vi "Loop_Auto.vi"() -> ()   [LabVIEW 2017, in "Autonomous.lvlib"]
uses:
  Autonomous.lvlib
  ENUM_Auto_State.ctl
  TypeDef/CLUSTER_CMD_WC_Drive.ctl
  TypeDef/ENUM_WC_Drive_DriveMode.ctl
  TypeDef/CLUSTER_Drive_ACT Loop_VBus Data.ctl
  TypeDef/CLUSTER_X and Y.ctl
  TypeDef/CLUSTER_Drive_ACT Loop_Profile Data.ctl
  ENUM_Auto_AutoMode.ctl
  TypeDef/CLUSTER_AUTO_switchBools.ctl
  Rotation_Overloard/CLUSTER_Rotation_CMD.ctl
  Rotation_Overloard/ENUM_Rotation_Positon.ctl
  <vilib>/Rock Robotics/WPI/ThirdParty/Sensors/navX/_TypeDefs/FRIC_navX_DeviceNumbersTypeDef.ctl
  ENUM_Auto_Action.ctl
  _SHARE ALL/Global Share All/Global_STOP.vi
  Globals/Global_Drive_Encoders.vi
  Rotation_Overloard/Global_CMD.vi
  Rotation_Overloard/Global_SM_Output.vi
  <vilib>/addons/control/pid/pid.llb/PID (DBL).vi
  Globals/Global_CMD_Drive.vi
  Rotation_Overloard/Rotation_Overlord.lvlib
  <vilib>/addons/control/pid/NI_PID_pid.lvlib
panel:
  in  "Enum":enum16{"LRL", "RLR", "RRR", "LLL"}(ring)
  out "Yaw":dbl
  out "Cycle Time (S)":dbl format="%.3g"
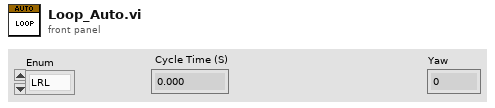
[diagram p1: front panel]
types:
  T1 = typedef "Rotation_Overlord.lvlib/ENUM_Rotation_Positon.ctl" = enum16{"Neutral", "Pickup", "Switch", "Scale", "Climb", "Manual"}
  T2 = typedef "Rotation_Overlord.lvlib/CLUSTER_Rotation_CMD.ctl" = cluster{"Rotation Positon":T1, "Enable Rotation":bool, "Manual Override":bool, "Arm Value":dbl, "Claw Rotation Value":dbl, "Lift Value":dbl}
  T3 = typedef "CLUSTER_AUTO_switchBools.ctl" = cluster{"First Drive":bool, "Rotated ":bool, "Second Move":bool, "Arm In position":bool, "Cube released":bool}
  T4 = typedef "ENUM_Auto_AutoMode.ctl" = enum16{"No Movement", "Scale And Switch", "Switch", "Scale", "Cross Line"}
  T5 = typedef "CLUSTER_CMD_WC_Drive.ctl" = cluster{"Drive_Mode":T6, "VBus":T7, "Profile":T9, "Zero Drive Encoders":bool, "Set Target Position(IN)":dbl, "Target Angle(Degree)":dbl, "Lock Angle":bool, "Zero YAW":bool, "Follow Cubes":bool, "Follow Road":bool, "Anti-Turbo":bool}
  T6 = typedef "ENUM_WC_Drive_DriveMode.ctl" = enum16{"Motion Profile", "CrossLineAuto", "VBus", "Stop"}
  T7 = typedef "CLUSTER_Drive_ACT Loop_VBus Data.ctl" = cluster{"Drive":T8, "Turbo":bool}
  T8 = typedef "CLUSTER_X and Y.ctl" = cluster{"Steer":dbl, "Throtle":dbl}
  T9 = typedef "CLUSTER_Drive_ACT Loop_Profile Data.ctl" = cluster{"Start":bool}
  T10 = typedef "Autonomous.lvlib/ENUM_Auto_State.ctl" = enum16{"Startup", "Idle", "position claw arm lift", "Intake", "Rotate To Angle", "Cross Line", "Shutdown"}
  T11 = typedef "Autonomous.lvlib/ENUM_Auto_Action.ctl" = enum16{"No Action", "Reset Time", "Reset All", "Lock Angle", "Drive", "Zero Drive Encoders", "Zero YAW"}
  T12 = cluster{"State":T10, "Previous State":T10, "Current Time":timestamp, "Previous Time":timestamp, "Start Time":timestamp, "Target Time (ms)":u32, "Cycle Time(S)":dbl, "CMD_Drive_Data":T5, "Test":dbl, "Steering":dbl, "Throtal":dbl, "Encoder Target Position(in)":dbl, "Zero Drive Encoders":bool, "Lock Angle":bool, "Target Angle(Degree)":dbl, "Zero YAW":bool, "Left Encoder":i32, "Right Encoder":i32, "YAW":dbl, "AutoMode":T4, "Switch Booleans":T3, "CMD_SM_Rotation":T2, "SM_Rotation_Output":T1}
  T13 = typedef "FRIC_navX_DeviceNumbersTypeDef.ctl" = enum16{"Dev0", "Dev1", "Dev2", "Dev3"}
  T14 = cluster{"proportional gain (Kc)":dbl, "integral time (Ti, min)":dbl, "derivative time (Td, min)":dbl}
  T15 = cluster{"Left_Drive_Encoder":i32, "Right_Drive_Encoder":i32}
  T16 = cluster{"Rollover":dbl, "Yaw":dbl, "Cont Yaw":dbl}
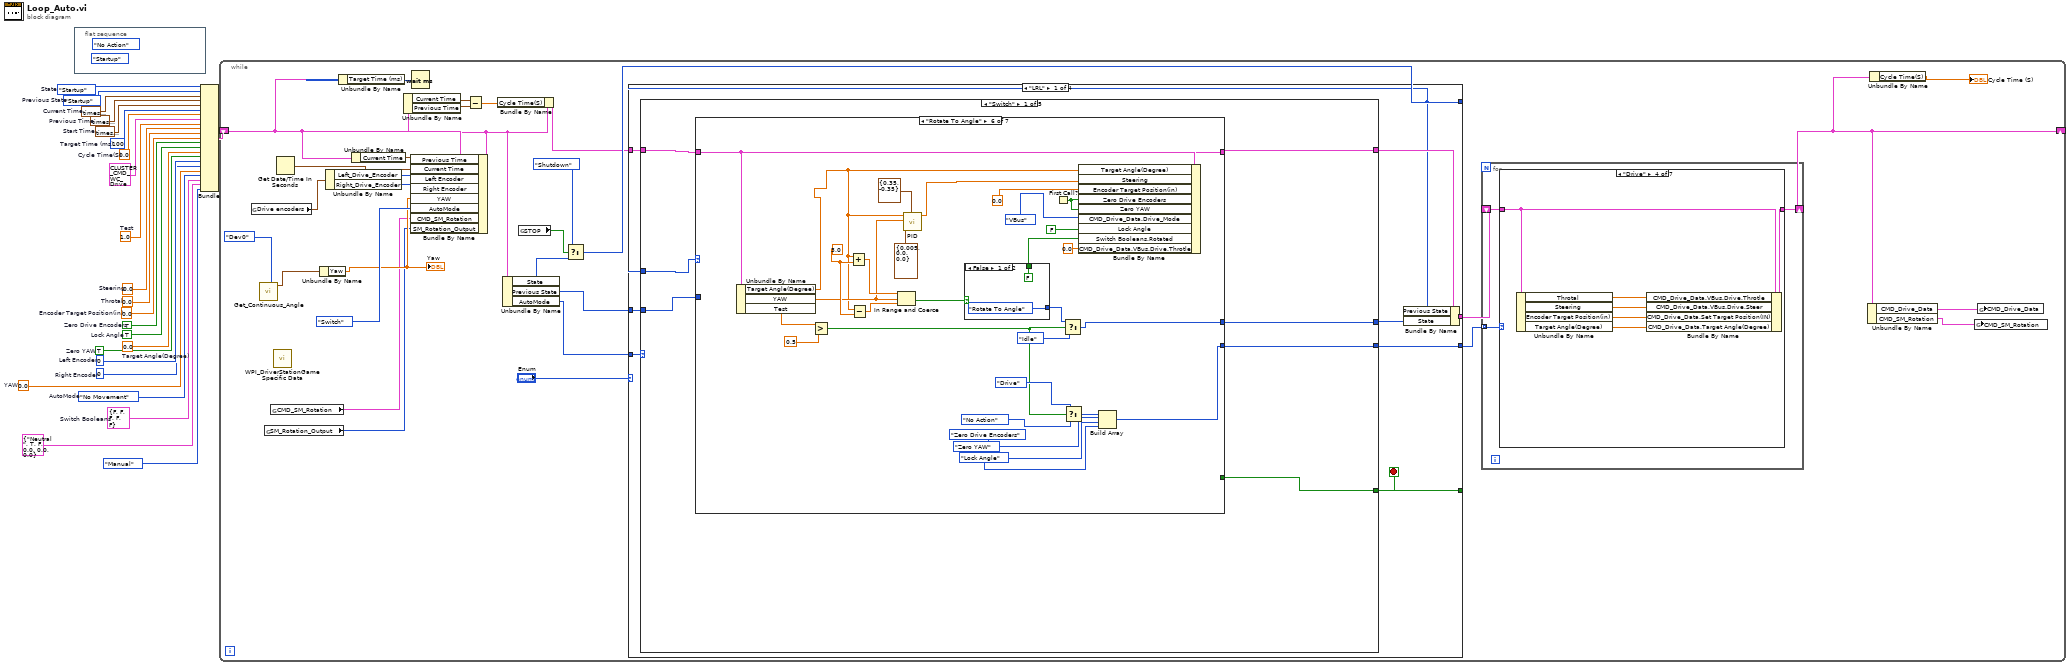
[diagram p0: block diagram]
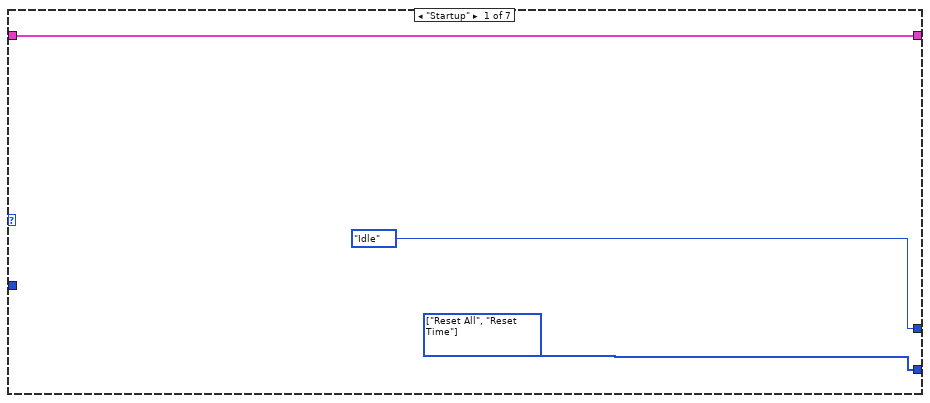
[diagram p2: hidden frame]
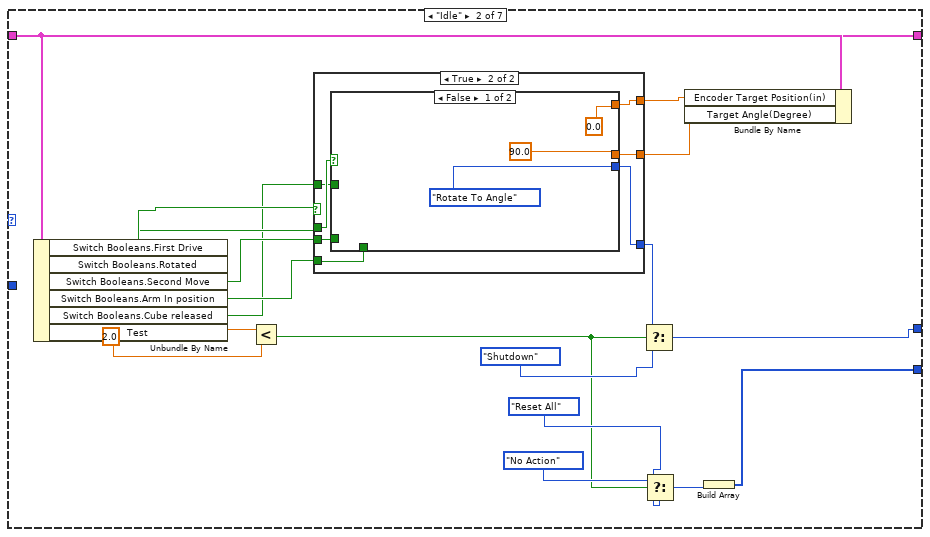
[diagram p3: hidden frame]
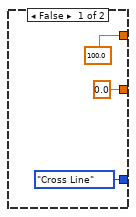
[diagram p4: hidden frame]
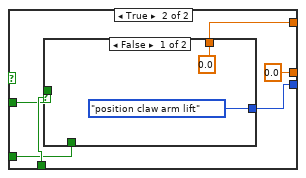
[diagram p5: hidden frame]
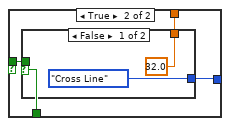
[diagram p6: hidden frame]
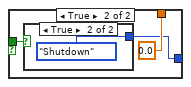
[diagram p7: hidden frame]
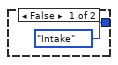
[diagram p8: hidden frame]
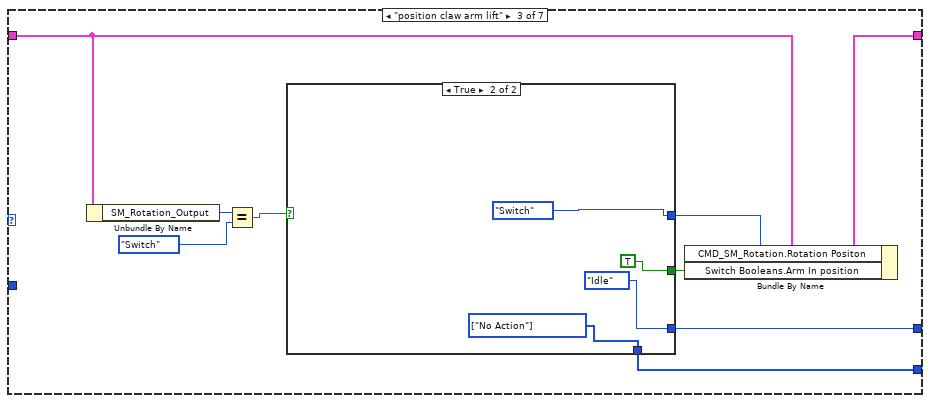
[diagram p9: hidden frame]
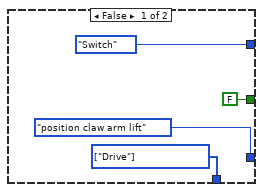
[diagram p10: hidden frame]
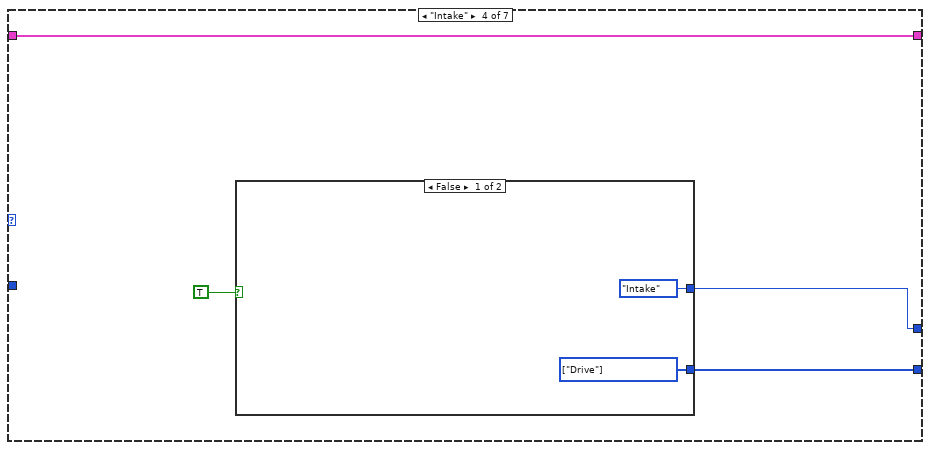
[diagram p11: hidden frame]
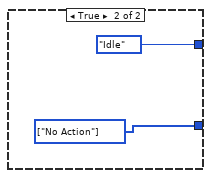
[diagram p12: hidden frame]
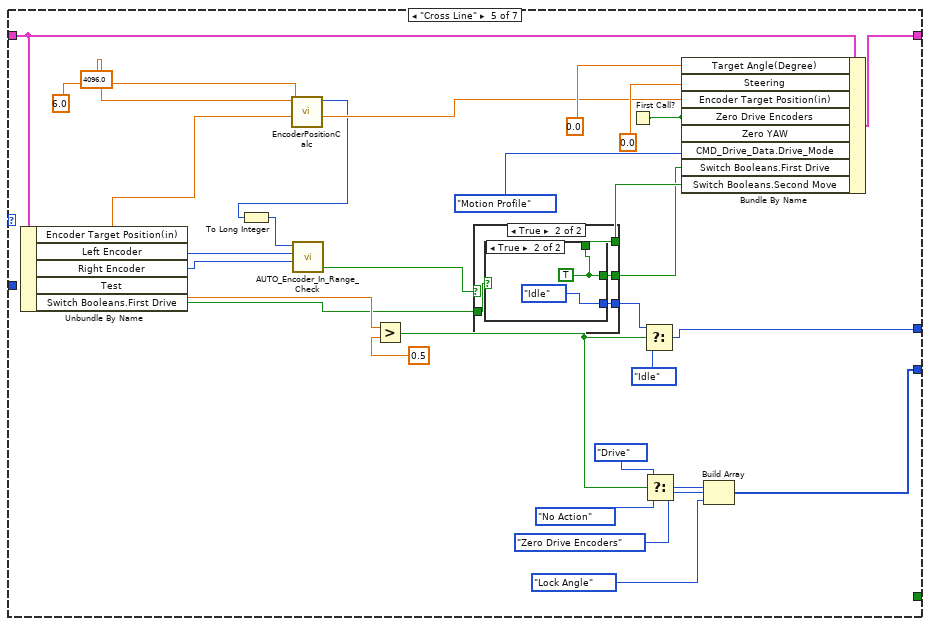
[diagram p13: hidden frame]
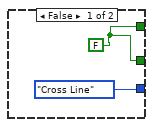
[diagram p14: hidden frame]
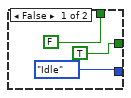
[diagram p15: hidden frame]
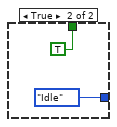
[diagram p16: hidden frame]
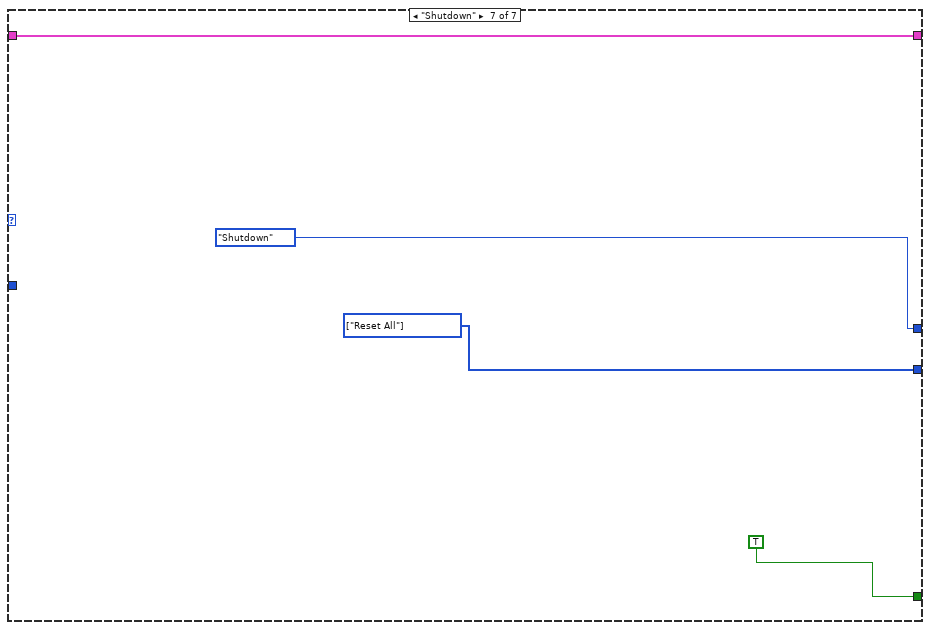
[diagram p17: hidden frame]
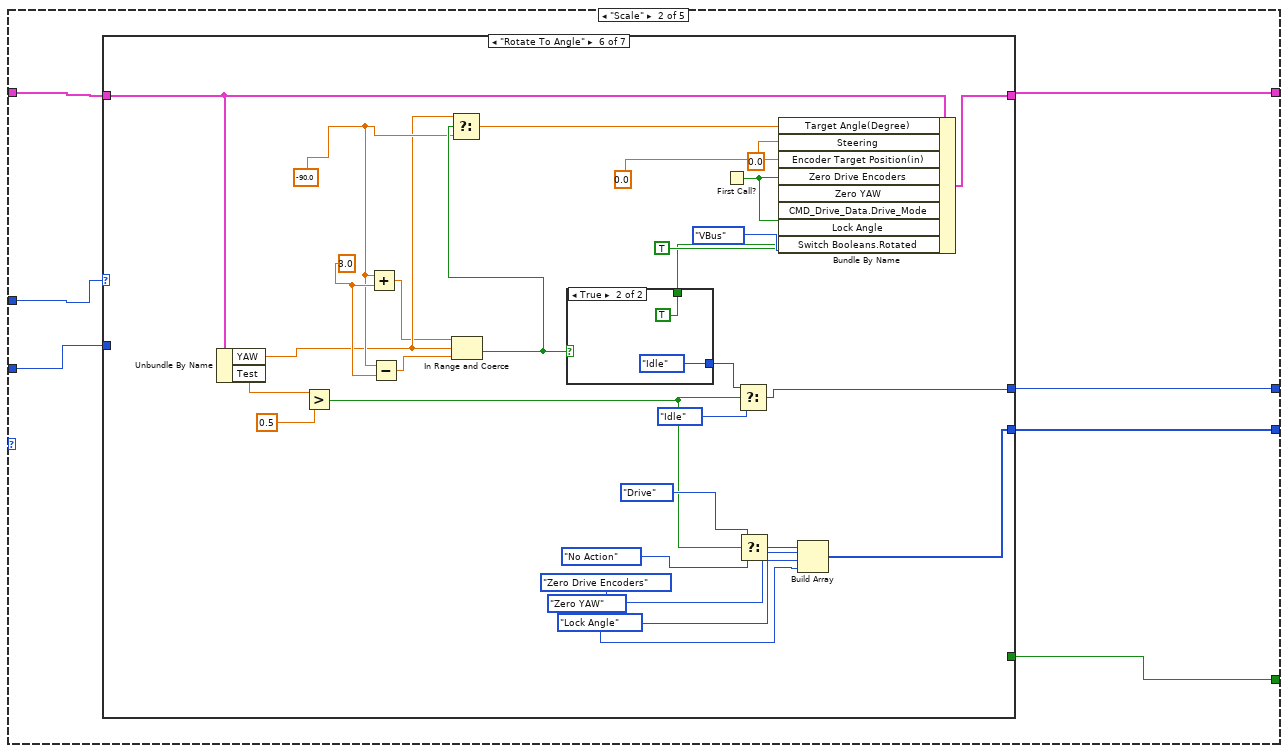
[diagram p18: hidden frame]
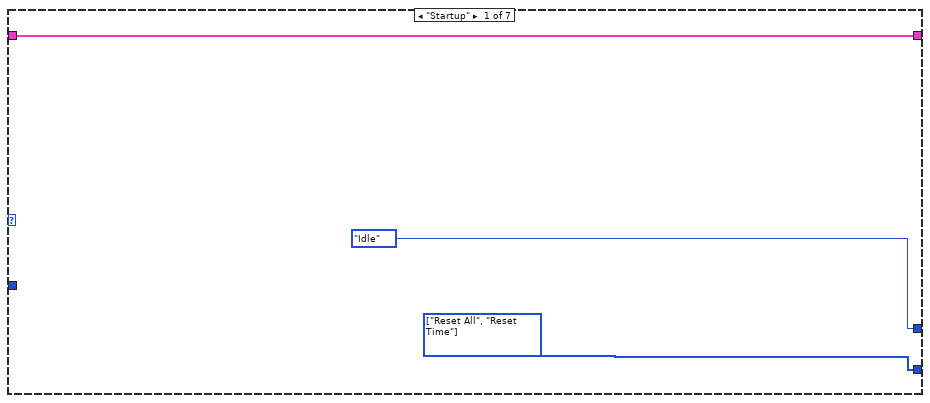
[diagram p19: hidden frame]
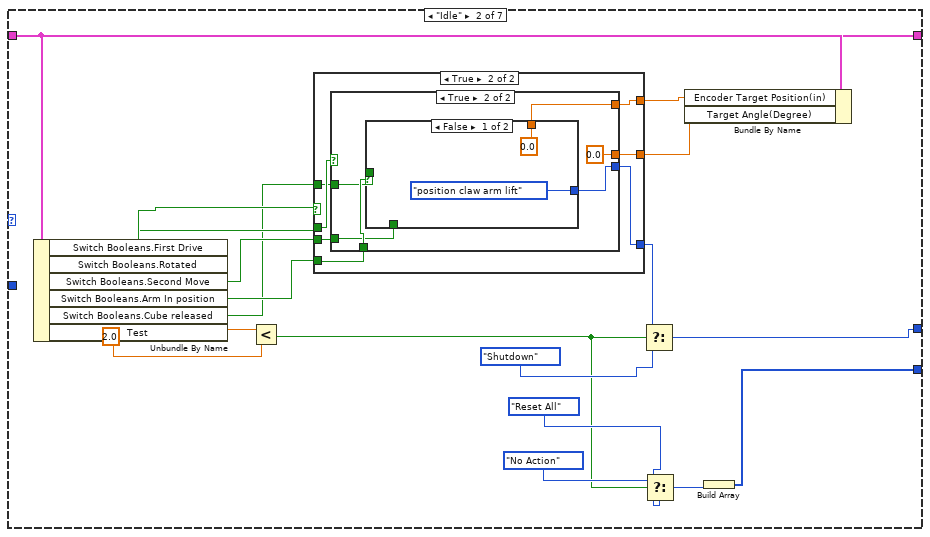
[diagram p20: hidden frame]
diagram:
  w3 = T3 {"First Drive"=FALSE, "Rotated "=FALSE, "Second Move"=FALSE, "Arm In position"=FALSE, "Cube released"=FALSE}  # Switch Booleans
  w4 = ENUM_Auto_AutoMode."No Movement"  # AutoMode
  w5 = 0.0  # YAW
  w6 = 0  # Right Encoder
  w7 = 0  # Left Encoder
  w8 = TRUE  # Zero YAW
  w9 = 0.0  # Target Angle(Degree)
  w10 = TRUE  # Lock Angle
  w11 = TRUE  # Zero Drive Encoders
  w12 = 0.0  # Encoder Target Position(in)
  w13 = 0.0  # Throtal
  w14 = 0.0  # Steering
  w15 = 1.0  # Test
  w17 = 0.0  # Cycle Time(S)
  w18 = ENUM_Auto_State."Startup"  # Previous State
  w19 = timestamp(0 s since 1904-01-01)  # Previous Time
  w20 = u32 100  # Target Time (ms)
  w21 = timestamp(0 s since 1904-01-01)  # Start Time
  w22 = timestamp(0 s since 1904-01-01)  # Current Time
  w23 = ENUM_Auto_State."Startup"  # State
  n1 = flat-sequence {
    frame #0 {
      (unwired) ENUM_Auto_State."Startup" ("State")
      (unwired) ENUM_Auto_Action."No Action" ("Action")
    }
  }
  n2 = Bundle("State"=w23, "Previous State"=w18, "Current Time"=w22, "Previous Time"=w19, "Start Time"=w21, "Target Time (ms)"=w20, "Cycle Time(S)"=w17, "CMD_Drive_Data"=T5 {"Drive_Mode"=enum."Motion Profile", "VBus"={"Drive"={"Steer"=0.0, "Throtle"=0.0}, "Turbo"=FALSE}, "Profile"={"Start"=FALSE}, "Zero Drive Encoders"=FALSE, "Set Target Position(IN)"=0.0, "Target Angle(Degree)"=0.0, "Lock Angle"=FALSE, "Zero YAW"=FALSE, "Follow Cubes"=FALSE, "Follow Road"=FALSE, "Anti-Turbo"=FALSE}, "Test"=w15, "Steering"=w14, "Throtal"=w13, "Encoder Target Position(in)"=w12, "Zero Drive Encoders"=w11, "Lock Angle"=w10, "Target Angle(Degree)"=w9, "Zero YAW"=w8, "Left Encoder"=w7, "Right Encoder"=w6, "YAW"=w5, "AutoMode"=w4, "Switch Booleans"=w3, "CMD_SM_Rotation"=T2 {"Rotation Positon"=enum."Neutral", "Enable Rotation"=TRUE, "Manual Override"=FALSE, "Arm Value"=0.0, "Claw Rotation Value"=0.0, "Lift Value"=0.0}, "SM_Rotation_Output"=ENUM_Rotation_Positon."Manual") -> (w24:T12)  [unwired: 1 in]
  n3 = while {
    shift-right: [w46] -> _
    shift-left: w24 -> [w49]
    stop <- w38 stop-if-true
    n4 = global read "Global_Drive_Encoders.vi" "Drive encoders"() -> (w31:T15)
    n5 = call <vilib>:"Get_Continuous_Angle.vi"("Device Number"=FRIC_navX_DeviceNumbersTypeDef."Dev0") -> ("Continuous Angle"=w33:T16)  [unwired: 10 in]
    n6 = global read "Global_SM_Output.vi" "SM_Rotation_Output"() -> (w27:T1)
    n7 = global read "Global_CMD.vi" "CMD_SM_Rotation"() -> (w28:T2)
    n8 = call <vilib>:"WPI_DriverStationGame Specific Data.vi"() -> ()  [unwired: 11 in, 1 out]
    n9 = Get Date/Time In Seconds() -> (seconds since 1Jan1904=w56:timestamp)
    n10 = Unbundle By Name(w33) -> ("Yaw"=w32:dbl)
    "Yaw" <- w32
    n11 = Unbundle By Name(w31) -> ("Left_Drive_Encoder"=w30:i32, "Right_Drive_Encoder"=w29:i32)
    n12 = Unbundle By Name(w49) -> ("Target Time (ms)"=w51:u32)
    n13 = Unbundle By Name(w49) -> ("Current Time"=w50:timestamp)
    n14 = Bundle By Name(cluster=w49, "Previous Time"=w50, "Current Time"=w56, "Left Encoder"=w30, "Right Encoder"=w29, "YAW"=w32, "AutoMode"=ENUM_Auto_AutoMode."Switch", "CMD_SM_Rotation"=w28, "SM_Rotation_Output"=w27) -> (w42:T12)
    n15 = Unbundle By Name(w42) -> ("Current Time"=w43:timestamp, "Previous Time"=w44:timestamp)
    n16 = Wait (ms)(milliseconds to wait=w51) -> ()  [unwired: 1 out]
    n17 = Subtract(x=w43, y=w44) -> (x-y=w40:dbl)
    n18 = Bundle By Name(cluster=w42, "Cycle Time(S)"=w40) -> (w41:T12)
    n19 = Unbundle By Name(w42) -> ("State"=w52:T10, "Previous State"=w48:T10, "AutoMode"=w36:T4)
    n20 = global read "Global_STOP.vi" "STOP"() -> (w54:bool)
    n21 = Select(t=ENUM_Auto_State."Shutdown" ("State"), s=w54, f=w52) -> (s? t:f=w47:T10)
    n22 = case shown="\"LRL\"" "Enum" {
      tunnel: [w65 w692 w1318 w1942] -> w55
      tunnel: w48 -> [w62 w689 w1315 w1939]
      tunnel: w47 -> [w61 w688 w1314 w1938]
      tunnel: w41 -> [w60 w687 w1313 w1937]
      tunnel: [w59 w686 w1312 w1936] -> w39
      tunnel: [w58 w685 w1311 w1935] -> w38
      tunnel: w36 -> [w57 w684 w1310 w1934]
      frame "LRL" {
        n23 = case shown="\"Switch\"" w57 {
          tunnel: [w72 w236 w397 w558 w651] -> w64
          tunnel: [w66 w230 w391 w557 w650] -> w63
          tunnel: w62 -> [w71 w235 w396 w556 w649]
          tunnel: w61 -> [w70 w234 w395 w555 w648]
          tunnel: w60 -> [w69 w233 w394 w554 w647]
          tunnel: [w67 w231 w392 w553 w646] -> w59
          tunnel: [w68 w232 w393 w552 w645] -> w58
          frame "Switch" {
            n24 = case shown="\"Rotate To Angle\"" w70 {
              tunnel: w69 -> [w75 w81 w132 w147 w173 w214 w229]
              tunnel: [w75 w80 w131 w147 w172 w213 w229] -> w72
              tunnel: w71 -> [_ _ _ _ _ _ _]
              tunnel: [_ _ _ _ _ _ TRUE] -> w68
              tunnel: [ENUM_Auto_State."Idle" ("State") w76 w129 w145 w159 w200 ENUM_Auto_State."Shutdown" ("State")] -> w66
              tunnel: [w73 w77 w127 w146 w158 w199 w226] -> w67
              frame "Startup" {
                w73 = T11[] [enum."Reset All", enum."Reset Time"] items=["No Action", "Reset Time", "Reset All", "Lock Angle", "Drive", "Zero Drive Encoders", "Zero YAW"] ("Actions")
              }
              frame "Idle" {
                n25 = Unbundle By Name(w81) -> ("Switch Booleans.First Drive"=w86:bool, "Switch Booleans.Rotated"=w85:bool, "Switch Booleans.Second Move"=w84:bool, "Switch Booleans.Arm In position"=w83:bool, "Switch Booleans.Cube released"=w82:bool, "Test"=w88:dbl)
                n26 = Less?(x=w88, y=2.0) -> (x < y?=w90:bool)
                n27 = case shown="True" w86 {
                  tunnel: [ENUM_Auto_State."Cross Line" ("State") w103] -> w94
                  tunnel: w85 -> [_ w104]
                  tunnel: w84 -> [_ w102]
                  tunnel: w83 -> [_ w101]
                  tunnel: w82 -> [_ w100]
                  tunnel: [100.0 w98] -> w79
                  tunnel: [0.0 w99] -> w78
                  frame False {
                  }
                  frame True {
                    n28 = case shown="False" w104 {
                      tunnel: [ENUM_Auto_State."Rotate To Angle" ("State") w111] -> w103
                      tunnel: w102 -> [_ w110]
                      tunnel: w101 -> [_ w112]
                      tunnel: w100 -> [_ w108]
                      tunnel: [90.0 0.0] -> w99
                      tunnel: [0.0 w109] -> w98
                      frame False {
                      }
                      frame True {
                        n29 = case shown="False" w112 {
                          tunnel: [ENUM_Auto_State."position claw arm lift" ("State") w118] -> w111
                          tunnel: w110 -> [_ w119]
                          tunnel: [0.0 w117] -> w109
                          tunnel: w108 -> [_ w116]
                          frame False {
                          }
                          frame True {
                            n30 = case shown="False" w119 {
                              tunnel: [ENUM_Auto_State."Cross Line" ("State") w123] -> w118
                              tunnel: [32.0 0.0] -> w117
                              tunnel: w116 -> [_ w122]
                              frame False {
                              }
                              frame True {
                                n31 = case shown="True" w122 {
                                tunnel: [ENUM_Auto_State."Intake" ("State") ENUM_Auto_State."Shutdown" ("State")] -> w123
                                frame False {
                                }
                                frame True {
                                }
                                }
                              }
                            }
                          }
                        }
                      }
                    }
                  }
                }
                n32 = Select(t=w94, s=w90, f=ENUM_Auto_State."Shutdown" ("State")) -> (s? t:f=w76:T10)
                n33 = Select(t=ENUM_Auto_Action."Reset All" ("Action"), s=w90, f=ENUM_Auto_Action."No Action" ("Action")) -> (s? t:f=w89:T11)
                n34 = Bundle By Name(cluster=w81, "Encoder Target Position(in)"=w79, "Target Angle(Degree)"=w78) -> (w80:T12)
                n35 = Build Array(w89) -> (w77:T11[])
              }
              frame "position claw arm lift" {
                n36 = Unbundle By Name(w132) -> ("SM_Rotation_Output"=w135:T1)
                n37 = Equal?(x=w135, y=ENUM_Rotation_Positon."Switch" ("CMD_SM_Rotation.Rotation Positon")) -> (x = y?=w133:bool)
                n38 = case shown="True" w133 {
                  tunnel: [ENUM_Rotation_Positon."Switch" ("CMD_SM_Rotation.Rotation Positon") ENUM_Rotation_Positon."Switch" ("CMD_SM_Rotation.Rotation Positon")] -> w130
                  tunnel: [ENUM_Auto_State."position claw arm lift" ("State") ENUM_Auto_State."Idle" ("State")] -> w129
                  tunnel: [FALSE ("Switch Booleans.Arm In position") TRUE ("Switch Booleans.Arm In position")] -> w128
                  tunnel: [w136 w140] -> w127
                  frame False {
                    w136 = T11[] [enum."Drive"] items=["No Action", "Reset Time", "Reset All", "Lock Angle", "Drive", "Zero Drive Encoders", "Zero YAW"] ("Actions")
                  }
                  frame True {
                    w140 = T11[] [enum."No Action"] items=["No Action", "Reset Time", "Reset All", "Lock Angle", "Drive", "Zero Drive Encoders", "Zero YAW"] ("Actions")
                  }
                }
                n39 = Bundle By Name(cluster=w132, "CMD_SM_Rotation.Rotation Positon"=w130, "Switch Booleans.Arm In position"=w128) -> (w131:T12)
              }
              frame "Intake" {
                n40 = case shown="False" TRUE {
                  tunnel: [ENUM_Auto_State."Intake" ("State") ENUM_Auto_State."Idle" ("State")] -> w145
                  tunnel: [w148 w150] -> w146
                  frame False {
                    w148 = T11[] [enum."Drive"] items=["No Action", "Reset Time", "Reset All", "Lock Angle", "Drive", "Zero Drive Encoders", "Zero YAW"] ("Actions")
                  }
                  frame True {
                    w150 = T11[] [enum."No Action"] items=["No Action", "Reset Time", "Reset All", "Lock Angle", "Drive", "Zero Drive Encoders", "Zero YAW"] ("Actions")
                  }
                }
              }
              frame "Cross Line" {
                n41 = Unbundle By Name(w173) -> ("Encoder Target Position(in)"=w155:dbl, "Left Encoder"=w157:i32, "Right Encoder"=w156:i32, "Test"=w175:dbl, "Switch Booleans.First Drive"=w164:bool)
                n42 = call "EncoderPositionCalc.vi"("PositionTarget(in)"=w155, "Wheel Size(in)"=6.0, "EncoderCount/Revolution"=4096.0) -> ("PostionTarget(Counts)"=w152:i32)  [unwired: 8 in]
                n43 = To Long Integer(number=w152) -> (32bit integer=w153:i32)
                n44 = call "AUTO_Encoder_In_Range_Check.vi"("Right Encoder"=w156, "Left Encoder"=w157, "PostionTarget(Counts)"=w153) -> ("Boolean"=w166:bool)  [unwired: 8 in]
                n45 = Greater?(x=w175, y=0.5) -> (0:w177:bool)
                n46 = case shown="True" w166 {
                  tunnel: [ENUM_Auto_State."Cross Line" ("State") w186] -> w167
                  tunnel: w164 -> [_ w185]
                  tunnel: [w181 w184] -> w163
                  tunnel: [w181 w183] -> w162
                  frame False {
                    w181 = FALSE
                  }
                  frame True {
                    n47 = case shown="True" w185 {
                      tunnel: [ENUM_Auto_State."Idle" ("State") ENUM_Auto_State."Idle" ("State")] -> w186
                      tunnel: [FALSE w190] -> w184
                      tunnel: [TRUE w190] -> w183
                      frame False {
                      }
                      frame True {
                        w190 = TRUE
                      }
                    }
                  }
                }
                n48 = First Call?() -> (First Call?: T/F=w154:bool)
                n49 = Select(t=w167, s=w177, f=ENUM_Auto_State."Idle" ("State")) -> (s? t:f=w159:T10)
                n50 = Select(t=ENUM_Auto_Action."Drive" ("Action"), s=w177, f=ENUM_Auto_Action."No Action" ("Action")) -> (s? t:f=w176:T11)
                n51 = Bundle By Name(cluster=w173, "Target Angle(Degree)"=0.0, "Steering"=0.0, "Encoder Target Position(in)"=w155, "Zero Drive Encoders"=w154, "Zero YAW"=w154, "CMD_Drive_Data.Drive_Mode"=ENUM_WC_Drive_DriveMode."Motion Profile", "Switch Booleans.First Drive"=w162, "Switch Booleans.Second Move"=w163) -> (w172:T12)
                n52 = Build Array(w176, ENUM_Auto_Action."Zero Drive Encoders" ("Action"), ENUM_Auto_Action."Lock Angle" ("Action")) -> (w158:T11[])
              }
              frame "Rotate To Angle" {
                w206 = 3.0 ("y")
                n53 = Unbundle By Name(w214) -> ("Target Angle(Degree)"=w194:dbl, "YAW"=w195:dbl, "Test"=w216:dbl)
                n54 = Greater?(x=w216, y=0.5) -> (0:w218:bool)
                n55 = Add(x=w194, y=w206) -> (x+y=w202:dbl)
                n56 = Subtract(x=w194, y=w206) -> (x-y=w201:dbl)
                n57 = In Range and Coerce(upper limit=w202, x=w195, lower limit=w201) -> (In Range?=w204:bool)  [unwired: 1 out]
                n58 = call-poly <vilib>:"PID.vi"("output range"=cluster{"output high":dbl, "output low":dbl} {"output high"=0.35, "output low"=-0.35}, "PID gains"=T14 {"proportional gain (Kc)"=0.005, "integral time (Ti, min)"=0.0, "derivative time (Td, min)"=0.0}, "process variable"=w195, "setpoint"=w194) -> ("output"=w193:dbl)  [unwired: 6 in, 1 out]
                n59 = case shown="False" w204 {
                  tunnel: [ENUM_Auto_State."Rotate To Angle" ("State") ENUM_Auto_State."Idle" ("State")] -> w208
                  tunnel: [FALSE ("Lock Angle") TRUE ("Lock Angle")] -> w203
                  frame False {
                  }
                  frame True {
                  }
                }
                n60 = First Call?() -> (First Call?: T/F=w198:bool)
                n61 = Select(t=w208, s=w218, f=ENUM_Auto_State."Idle" ("State")) -> (s? t:f=w200:T10)
                n62 = Select(t=ENUM_Auto_Action."Drive" ("Action"), s=w218, f=ENUM_Auto_Action."No Action" ("Action")) -> (s? t:f=w217:T11)
                n63 = Bundle By Name(cluster=w214, "Target Angle(Degree)"=w194, "Steering"=w193, "Encoder Target Position(in)"=0.0, "Zero Drive Encoders"=w198, "Zero YAW"=w198, "CMD_Drive_Data.Drive_Mode"=ENUM_WC_Drive_DriveMode."VBus", "Lock Angle"=FALSE, "Switch Booleans.Rotated"=w203, "CMD_Drive_Data.VBus.Drive.Throtle"=0.0) -> (w213:T12)
                n64 = Build Array(w217, ENUM_Auto_Action."Zero Drive Encoders" ("Action"), ENUM_Auto_Action."Zero YAW" ("Action"), ENUM_Auto_Action."Lock Angle" ("Action")) -> (w199:T11[])
              }
              frame "Shutdown" {
                w226 = T11[] [enum."Reset All"] items=["No Action", "Reset Time", "Reset All", "Lock Angle", "Drive", "Zero Drive Encoders", "Zero YAW"] ("Actions")
              }
            }
          }
          frame "Scale" {
            n65 = case shown="\"Rotate To Angle\"" w234 {
              tunnel: w233 -> [w239 w245 w296 w311 w336 w375 w390]
              tunnel: [w239 w244 w295 w311 w335 w374 w390] -> w236
              tunnel: w235 -> [_ _ _ _ _ _ _]
              tunnel: [_ _ _ _ _ _ TRUE] -> w232
              tunnel: [ENUM_Auto_State."Idle" ("State") w240 w293 w309 w317 w356 ENUM_Auto_State."Shutdown" ("State")] -> w230
              tunnel: [w237 w241 w291 w310 w316 w355 w387] -> w231
              frame "Startup" {
                w237 = T11[] [enum."Reset All", enum."Reset Time"] items=["No Action", "Reset Time", "Reset All", "Lock Angle", "Drive", "Zero Drive Encoders", "Zero YAW"] ("Actions")
              }
              frame "Idle" {
                n66 = Unbundle By Name(w245) -> ("Switch Booleans.First Drive"=w250:bool, "Switch Booleans.Rotated"=w249:bool, "Switch Booleans.Second Move"=w248:bool, "Switch Booleans.Arm In position"=w247:bool, "Switch Booleans.Cube released"=w246:bool, "Test"=w252:dbl)
                n67 = Less?(x=w252, y=2.0) -> (x < y?=w254:bool)
                n68 = case shown="True" w250 {
                  tunnel: [ENUM_Auto_State."Cross Line" ("State") w267] -> w258
                  tunnel: w249 -> [_ w268]
                  tunnel: w248 -> [_ w266]
                  tunnel: w247 -> [_ w265]
                  tunnel: w246 -> [_ w264]
                  tunnel: [94.0 w262] -> w243
                  tunnel: [0.0 w263] -> w242
                  frame False {
                  }
                  frame True {
                    n69 = case shown="True" w268 {
                      tunnel: [ENUM_Auto_State."Rotate To Angle" ("State") w275] -> w267
                      tunnel: w266 -> [_ w274]
                      tunnel: w265 -> [_ w276]
                      tunnel: w264 -> [_ w272]
                      tunnel: [90.0 0.0] -> w263
                      tunnel: [0.0 w273] -> w262
                      frame False {
                      }
                      frame True {
                        n70 = case shown="False" w276 {
                          tunnel: [ENUM_Auto_State."position claw arm lift" ("State") w282] -> w275
                          tunnel: w274 -> [_ w283]
                          tunnel: [0.0 w281] -> w273
                          tunnel: w272 -> [_ w280]
                          frame False {
                          }
                          frame True {
                            n71 = case shown="False" w283 {
                              tunnel: [ENUM_Auto_State."Cross Line" ("State") w287] -> w282
                              tunnel: [32.0 0.0] -> w281
                              tunnel: w280 -> [_ w286]
                              frame False {
                              }
                              frame True {
                                n72 = case shown="True" w286 {
                                tunnel: [ENUM_Auto_State."Intake" ("State") ENUM_Auto_State."Shutdown" ("State")] -> w287
                                frame False {
                                }
                                frame True {
                                }
                                }
                              }
                            }
                          }
                        }
                      }
                    }
                  }
                }
                n73 = Select(t=w258, s=w254, f=ENUM_Auto_State."Shutdown" ("State")) -> (s? t:f=w240:T10)
                n74 = Select(t=ENUM_Auto_Action."Reset All" ("Action"), s=w254, f=ENUM_Auto_Action."No Action" ("Action")) -> (s? t:f=w253:T11)
                n75 = Bundle By Name(cluster=w245, "Encoder Target Position(in)"=w243, "Target Angle(Degree)"=w242) -> (w244:T12)
                n76 = Build Array(w253) -> (w241:T11[])
              }
              frame "position claw arm lift" {
                n77 = Unbundle By Name(w296) -> ("SM_Rotation_Output"=w299:T1)
                n78 = Equal?(x=w299, y=ENUM_Rotation_Positon."Switch" ("CMD_SM_Rotation.Rotation Positon")) -> (x = y?=w297:bool)
                n79 = case shown="True" w297 {
                  tunnel: [ENUM_Rotation_Positon."Switch" ("CMD_SM_Rotation.Rotation Positon") ENUM_Rotation_Positon."Switch" ("CMD_SM_Rotation.Rotation Positon")] -> w294
                  tunnel: [ENUM_Auto_State."position claw arm lift" ("State") ENUM_Auto_State."Idle" ("State")] -> w293
                  tunnel: [FALSE ("Switch Booleans.Arm In position") TRUE ("Switch Booleans.Arm In position")] -> w292
                  tunnel: [w300 w304] -> w291
                  frame False {
                    w300 = T11[] [enum."Drive"] items=["No Action", "Reset Time", "Reset All", "Lock Angle", "Drive", "Zero Drive Encoders", "Zero YAW"] ("Actions")
                  }
                  frame True {
                    w304 = T11[] [enum."No Action"] items=["No Action", "Reset Time", "Reset All", "Lock Angle", "Drive", "Zero Drive Encoders", "Zero YAW"] ("Actions")
                  }
                }
                n80 = Bundle By Name(cluster=w296, "CMD_SM_Rotation.Rotation Positon"=w294, "Switch Booleans.Arm In position"=w292) -> (w295:T12)
              }
              frame "Intake" {
                n81 = case shown="False" TRUE {
                  tunnel: [ENUM_Auto_State."Intake" ("State") ENUM_Auto_State."Idle" ("State")] -> w309
                  tunnel: [w312 w314] -> w310
                  frame False {
                    w312 = T11[] [enum."Drive"] items=["No Action", "Reset Time", "Reset All", "Lock Angle", "Drive", "Zero Drive Encoders", "Zero YAW"] ("Actions")
                  }
                  frame True {
                    w314 = T11[] [enum."No Action"] items=["No Action", "Reset Time", "Reset All", "Lock Angle", "Drive", "Zero Drive Encoders", "Zero YAW"] ("Actions")
                  }
                }
              }
              frame "Cross Line" {
                n82 = Unbundle By Name(w336) -> ("Encoder Target Position(in)"=w318:dbl, "Left Encoder"=w327:i32, "Right Encoder"=w326:i32, "Test"=w338:dbl, "Switch Booleans.First Drive"=w323:bool)
                n83 = call "EncoderPositionCalc.vi"("PositionTarget(in)"=w318, "Wheel Size(in)"=6.0, "EncoderCount/Revolution"=4096.0) -> ("PostionTarget(Counts)"=w325:i32)  [unwired: 8 in]
                n84 = call "AUTO_Encoder_In_Range_Check.vi"("Right Encoder"=w326, "Left Encoder"=w327, "PostionTarget(Counts)"=w325) -> ("Boolean"=w328:bool)  [unwired: 8 in]
                n85 = Greater?(x=w338, y=0.5) -> (0:w340:bool)
                n86 = case shown="False" w328 {
                  tunnel: [ENUM_Auto_State."Cross Line" ("State") w349] -> w329
                  tunnel: w323 -> [_ w348]
                  tunnel: [w344 w347] -> w322
                  tunnel: [w344 w346] -> w321
                  frame False {
                    w344 = FALSE
                  }
                  frame True {
                    n87 = case shown="False" w348 {
                      tunnel: [ENUM_Auto_State."Idle" ("State") ENUM_Auto_State."Idle" ("State")] -> w349
                      tunnel: [FALSE w353] -> w347
                      tunnel: [TRUE w353] -> w346
                      frame False {
                      }
                      frame True {
                        w353 = TRUE
                      }
                    }
                  }
                }
                n88 = First Call?() -> (First Call?: T/F=w331:bool)
                n89 = Select(t=w329, s=w340, f=ENUM_Auto_State."Idle" ("State")) -> (s? t:f=w317:T10)
                n90 = Select(t=ENUM_Auto_Action."Drive" ("Action"), s=w340, f=ENUM_Auto_Action."No Action" ("Action")) -> (s? t:f=w339:T11)
                n91 = Bundle By Name(cluster=w336, "Target Angle(Degree)"=0.0, "Steering"=0.0, "Encoder Target Position(in)"=w318, "Zero Drive Encoders"=w331, "Zero YAW"=w331, "CMD_Drive_Data.Drive_Mode"=ENUM_WC_Drive_DriveMode."Motion Profile", "Switch Booleans.First Drive"=w321, "Switch Booleans.Second Move"=w322) -> (w335:T12)
                n92 = Build Array(w339, ENUM_Auto_Action."Zero Drive Encoders" ("Action"), ENUM_Auto_Action."Lock Angle" ("Action")) -> (w316:T11[])
              }
              frame "Rotate To Angle" {
                w366 = 3.0 ("y")
                w362 = -90.0 ("Target Angle(Degree)")
                n93 = Unbundle By Name(w375) -> ("YAW"=w361:dbl, "Test"=w377:dbl)
                n94 = Greater?(x=w377, y=0.5) -> (0:w379:bool)
                n95 = Add(x=w362, y=w366) -> (x+y=w358:dbl)
                n96 = Subtract(x=w362, y=w366) -> (x-y=w357:dbl)
                n97 = In Range and Coerce(upper limit=w358, x=w361, lower limit=w357) -> (In Range?=w363:bool)  [unwired: 1 out]
                n98 = Select(t=w361, s=w363, f=w362) -> (s? t:f=w364:dbl)
                n99 = case shown="True" w363 {
                  tunnel: [ENUM_Auto_State."Rotate To Angle" ("State") ENUM_Auto_State."Idle" ("State")] -> w368
                  tunnel: [FALSE ("Lock Angle") TRUE ("Lock Angle")] -> w359
                  frame False {
                  }
                  frame True {
                  }
                }
                n100 = First Call?() -> (First Call?: T/F=w372:bool)
                n101 = Select(t=w368, s=w379, f=ENUM_Auto_State."Idle" ("State")) -> (s? t:f=w356:T10)
                n102 = Select(t=ENUM_Auto_Action."Drive" ("Action"), s=w379, f=ENUM_Auto_Action."No Action" ("Action")) -> (s? t:f=w378:T11)
                n103 = Bundle By Name(cluster=w375, "Target Angle(Degree)"=w364, "Steering"=0.0, "Encoder Target Position(in)"=0.0, "Zero Drive Encoders"=w372, "Zero YAW"=w372, "CMD_Drive_Data.Drive_Mode"=ENUM_WC_Drive_DriveMode."VBus", "Lock Angle"=TRUE, "Switch Booleans.Rotated"=w359) -> (w374:T12)
                n104 = Build Array(w378, ENUM_Auto_Action."Zero Drive Encoders" ("Action"), ENUM_Auto_Action."Zero YAW" ("Action"), ENUM_Auto_Action."Lock Angle" ("Action")) -> (w355:T11[])
              }
              frame "Shutdown" {
                w387 = T11[] [enum."Reset All"] items=["No Action", "Reset Time", "Reset All", "Lock Angle", "Drive", "Zero Drive Encoders", "Zero YAW"] ("Actions")
              }
            }
          }
          frame "Scale And Switch" {
            n105 = case shown="\"Rotate To Angle\"" w395 {
              tunnel: w394 -> [w400 w406 w457 w472 w497 w536 w551]
              tunnel: [w400 w405 w456 w472 w496 w535 w551] -> w397
              tunnel: w396 -> [_ _ _ _ _ _ _]
              tunnel: [_ _ _ _ _ _ TRUE] -> w393
              tunnel: [ENUM_Auto_State."Idle" ("State") w401 w454 w470 w478 w517 ENUM_Auto_State."Shutdown" ("State")] -> w391
              tunnel: [w398 w402 w452 w471 w477 w516 w548] -> w392
              frame "Startup" {
                w398 = T11[] [enum."Reset All", enum."Reset Time"] items=["No Action", "Reset Time", "Reset All", "Lock Angle", "Drive", "Zero Drive Encoders", "Zero YAW"] ("Actions")
              }
              frame "Idle" {
                n106 = Unbundle By Name(w406) -> ("Switch Booleans.First Drive"=w411:bool, "Switch Booleans.Rotated"=w410:bool, "Switch Booleans.Second Move"=w409:bool, "Switch Booleans.Arm In position"=w408:bool, "Switch Booleans.Cube released"=w407:bool, "Test"=w413:dbl)
                n107 = Less?(x=w413, y=2.0) -> (x < y?=w415:bool)
                n108 = case shown="True" w411 {
                  tunnel: [ENUM_Auto_State."Cross Line" ("State") w428] -> w419
                  tunnel: w410 -> [_ w429]
                  tunnel: w409 -> [_ w427]
                  tunnel: w408 -> [_ w426]
                  tunnel: w407 -> [_ w425]
                  tunnel: [94.0 w423] -> w404
                  tunnel: [0.0 w424] -> w403
                  frame False {
                  }
                  frame True {
                    n109 = case shown="True" w429 {
                      tunnel: [ENUM_Auto_State."Rotate To Angle" ("State") w436] -> w428
                      tunnel: w427 -> [_ w435]
                      tunnel: w426 -> [_ w437]
                      tunnel: w425 -> [_ w433]
                      tunnel: [90.0 0.0] -> w424
                      tunnel: [0.0 w434] -> w423
                      frame False {
                      }
                      frame True {
                        n110 = case shown="False" w437 {
                          tunnel: [ENUM_Auto_State."position claw arm lift" ("State") w443] -> w436
                          tunnel: w435 -> [_ w444]
                          tunnel: [0.0 w442] -> w434
                          tunnel: w433 -> [_ w441]
                          frame False {
                          }
                          frame True {
                            n111 = case shown="False" w444 {
                              tunnel: [ENUM_Auto_State."Cross Line" ("State") w448] -> w443
                              tunnel: [32.0 0.0] -> w442
                              tunnel: w441 -> [_ w447]
                              frame False {
                              }
                              frame True {
                                n112 = case shown="True" w447 {
                                tunnel: [ENUM_Auto_State."Intake" ("State") ENUM_Auto_State."Shutdown" ("State")] -> w448
                                frame False {
                                }
                                frame True {
                                }
                                }
                              }
                            }
                          }
                        }
                      }
                    }
                  }
                }
                n113 = Select(t=w419, s=w415, f=ENUM_Auto_State."Shutdown" ("State")) -> (s? t:f=w401:T10)
                n114 = Select(t=ENUM_Auto_Action."Reset All" ("Action"), s=w415, f=ENUM_Auto_Action."No Action" ("Action")) -> (s? t:f=w414:T11)
                n115 = Bundle By Name(cluster=w406, "Encoder Target Position(in)"=w404, "Target Angle(Degree)"=w403) -> (w405:T12)
                n116 = Build Array(w414) -> (w402:T11[])
              }
              frame "position claw arm lift" {
                n117 = Unbundle By Name(w457) -> ("SM_Rotation_Output"=w460:T1)
                n118 = Equal?(x=w460, y=ENUM_Rotation_Positon."Switch" ("CMD_SM_Rotation.Rotation Positon")) -> (x = y?=w458:bool)
                n119 = case shown="True" w458 {
                  tunnel: [ENUM_Rotation_Positon."Switch" ("CMD_SM_Rotation.Rotation Positon") ENUM_Rotation_Positon."Switch" ("CMD_SM_Rotation.Rotation Positon")] -> w455
                  tunnel: [ENUM_Auto_State."position claw arm lift" ("State") ENUM_Auto_State."Idle" ("State")] -> w454
                  tunnel: [FALSE ("Switch Booleans.Arm In position") TRUE ("Switch Booleans.Arm In position")] -> w453
                  tunnel: [w461 w465] -> w452
                  frame False {
                    w461 = T11[] [enum."Drive"] items=["No Action", "Reset Time", "Reset All", "Lock Angle", "Drive", "Zero Drive Encoders", "Zero YAW"] ("Actions")
                  }
                  frame True {
                    w465 = T11[] [enum."No Action"] items=["No Action", "Reset Time", "Reset All", "Lock Angle", "Drive", "Zero Drive Encoders", "Zero YAW"] ("Actions")
                  }
                }
                n120 = Bundle By Name(cluster=w457, "CMD_SM_Rotation.Rotation Positon"=w455, "Switch Booleans.Arm In position"=w453) -> (w456:T12)
              }
              frame "Intake" {
                n121 = case shown="False" TRUE {
                  tunnel: [ENUM_Auto_State."Intake" ("State") ENUM_Auto_State."Idle" ("State")] -> w470
                  tunnel: [w473 w475] -> w471
                  frame False {
                    w473 = T11[] [enum."Drive"] items=["No Action", "Reset Time", "Reset All", "Lock Angle", "Drive", "Zero Drive Encoders", "Zero YAW"] ("Actions")
                  }
                  frame True {
                    w475 = T11[] [enum."No Action"] items=["No Action", "Reset Time", "Reset All", "Lock Angle", "Drive", "Zero Drive Encoders", "Zero YAW"] ("Actions")
                  }
                }
              }
              frame "Cross Line" {
                n122 = Unbundle By Name(w497) -> ("Encoder Target Position(in)"=w479:dbl, "Left Encoder"=w488:i32, "Right Encoder"=w487:i32, "Test"=w499:dbl, "Switch Booleans.First Drive"=w484:bool)
                n123 = call "EncoderPositionCalc.vi"("PositionTarget(in)"=w479, "Wheel Size(in)"=6.0, "EncoderCount/Revolution"=4096.0) -> ("PostionTarget(Counts)"=w486:i32)  [unwired: 8 in]
                n124 = call "AUTO_Encoder_In_Range_Check.vi"("Right Encoder"=w487, "Left Encoder"=w488, "PostionTarget(Counts)"=w486) -> ("Boolean"=w489:bool)  [unwired: 8 in]
                n125 = Greater?(x=w499, y=0.5) -> (0:w501:bool)
                n126 = case shown="False" w489 {
                  tunnel: [ENUM_Auto_State."Cross Line" ("State") w510] -> w490
                  tunnel: w484 -> [_ w509]
                  tunnel: [w505 w508] -> w483
                  tunnel: [w505 w507] -> w482
                  frame False {
                    w505 = FALSE
                  }
                  frame True {
                    n127 = case shown="False" w509 {
                      tunnel: [ENUM_Auto_State."Idle" ("State") ENUM_Auto_State."Idle" ("State")] -> w510
                      tunnel: [FALSE w514] -> w508
                      tunnel: [TRUE w514] -> w507
                      frame False {
                      }
                      frame True {
                        w514 = TRUE
                      }
                    }
                  }
                }
                n128 = First Call?() -> (First Call?: T/F=w492:bool)
                n129 = Select(t=w490, s=w501, f=ENUM_Auto_State."Idle" ("State")) -> (s? t:f=w478:T10)
                n130 = Select(t=ENUM_Auto_Action."Drive" ("Action"), s=w501, f=ENUM_Auto_Action."No Action" ("Action")) -> (s? t:f=w500:T11)
                n131 = Bundle By Name(cluster=w497, "Target Angle(Degree)"=0.0, "Steering"=0.0, "Encoder Target Position(in)"=w479, "Zero Drive Encoders"=w492, "Zero YAW"=w492, "CMD_Drive_Data.Drive_Mode"=ENUM_WC_Drive_DriveMode."Motion Profile", "Switch Booleans.First Drive"=w482, "Switch Booleans.Second Move"=w483) -> (w496:T12)
                n132 = Build Array(w500, ENUM_Auto_Action."Zero Drive Encoders" ("Action"), ENUM_Auto_Action."Lock Angle" ("Action")) -> (w477:T11[])
              }
              frame "Rotate To Angle" {
                w527 = 3.0 ("y")
                w523 = -90.0 ("Target Angle(Degree)")
                n133 = Unbundle By Name(w536) -> ("YAW"=w522:dbl, "Test"=w538:dbl)
                n134 = Greater?(x=w538, y=0.5) -> (0:w540:bool)
                n135 = Add(x=w523, y=w527) -> (x+y=w519:dbl)
                n136 = Subtract(x=w523, y=w527) -> (x-y=w518:dbl)
                n137 = In Range and Coerce(upper limit=w519, x=w522, lower limit=w518) -> (In Range?=w524:bool)  [unwired: 1 out]
                n138 = Select(t=w522, s=w524, f=w523) -> (s? t:f=w525:dbl)
                n139 = case shown="True" w524 {
                  tunnel: [ENUM_Auto_State."Rotate To Angle" ("State") ENUM_Auto_State."Idle" ("State")] -> w529
                  tunnel: [FALSE ("Lock Angle") TRUE ("Lock Angle")] -> w520
                  frame False {
                  }
                  frame True {
                  }
                }
                n140 = First Call?() -> (First Call?: T/F=w533:bool)
                n141 = Select(t=w529, s=w540, f=ENUM_Auto_State."Idle" ("State")) -> (s? t:f=w517:T10)
                n142 = Select(t=ENUM_Auto_Action."Drive" ("Action"), s=w540, f=ENUM_Auto_Action."No Action" ("Action")) -> (s? t:f=w539:T11)
                n143 = Bundle By Name(cluster=w536, "Target Angle(Degree)"=w525, "Steering"=0.0, "Encoder Target Position(in)"=0.0, "Zero Drive Encoders"=w533, "Zero YAW"=w533, "CMD_Drive_Data.Drive_Mode"=ENUM_WC_Drive_DriveMode."VBus", "Lock Angle"=TRUE, "Switch Booleans.Rotated"=w520) -> (w535:T12)
                n144 = Build Array(w539, ENUM_Auto_Action."Zero Drive Encoders" ("Action"), ENUM_Auto_Action."Zero YAW" ("Action"), ENUM_Auto_Action."Lock Angle" ("Action")) -> (w516:T11[])
              }
              frame "Shutdown" {
                w548 = T11[] [enum."Reset All"] items=["No Action", "Reset Time", "Reset All", "Lock Angle", "Drive", "Zero Drive Encoders", "Zero YAW"] ("Actions")
              }
            }
          }
          frame "Cross Line" {
            n145 = case shown="\"Rotate To Angle\"" w555 {
              tunnel: w554 -> [w561 w564 w592 w621 w636 w640 w644]
              tunnel: [w561 w563 w591 w620 w636 w640 w644] -> w558
              tunnel: [ENUM_Auto_State."Idle" ("State") w574 w601 w630 ENUM_Auto_State."Shutdown" ("State") ENUM_Auto_State."Shutdown" ("State") ENUM_Auto_State."Shutdown" ("State")] -> w557
              tunnel: [w560 w567 w595 w624 w634 w638 w642] -> w553
              tunnel: w556 -> [_ _ _ _ _ _ _]
              tunnel: [_ _ _ _ TRUE TRUE TRUE] -> w552
              frame "Startup" {
                w560 = T11[] [enum."Reset All", enum."Reset Time"] items=["No Action", "Reset Time", "Reset All", "Lock Angle", "Drive", "Zero Drive Encoders", "Zero YAW"] ("Actions")
              }
              frame "Idle" {
                n146 = Unbundle By Name(w564) -> ("Test"=w566:dbl)
                n147 = Less?(x=w566, y=2.0) -> (x < y?=w569:bool)
                n148 = Select(t=ENUM_Auto_State."Cross Line" ("State"), s=w569, f=ENUM_Auto_State."Shutdown" ("State")) -> (s? t:f=w574:T10)
                n149 = Select(t=ENUM_Auto_Action."Reset All" ("Action"), s=w569, f=ENUM_Auto_Action."No Action" ("Action")) -> (s? t:f=w568:T11)
                n150 = Build Array(w568) -> (w567:T11[])
                n151 = Bundle By Name(cluster=w564, "Encoder Target Position(in)"=94.0) -> (w563:T12)
              }
              frame "Cross Line" {
                w577 = 120.0 ("Encoder Target Position(in)")
                n152 = Unbundle By Name(w592) -> ("Zero YAW"=w583:bool, "Left Encoder"=w581:i32, "Right Encoder"=w580:i32, "Test"=w594:dbl)
                n153 = Greater?(x=w594, y=0.5) -> (0:w597:bool)
                n154 = call "EncoderPositionCalc.vi"("PositionTarget(in)"=4092.0, "Wheel Size(in)"=6.0, "EncoderCount/Revolution"=w577) -> ("PostionTarget(Counts)"=w578:i32)  [unwired: 8 in]
                n155 = call "AUTO_Encoder_In_Range_Check.vi"("Right Encoder"=w580, "Left Encoder"=w581, "PostionTarget(Counts)"=w578) -> ("Boolean"=w579:bool)  [unwired: 8 in]
                n156 = case shown="True" w579 {
                  tunnel: [ENUM_Auto_State."Cross Line" ("State") ENUM_Auto_State."Shutdown" ("State")] -> w582
                  frame False {
                  }
                  frame True {
                  }
                }
                n157 = First Call?() -> (First Call?: T/F=w584:bool)
                n158 = Select(t=w582, s=w597, f=ENUM_Auto_State."Idle" ("State")) -> (s? t:f=w601:T10)
                n159 = Select(t=ENUM_Auto_Action."Drive" ("Action"), s=w597, f=ENUM_Auto_Action."No Action" ("Action")) -> (s? t:f=w596:T11)
                n160 = Bundle By Name(cluster=w592, "Target Angle(Degree)"=0.0, "Steering"=0.0, "Encoder Target Position(in)"=w577, "Zero Drive Encoders"=w584, "Zero YAW"=w583, "CMD_Drive_Data.Drive_Mode"=ENUM_WC_Drive_DriveMode."Motion Profile") -> (w591:T12)
                n161 = Build Array(w596, ENUM_Auto_Action."Zero Drive Encoders" ("Action"), ENUM_Auto_Action."Zero YAW" ("Action"), ENUM_Auto_Action."Lock Angle" ("Action")) -> (w595:T11[])
              }
              frame "Rotate To Angle" {
                w609 = 3.0 ("y")
                w605 = 180.0 ("Target Angle(Degree)")
                n162 = Unbundle By Name(w621) -> ("YAW"=w604:dbl, "Test"=w623:dbl)
                n163 = Greater?(x=w623, y=0.5) -> (0:w626:bool)
                n164 = Add(x=w605, y=w609) -> (x+y=w611:dbl)
                n165 = Subtract(x=w605, y=w609) -> (x-y=w610:dbl)
                n166 = In Range and Coerce(upper limit=w611, x=w604, lower limit=w610) -> (In Range?=w606:bool)  [unwired: 1 out]
                n167 = Select(t=w604, s=w606, f=w605) -> (s? t:f=w607:dbl)
                n168 = case shown="False" w606 {
                  tunnel: [ENUM_Auto_State."Cross Line" ("State") ENUM_Auto_State."Cross Line" ("State")] -> w613
                  frame False {
                  }
                  frame True {
                  }
                }
                n169 = First Call?() -> (First Call?: T/F=w617:bool)
                n170 = Select(t=w613, s=w626, f=ENUM_Auto_State."Idle" ("State")) -> (s? t:f=w630:T10)
                n171 = Select(t=ENUM_Auto_Action."Drive" ("Action"), s=w626, f=ENUM_Auto_Action."No Action" ("Action")) -> (s? t:f=w625:T11)
                n172 = Bundle By Name(cluster=w621, "Target Angle(Degree)"=w607, "Steering"=0.0, "Encoder Target Position(in)"=0.0, "Zero Drive Encoders"=w617, "Zero YAW"=w617, "CMD_Drive_Data.Drive_Mode"=ENUM_WC_Drive_DriveMode."VBus", "Lock Angle"=TRUE) -> (w620:T12)
                n173 = Build Array(w625, ENUM_Auto_Action."Zero Drive Encoders" ("Action"), ENUM_Auto_Action."Zero YAW" ("Action"), ENUM_Auto_Action."Lock Angle" ("Action")) -> (w624:T11[])
              }
              frame "Shutdown" {
                w634 = T11[] [enum."Reset All"] items=["No Action", "Reset Time", "Reset All", "Lock Angle", "Drive", "Zero Drive Encoders", "Zero YAW"] ("Actions")
              }
              frame "position claw arm lift" {
                w638 = T11[] [enum."Reset All"] items=["No Action", "Reset Time", "Reset All", "Lock Angle", "Drive", "Zero Drive Encoders", "Zero YAW"] ("Actions")
              }
              frame "Intake" {
                w642 = T11[] [enum."Reset All"] items=["No Action", "Reset Time", "Reset All", "Lock Angle", "Drive", "Zero Drive Encoders", "Zero YAW"] ("Actions")
              }
            }
          }
          frame "No Movement" {
            n174 = case shown="\"Intake\"" w648 {
              tunnel: w647 -> [w654 w657 w670 w673 w676 w679 w683]
              tunnel: [w654 w656 w670 w673 w676 w679 w683] -> w651
              tunnel: [ENUM_Auto_State."Idle" ("State") w667 ENUM_Auto_State."Idle" ("State") ENUM_Auto_State."Idle" ("State") ENUM_Auto_State."Idle" ("State") ENUM_Auto_State."Idle" ("State") ENUM_Auto_State."Shutdown" ("State")] -> w650
              tunnel: [w653 w660 w668 w671 w674 w677 w681] -> w646
              tunnel: w649 -> [_ _ _ _ _ _ _]
              tunnel: [_ _ _ _ _ _ TRUE] -> w645
              frame "Startup" {
                w653 = T11[] [enum."Reset All", enum."Reset Time"] items=["No Action", "Reset Time", "Reset All", "Lock Angle", "Drive", "Zero Drive Encoders", "Zero YAW"] ("Actions")
              }
              frame "Idle" {
                n175 = Unbundle By Name(w657) -> ("Test"=w659:dbl)
                n176 = Less?(x=w659, y=2.0) -> (x < y?=w662:bool)
                n177 = Select(t=ENUM_Auto_State."Idle" ("State"), s=w662, f=ENUM_Auto_State."Shutdown" ("State")) -> (s? t:f=w667:T10)
                n178 = Select(t=ENUM_Auto_Action."Reset All" ("Action"), s=w662, f=ENUM_Auto_Action."No Action" ("Action")) -> (s? t:f=w661:T11)
                n179 = Build Array(w661) -> (w660:T11[])
                n180 = Bundle By Name(cluster=w657, "Encoder Target Position(in)"=120.0) -> (w656:T12)
              }
              frame "Cross Line" {
                w668 = T11[] [enum."No Action"] items=["No Action", "Reset Time", "Reset All", "Lock Angle", "Drive", "Zero Drive Encoders", "Zero YAW"] ("Actions")
              }
              frame "position claw arm lift" {
                w671 = T11[] [enum."No Action"] items=["No Action", "Reset Time", "Reset All", "Lock Angle", "Drive", "Zero Drive Encoders", "Zero YAW"] ("Actions")
              }
              frame "Intake" {
                w674 = T11[] [enum."No Action"] items=["No Action", "Reset Time", "Reset All", "Lock Angle", "Drive", "Zero Drive Encoders", "Zero YAW"] ("Actions")
              }
              frame "Rotate To Angle" {
                w677 = T11[] [enum."No Action"] items=["No Action", "Reset Time", "Reset All", "Lock Angle", "Drive", "Zero Drive Encoders", "Zero YAW"] ("Actions")
              }
              frame "Shutdown" {
                w681 = T11[] [enum."Reset All"] items=["No Action", "Reset Time", "Reset All", "Lock Angle", "Drive", "Zero Drive Encoders", "Zero YAW"] ("Actions")
              }
            }
          }
        }
        n181 = Bundle By Name(cluster=w64, "Previous State"=w61, "State"=w63) -> (w65:T12)
      }
      frame "RLR" {
        n182 = case shown="\"Switch\"" w684 {
          tunnel: [w699 w860 w1021 w1182 w1275] -> w691
          tunnel: [w693 w854 w1015 w1181 w1274] -> w690
          tunnel: w689 -> [w698 w859 w1020 w1180 w1273]
          tunnel: w688 -> [w697 w858 w1019 w1179 w1272]
          tunnel: w687 -> [w696 w857 w1018 w1178 w1271]
          tunnel: [w694 w855 w1016 w1177 w1270] -> w686
          tunnel: [w695 w856 w1017 w1176 w1269] -> w685
          frame "Switch" {
            n183 = case shown="\"Rotate To Angle\"" w697 {
              tunnel: w696 -> [w702 w708 w759 w774 w799 w838 w853]
              tunnel: [w702 w707 w758 w774 w798 w837 w853] -> w699
              tunnel: w698 -> [_ _ _ _ _ _ _]
              tunnel: [_ _ _ _ _ _ TRUE] -> w695
              tunnel: [ENUM_Auto_State."Idle" ("State") w703 w756 w772 w780 w819 ENUM_Auto_State."Shutdown" ("State")] -> w693
              tunnel: [w700 w704 w754 w773 w779 w818 w850] -> w694
              frame "Startup" {
                w700 = T11[] [enum."Reset All", enum."Reset Time"] items=["No Action", "Reset Time", "Reset All", "Lock Angle", "Drive", "Zero Drive Encoders", "Zero YAW"] ("Actions")
              }
              frame "Idle" {
                n184 = Unbundle By Name(w708) -> ("Switch Booleans.First Drive"=w713:bool, "Switch Booleans.Rotated"=w712:bool, "Switch Booleans.Second Move"=w711:bool, "Switch Booleans.Arm In position"=w710:bool, "Switch Booleans.Cube released"=w709:bool, "Test"=w715:dbl)
                n185 = Less?(x=w715, y=2.0) -> (x < y?=w717:bool)
                n186 = case shown="True" w713 {
                  tunnel: [ENUM_Auto_State."Cross Line" ("State") w730] -> w721
                  tunnel: w712 -> [_ w731]
                  tunnel: w711 -> [_ w729]
                  tunnel: w710 -> [_ w728]
                  tunnel: w709 -> [_ w727]
                  tunnel: [94.0 w725] -> w706
                  tunnel: [0.0 w726] -> w705
                  frame False {
                  }
                  frame True {
                    n187 = case shown="True" w731 {
                      tunnel: [ENUM_Auto_State."Rotate To Angle" ("State") w738] -> w730
                      tunnel: w729 -> [_ w737]
                      tunnel: w728 -> [_ w739]
                      tunnel: w727 -> [_ w735]
                      tunnel: [90.0 0.0] -> w726
                      tunnel: [0.0 w736] -> w725
                      frame False {
                      }
                      frame True {
                        n188 = case shown="False" w739 {
                          tunnel: [ENUM_Auto_State."position claw arm lift" ("State") w745] -> w738
                          tunnel: w737 -> [_ w746]
                          tunnel: [0.0 w744] -> w736
                          tunnel: w735 -> [_ w743]
                          frame False {
                          }
                          frame True {
                            n189 = case shown="True" w746 {
                              tunnel: [ENUM_Auto_State."Cross Line" ("State") w750] -> w745
                              tunnel: [32.0 0.0] -> w744
                              tunnel: w743 -> [_ w749]
                              frame False {
                              }
                              frame True {
                                n190 = case shown="True" w749 {
                                tunnel: [ENUM_Auto_State."Intake" ("State") ENUM_Auto_State."Shutdown" ("State")] -> w750
                                frame False {
                                }
                                frame True {
                                }
                                }
                              }
                            }
                          }
                        }
                      }
                    }
                  }
                }
                n191 = Select(t=w721, s=w717, f=ENUM_Auto_State."Shutdown" ("State")) -> (s? t:f=w703:T10)
                n192 = Select(t=ENUM_Auto_Action."Reset All" ("Action"), s=w717, f=ENUM_Auto_Action."No Action" ("Action")) -> (s? t:f=w716:T11)
                n193 = Bundle By Name(cluster=w708, "Encoder Target Position(in)"=w706, "Target Angle(Degree)"=w705) -> (w707:T12)
                n194 = Build Array(w716) -> (w704:T11[])
              }
              frame "position claw arm lift" {
                n195 = Unbundle By Name(w759) -> ("SM_Rotation_Output"=w762:T1)
                n196 = Equal?(x=w762, y=ENUM_Rotation_Positon."Switch" ("CMD_SM_Rotation.Rotation Positon")) -> (x = y?=w760:bool)
                n197 = case shown="True" w760 {
                  tunnel: [ENUM_Rotation_Positon."Switch" ("CMD_SM_Rotation.Rotation Positon") ENUM_Rotation_Positon."Switch" ("CMD_SM_Rotation.Rotation Positon")] -> w757
                  tunnel: [ENUM_Auto_State."position claw arm lift" ("State") ENUM_Auto_State."Idle" ("State")] -> w756
                  tunnel: [FALSE ("Switch Booleans.Arm In position") TRUE ("Switch Booleans.Arm In position")] -> w755
                  tunnel: [w763 w767] -> w754
                  frame False {
                    w763 = T11[] [enum."Drive"] items=["No Action", "Reset Time", "Reset All", "Lock Angle", "Drive", "Zero Drive Encoders", "Zero YAW"] ("Actions")
                  }
                  frame True {
                    w767 = T11[] [enum."No Action"] items=["No Action", "Reset Time", "Reset All", "Lock Angle", "Drive", "Zero Drive Encoders", "Zero YAW"] ("Actions")
                  }
                }
                n198 = Bundle By Name(cluster=w759, "CMD_SM_Rotation.Rotation Positon"=w757, "Switch Booleans.Arm In position"=w755) -> (w758:T12)
              }
              frame "Intake" {
                n199 = case shown="False" TRUE {
                  tunnel: [ENUM_Auto_State."Intake" ("State") ENUM_Auto_State."Idle" ("State")] -> w772
                  tunnel: [w775 w777] -> w773
                  frame False {
                    w775 = T11[] [enum."Drive"] items=["No Action", "Reset Time", "Reset All", "Lock Angle", "Drive", "Zero Drive Encoders", "Zero YAW"] ("Actions")
                  }
                  frame True {
                    w777 = T11[] [enum."No Action"] items=["No Action", "Reset Time", "Reset All", "Lock Angle", "Drive", "Zero Drive Encoders", "Zero YAW"] ("Actions")
                  }
                }
              }
              frame "Cross Line" {
                n200 = Unbundle By Name(w799) -> ("Encoder Target Position(in)"=w781:dbl, "Left Encoder"=w790:i32, "Right Encoder"=w789:i32, "Test"=w801:dbl, "Switch Booleans.First Drive"=w786:bool)
                n201 = call "EncoderPositionCalc.vi"("PositionTarget(in)"=w781, "Wheel Size(in)"=6.0, "EncoderCount/Revolution"=4096.0) -> ("PostionTarget(Counts)"=w788:i32)  [unwired: 8 in]
                n202 = call "AUTO_Encoder_In_Range_Check.vi"("Right Encoder"=w789, "Left Encoder"=w790, "PostionTarget(Counts)"=w788) -> ("Boolean"=w791:bool)  [unwired: 8 in]
                n203 = Greater?(x=w801, y=0.5) -> (0:w803:bool)
                n204 = case shown="False" w791 {
                  tunnel: [ENUM_Auto_State."Cross Line" ("State") w812] -> w792
                  tunnel: w786 -> [_ w811]
                  tunnel: [w807 w810] -> w785
                  tunnel: [w807 w809] -> w784
                  frame False {
                    w807 = FALSE
                  }
                  frame True {
                    n205 = case shown="False" w811 {
                      tunnel: [ENUM_Auto_State."Idle" ("State") ENUM_Auto_State."Idle" ("State")] -> w812
                      tunnel: [FALSE w816] -> w810
                      tunnel: [TRUE w816] -> w809
                      frame False {
                      }
                      frame True {
                        w816 = TRUE
                      }
                    }
                  }
                }
                n206 = First Call?() -> (First Call?: T/F=w794:bool)
                n207 = Select(t=w792, s=w803, f=ENUM_Auto_State."Idle" ("State")) -> (s? t:f=w780:T10)
                n208 = Select(t=ENUM_Auto_Action."Drive" ("Action"), s=w803, f=ENUM_Auto_Action."No Action" ("Action")) -> (s? t:f=w802:T11)
                n209 = Bundle By Name(cluster=w799, "Target Angle(Degree)"=0.0, "Steering"=0.0, "Encoder Target Position(in)"=w781, "Zero Drive Encoders"=w794, "Zero YAW"=w794, "CMD_Drive_Data.Drive_Mode"=ENUM_WC_Drive_DriveMode."Motion Profile", "Switch Booleans.First Drive"=w784, "Switch Booleans.Second Move"=w785) -> (w798:T12)
                n210 = Build Array(w802, ENUM_Auto_Action."Zero Drive Encoders" ("Action"), ENUM_Auto_Action."Lock Angle" ("Action")) -> (w779:T11[])
              }
              frame "Rotate To Angle" {
                w829 = 3.0 ("y")
                w825 = -90.0 ("Target Angle(Degree)")
                n211 = Unbundle By Name(w838) -> ("YAW"=w824:dbl, "Test"=w840:dbl)
                n212 = Greater?(x=w840, y=0.5) -> (0:w842:bool)
                n213 = Add(x=w825, y=w829) -> (x+y=w821:dbl)
                n214 = Subtract(x=w825, y=w829) -> (x-y=w820:dbl)
                n215 = In Range and Coerce(upper limit=w821, x=w824, lower limit=w820) -> (In Range?=w826:bool)  [unwired: 1 out]
                n216 = Select(t=w824, s=w826, f=w825) -> (s? t:f=w827:dbl)
                n217 = case shown="True" w826 {
                  tunnel: [ENUM_Auto_State."Rotate To Angle" ("State") ENUM_Auto_State."Idle" ("State")] -> w831
                  tunnel: [FALSE ("Lock Angle") TRUE ("Lock Angle")] -> w822
                  frame False {
                  }
                  frame True {
                  }
                }
                n218 = First Call?() -> (First Call?: T/F=w835:bool)
                n219 = Select(t=w831, s=w842, f=ENUM_Auto_State."Idle" ("State")) -> (s? t:f=w819:T10)
                n220 = Select(t=ENUM_Auto_Action."Drive" ("Action"), s=w842, f=ENUM_Auto_Action."No Action" ("Action")) -> (s? t:f=w841:T11)
                n221 = Bundle By Name(cluster=w838, "Target Angle(Degree)"=w827, "Steering"=0.0, "Encoder Target Position(in)"=0.0, "Zero Drive Encoders"=w835, "Zero YAW"=w835, "CMD_Drive_Data.Drive_Mode"=ENUM_WC_Drive_DriveMode."VBus", "Lock Angle"=TRUE, "Switch Booleans.Rotated"=w822) -> (w837:T12)
                n222 = Build Array(w841, ENUM_Auto_Action."Zero Drive Encoders" ("Action"), ENUM_Auto_Action."Zero YAW" ("Action"), ENUM_Auto_Action."Lock Angle" ("Action")) -> (w818:T11[])
              }
              frame "Shutdown" {
                w850 = T11[] [enum."Reset All"] items=["No Action", "Reset Time", "Reset All", "Lock Angle", "Drive", "Zero Drive Encoders", "Zero YAW"] ("Actions")
              }
            }
          }
          frame "Scale" {
            n223 = case shown="\"Rotate To Angle\"" w858 {
              tunnel: w857 -> [w863 w869 w920 w935 w960 w999 w1014]
              tunnel: [w863 w868 w919 w935 w959 w998 w1014] -> w860
              tunnel: w859 -> [_ _ _ _ _ _ _]
              tunnel: [_ _ _ _ _ _ TRUE] -> w856
              tunnel: [ENUM_Auto_State."Idle" ("State") w864 w917 w933 w941 w980 ENUM_Auto_State."Shutdown" ("State")] -> w854
              tunnel: [w861 w865 w915 w934 w940 w979 w1011] -> w855
              frame "Startup" {
                w861 = T11[] [enum."Reset All", enum."Reset Time"] items=["No Action", "Reset Time", "Reset All", "Lock Angle", "Drive", "Zero Drive Encoders", "Zero YAW"] ("Actions")
              }
              frame "Idle" {
                n224 = Unbundle By Name(w869) -> ("Switch Booleans.First Drive"=w874:bool, "Switch Booleans.Rotated"=w873:bool, "Switch Booleans.Second Move"=w872:bool, "Switch Booleans.Arm In position"=w871:bool, "Switch Booleans.Cube released"=w870:bool, "Test"=w876:dbl)
                n225 = Less?(x=w876, y=2.0) -> (x < y?=w878:bool)
                n226 = case shown="True" w874 {
                  tunnel: [ENUM_Auto_State."Cross Line" ("State") w891] -> w882
                  tunnel: w873 -> [_ w892]
                  tunnel: w872 -> [_ w890]
                  tunnel: w871 -> [_ w889]
                  tunnel: w870 -> [_ w888]
                  tunnel: [94.0 w886] -> w867
                  tunnel: [0.0 w887] -> w866
                  frame False {
                  }
                  frame True {
                    n227 = case shown="True" w892 {
                      tunnel: [ENUM_Auto_State."Rotate To Angle" ("State") w899] -> w891
                      tunnel: w890 -> [_ w898]
                      tunnel: w889 -> [_ w900]
                      tunnel: w888 -> [_ w896]
                      tunnel: [90.0 0.0] -> w887
                      tunnel: [0.0 w897] -> w886
                      frame False {
                      }
                      frame True {
                        n228 = case shown="False" w900 {
                          tunnel: [ENUM_Auto_State."position claw arm lift" ("State") w906] -> w899
                          tunnel: w898 -> [_ w907]
                          tunnel: [0.0 w905] -> w897
                          tunnel: w896 -> [_ w904]
                          frame False {
                          }
                          frame True {
                            n229 = case shown="True" w907 {
                              tunnel: [ENUM_Auto_State."Cross Line" ("State") w911] -> w906
                              tunnel: [32.0 0.0] -> w905
                              tunnel: w904 -> [_ w910]
                              frame False {
                              }
                              frame True {
                                n230 = case shown="True" w910 {
                                tunnel: [ENUM_Auto_State."Intake" ("State") ENUM_Auto_State."Shutdown" ("State")] -> w911
                                frame False {
                                }
                                frame True {
                                }
                                }
                              }
                            }
                          }
                        }
                      }
                    }
                  }
                }
                n231 = Select(t=w882, s=w878, f=ENUM_Auto_State."Shutdown" ("State")) -> (s? t:f=w864:T10)
                n232 = Select(t=ENUM_Auto_Action."Reset All" ("Action"), s=w878, f=ENUM_Auto_Action."No Action" ("Action")) -> (s? t:f=w877:T11)
                n233 = Bundle By Name(cluster=w869, "Encoder Target Position(in)"=w867, "Target Angle(Degree)"=w866) -> (w868:T12)
                n234 = Build Array(w877) -> (w865:T11[])
              }
              frame "position claw arm lift" {
                n235 = Unbundle By Name(w920) -> ("SM_Rotation_Output"=w923:T1)
                n236 = Equal?(x=w923, y=ENUM_Rotation_Positon."Switch" ("CMD_SM_Rotation.Rotation Positon")) -> (x = y?=w921:bool)
                n237 = case shown="True" w921 {
                  tunnel: [ENUM_Rotation_Positon."Switch" ("CMD_SM_Rotation.Rotation Positon") ENUM_Rotation_Positon."Switch" ("CMD_SM_Rotation.Rotation Positon")] -> w918
                  tunnel: [ENUM_Auto_State."position claw arm lift" ("State") ENUM_Auto_State."Idle" ("State")] -> w917
                  tunnel: [FALSE ("Switch Booleans.Arm In position") TRUE ("Switch Booleans.Arm In position")] -> w916
                  tunnel: [w924 w928] -> w915
                  frame False {
                    w924 = T11[] [enum."Drive"] items=["No Action", "Reset Time", "Reset All", "Lock Angle", "Drive", "Zero Drive Encoders", "Zero YAW"] ("Actions")
                  }
                  frame True {
                    w928 = T11[] [enum."No Action"] items=["No Action", "Reset Time", "Reset All", "Lock Angle", "Drive", "Zero Drive Encoders", "Zero YAW"] ("Actions")
                  }
                }
                n238 = Bundle By Name(cluster=w920, "CMD_SM_Rotation.Rotation Positon"=w918, "Switch Booleans.Arm In position"=w916) -> (w919:T12)
              }
              frame "Intake" {
                n239 = case shown="False" TRUE {
                  tunnel: [ENUM_Auto_State."Intake" ("State") ENUM_Auto_State."Idle" ("State")] -> w933
                  tunnel: [w936 w938] -> w934
                  frame False {
                    w936 = T11[] [enum."Drive"] items=["No Action", "Reset Time", "Reset All", "Lock Angle", "Drive", "Zero Drive Encoders", "Zero YAW"] ("Actions")
                  }
                  frame True {
                    w938 = T11[] [enum."No Action"] items=["No Action", "Reset Time", "Reset All", "Lock Angle", "Drive", "Zero Drive Encoders", "Zero YAW"] ("Actions")
                  }
                }
              }
              frame "Cross Line" {
                n240 = Unbundle By Name(w960) -> ("Encoder Target Position(in)"=w942:dbl, "Left Encoder"=w951:i32, "Right Encoder"=w950:i32, "Test"=w962:dbl, "Switch Booleans.First Drive"=w947:bool)
                n241 = call "EncoderPositionCalc.vi"("PositionTarget(in)"=w942, "Wheel Size(in)"=6.0, "EncoderCount/Revolution"=4096.0) -> ("PostionTarget(Counts)"=w949:i32)  [unwired: 8 in]
                n242 = call "AUTO_Encoder_In_Range_Check.vi"("Right Encoder"=w950, "Left Encoder"=w951, "PostionTarget(Counts)"=w949) -> ("Boolean"=w952:bool)  [unwired: 8 in]
                n243 = Greater?(x=w962, y=0.5) -> (0:w964:bool)
                n244 = case shown="False" w952 {
                  tunnel: [ENUM_Auto_State."Cross Line" ("State") w973] -> w953
                  tunnel: w947 -> [_ w972]
                  tunnel: [w968 w971] -> w946
                  tunnel: [w968 w970] -> w945
                  frame False {
                    w968 = FALSE
                  }
                  frame True {
                    n245 = case shown="False" w972 {
                      tunnel: [ENUM_Auto_State."Idle" ("State") ENUM_Auto_State."Idle" ("State")] -> w973
                      tunnel: [FALSE w977] -> w971
                      tunnel: [TRUE w977] -> w970
                      frame False {
                      }
                      frame True {
                        w977 = TRUE
                      }
                    }
                  }
                }
                n246 = First Call?() -> (First Call?: T/F=w955:bool)
                n247 = Select(t=w953, s=w964, f=ENUM_Auto_State."Idle" ("State")) -> (s? t:f=w941:T10)
                n248 = Select(t=ENUM_Auto_Action."Drive" ("Action"), s=w964, f=ENUM_Auto_Action."No Action" ("Action")) -> (s? t:f=w963:T11)
                n249 = Bundle By Name(cluster=w960, "Target Angle(Degree)"=0.0, "Steering"=0.0, "Encoder Target Position(in)"=w942, "Zero Drive Encoders"=w955, "Zero YAW"=w955, "CMD_Drive_Data.Drive_Mode"=ENUM_WC_Drive_DriveMode."Motion Profile", "Switch Booleans.First Drive"=w945, "Switch Booleans.Second Move"=w946) -> (w959:T12)
                n250 = Build Array(w963, ENUM_Auto_Action."Zero Drive Encoders" ("Action"), ENUM_Auto_Action."Lock Angle" ("Action")) -> (w940:T11[])
              }
              frame "Rotate To Angle" {
                w990 = 3.0 ("y")
                w986 = -90.0 ("Target Angle(Degree)")
                n251 = Unbundle By Name(w999) -> ("YAW"=w985:dbl, "Test"=w1001:dbl)
                n252 = Greater?(x=w1001, y=0.5) -> (0:w1003:bool)
                n253 = Add(x=w986, y=w990) -> (x+y=w982:dbl)
                n254 = Subtract(x=w986, y=w990) -> (x-y=w981:dbl)
                n255 = In Range and Coerce(upper limit=w982, x=w985, lower limit=w981) -> (In Range?=w987:bool)  [unwired: 1 out]
                n256 = Select(t=w985, s=w987, f=w986) -> (s? t:f=w988:dbl)
                n257 = case shown="True" w987 {
                  tunnel: [ENUM_Auto_State."Rotate To Angle" ("State") ENUM_Auto_State."Idle" ("State")] -> w992
                  tunnel: [FALSE ("Lock Angle") TRUE ("Lock Angle")] -> w983
                  frame False {
                  }
                  frame True {
                  }
                }
                n258 = First Call?() -> (First Call?: T/F=w996:bool)
                n259 = Select(t=w992, s=w1003, f=ENUM_Auto_State."Idle" ("State")) -> (s? t:f=w980:T10)
                n260 = Select(t=ENUM_Auto_Action."Drive" ("Action"), s=w1003, f=ENUM_Auto_Action."No Action" ("Action")) -> (s? t:f=w1002:T11)
                n261 = Bundle By Name(cluster=w999, "Target Angle(Degree)"=w988, "Steering"=0.0, "Encoder Target Position(in)"=0.0, "Zero Drive Encoders"=w996, "Zero YAW"=w996, "CMD_Drive_Data.Drive_Mode"=ENUM_WC_Drive_DriveMode."VBus", "Lock Angle"=TRUE, "Switch Booleans.Rotated"=w983) -> (w998:T12)
                n262 = Build Array(w1002, ENUM_Auto_Action."Zero Drive Encoders" ("Action"), ENUM_Auto_Action."Zero YAW" ("Action"), ENUM_Auto_Action."Lock Angle" ("Action")) -> (w979:T11[])
              }
              frame "Shutdown" {
                w1011 = T11[] [enum."Reset All"] items=["No Action", "Reset Time", "Reset All", "Lock Angle", "Drive", "Zero Drive Encoders", "Zero YAW"] ("Actions")
              }
            }
          }
          frame "Scale And Switch" {
            n263 = case shown="\"Rotate To Angle\"" w1019 {
              tunnel: w1018 -> [w1024 w1030 w1081 w1096 w1121 w1160 w1175]
              tunnel: [w1024 w1029 w1080 w1096 w1120 w1159 w1175] -> w1021
              tunnel: w1020 -> [_ _ _ _ _ _ _]
              tunnel: [_ _ _ _ _ _ TRUE] -> w1017
              tunnel: [ENUM_Auto_State."Idle" ("State") w1025 w1078 w1094 w1102 w1141 ENUM_Auto_State."Shutdown" ("State")] -> w1015
              tunnel: [w1022 w1026 w1076 w1095 w1101 w1140 w1172] -> w1016
              frame "Startup" {
                w1022 = T11[] [enum."Reset All", enum."Reset Time"] items=["No Action", "Reset Time", "Reset All", "Lock Angle", "Drive", "Zero Drive Encoders", "Zero YAW"] ("Actions")
              }
              frame "Idle" {
                n264 = Unbundle By Name(w1030) -> ("Switch Booleans.First Drive"=w1035:bool, "Switch Booleans.Rotated"=w1034:bool, "Switch Booleans.Second Move"=w1033:bool, "Switch Booleans.Arm In position"=w1032:bool, "Switch Booleans.Cube released"=w1031:bool, "Test"=w1037:dbl)
                n265 = Less?(x=w1037, y=2.0) -> (x < y?=w1039:bool)
                n266 = case shown="True" w1035 {
                  tunnel: [ENUM_Auto_State."Cross Line" ("State") w1052] -> w1043
                  tunnel: w1034 -> [_ w1053]
                  tunnel: w1033 -> [_ w1051]
                  tunnel: w1032 -> [_ w1050]
                  tunnel: w1031 -> [_ w1049]
                  tunnel: [94.0 w1047] -> w1028
                  tunnel: [0.0 w1048] -> w1027
                  frame False {
                  }
                  frame True {
                    n267 = case shown="True" w1053 {
                      tunnel: [ENUM_Auto_State."Rotate To Angle" ("State") w1060] -> w1052
                      tunnel: w1051 -> [_ w1059]
                      tunnel: w1050 -> [_ w1061]
                      tunnel: w1049 -> [_ w1057]
                      tunnel: [90.0 0.0] -> w1048
                      tunnel: [0.0 w1058] -> w1047
                      frame False {
                      }
                      frame True {
                        n268 = case shown="False" w1061 {
                          tunnel: [ENUM_Auto_State."position claw arm lift" ("State") w1067] -> w1060
                          tunnel: w1059 -> [_ w1068]
                          tunnel: [0.0 w1066] -> w1058
                          tunnel: w1057 -> [_ w1065]
                          frame False {
                          }
                          frame True {
                            n269 = case shown="True" w1068 {
                              tunnel: [ENUM_Auto_State."Cross Line" ("State") w1072] -> w1067
                              tunnel: [32.0 0.0] -> w1066
                              tunnel: w1065 -> [_ w1071]
                              frame False {
                              }
                              frame True {
                                n270 = case shown="True" w1071 {
                                tunnel: [ENUM_Auto_State."Intake" ("State") ENUM_Auto_State."Shutdown" ("State")] -> w1072
                                frame False {
                                }
                                frame True {
                                }
                                }
                              }
                            }
                          }
                        }
                      }
                    }
                  }
                }
                n271 = Select(t=w1043, s=w1039, f=ENUM_Auto_State."Shutdown" ("State")) -> (s? t:f=w1025:T10)
                n272 = Select(t=ENUM_Auto_Action."Reset All" ("Action"), s=w1039, f=ENUM_Auto_Action."No Action" ("Action")) -> (s? t:f=w1038:T11)
                n273 = Bundle By Name(cluster=w1030, "Encoder Target Position(in)"=w1028, "Target Angle(Degree)"=w1027) -> (w1029:T12)
                n274 = Build Array(w1038) -> (w1026:T11[])
              }
              frame "position claw arm lift" {
                n275 = Unbundle By Name(w1081) -> ("SM_Rotation_Output"=w1084:T1)
                n276 = Equal?(x=w1084, y=ENUM_Rotation_Positon."Switch" ("CMD_SM_Rotation.Rotation Positon")) -> (x = y?=w1082:bool)
                n277 = case shown="True" w1082 {
                  tunnel: [ENUM_Rotation_Positon."Switch" ("CMD_SM_Rotation.Rotation Positon") ENUM_Rotation_Positon."Switch" ("CMD_SM_Rotation.Rotation Positon")] -> w1079
                  tunnel: [ENUM_Auto_State."position claw arm lift" ("State") ENUM_Auto_State."Idle" ("State")] -> w1078
                  tunnel: [FALSE ("Switch Booleans.Arm In position") TRUE ("Switch Booleans.Arm In position")] -> w1077
                  tunnel: [w1085 w1089] -> w1076
                  frame False {
                    w1085 = T11[] [enum."Drive"] items=["No Action", "Reset Time", "Reset All", "Lock Angle", "Drive", "Zero Drive Encoders", "Zero YAW"] ("Actions")
                  }
                  frame True {
                    w1089 = T11[] [enum."No Action"] items=["No Action", "Reset Time", "Reset All", "Lock Angle", "Drive", "Zero Drive Encoders", "Zero YAW"] ("Actions")
                  }
                }
                n278 = Bundle By Name(cluster=w1081, "CMD_SM_Rotation.Rotation Positon"=w1079, "Switch Booleans.Arm In position"=w1077) -> (w1080:T12)
              }
              frame "Intake" {
                n279 = case shown="False" TRUE {
                  tunnel: [ENUM_Auto_State."Intake" ("State") ENUM_Auto_State."Idle" ("State")] -> w1094
                  tunnel: [w1097 w1099] -> w1095
                  frame False {
                    w1097 = T11[] [enum."Drive"] items=["No Action", "Reset Time", "Reset All", "Lock Angle", "Drive", "Zero Drive Encoders", "Zero YAW"] ("Actions")
                  }
                  frame True {
                    w1099 = T11[] [enum."No Action"] items=["No Action", "Reset Time", "Reset All", "Lock Angle", "Drive", "Zero Drive Encoders", "Zero YAW"] ("Actions")
                  }
                }
              }
              frame "Cross Line" {
                n280 = Unbundle By Name(w1121) -> ("Encoder Target Position(in)"=w1103:dbl, "Left Encoder"=w1112:i32, "Right Encoder"=w1111:i32, "Test"=w1123:dbl, "Switch Booleans.First Drive"=w1108:bool)
                n281 = call "EncoderPositionCalc.vi"("PositionTarget(in)"=w1103, "Wheel Size(in)"=6.0, "EncoderCount/Revolution"=4096.0) -> ("PostionTarget(Counts)"=w1110:i32)  [unwired: 8 in]
                n282 = call "AUTO_Encoder_In_Range_Check.vi"("Right Encoder"=w1111, "Left Encoder"=w1112, "PostionTarget(Counts)"=w1110) -> ("Boolean"=w1113:bool)  [unwired: 8 in]
                n283 = Greater?(x=w1123, y=0.5) -> (0:w1125:bool)
                n284 = case shown="False" w1113 {
                  tunnel: [ENUM_Auto_State."Cross Line" ("State") w1134] -> w1114
                  tunnel: w1108 -> [_ w1133]
                  tunnel: [w1129 w1132] -> w1107
                  tunnel: [w1129 w1131] -> w1106
                  frame False {
                    w1129 = FALSE
                  }
                  frame True {
                    n285 = case shown="False" w1133 {
                      tunnel: [ENUM_Auto_State."Idle" ("State") ENUM_Auto_State."Idle" ("State")] -> w1134
                      tunnel: [FALSE w1138] -> w1132
                      tunnel: [TRUE w1138] -> w1131
                      frame False {
                      }
                      frame True {
                        w1138 = TRUE
                      }
                    }
                  }
                }
                n286 = First Call?() -> (First Call?: T/F=w1116:bool)
                n287 = Select(t=w1114, s=w1125, f=ENUM_Auto_State."Idle" ("State")) -> (s? t:f=w1102:T10)
                n288 = Select(t=ENUM_Auto_Action."Drive" ("Action"), s=w1125, f=ENUM_Auto_Action."No Action" ("Action")) -> (s? t:f=w1124:T11)
                n289 = Bundle By Name(cluster=w1121, "Target Angle(Degree)"=0.0, "Steering"=0.0, "Encoder Target Position(in)"=w1103, "Zero Drive Encoders"=w1116, "Zero YAW"=w1116, "CMD_Drive_Data.Drive_Mode"=ENUM_WC_Drive_DriveMode."Motion Profile", "Switch Booleans.First Drive"=w1106, "Switch Booleans.Second Move"=w1107) -> (w1120:T12)
                n290 = Build Array(w1124, ENUM_Auto_Action."Zero Drive Encoders" ("Action"), ENUM_Auto_Action."Lock Angle" ("Action")) -> (w1101:T11[])
              }
              frame "Rotate To Angle" {
                w1151 = 3.0 ("y")
                w1147 = -90.0 ("Target Angle(Degree)")
                n291 = Unbundle By Name(w1160) -> ("YAW"=w1146:dbl, "Test"=w1162:dbl)
                n292 = Greater?(x=w1162, y=0.5) -> (0:w1164:bool)
                n293 = Add(x=w1147, y=w1151) -> (x+y=w1143:dbl)
                n294 = Subtract(x=w1147, y=w1151) -> (x-y=w1142:dbl)
                n295 = In Range and Coerce(upper limit=w1143, x=w1146, lower limit=w1142) -> (In Range?=w1148:bool)  [unwired: 1 out]
                n296 = Select(t=w1146, s=w1148, f=w1147) -> (s? t:f=w1149:dbl)
                n297 = case shown="True" w1148 {
                  tunnel: [ENUM_Auto_State."Rotate To Angle" ("State") ENUM_Auto_State."Idle" ("State")] -> w1153
                  tunnel: [FALSE ("Lock Angle") TRUE ("Lock Angle")] -> w1144
                  frame False {
                  }
                  frame True {
                  }
                }
                n298 = First Call?() -> (First Call?: T/F=w1157:bool)
                n299 = Select(t=w1153, s=w1164, f=ENUM_Auto_State."Idle" ("State")) -> (s? t:f=w1141:T10)
                n300 = Select(t=ENUM_Auto_Action."Drive" ("Action"), s=w1164, f=ENUM_Auto_Action."No Action" ("Action")) -> (s? t:f=w1163:T11)
                n301 = Bundle By Name(cluster=w1160, "Target Angle(Degree)"=w1149, "Steering"=0.0, "Encoder Target Position(in)"=0.0, "Zero Drive Encoders"=w1157, "Zero YAW"=w1157, "CMD_Drive_Data.Drive_Mode"=ENUM_WC_Drive_DriveMode."VBus", "Lock Angle"=TRUE, "Switch Booleans.Rotated"=w1144) -> (w1159:T12)
                n302 = Build Array(w1163, ENUM_Auto_Action."Zero Drive Encoders" ("Action"), ENUM_Auto_Action."Zero YAW" ("Action"), ENUM_Auto_Action."Lock Angle" ("Action")) -> (w1140:T11[])
              }
              frame "Shutdown" {
                w1172 = T11[] [enum."Reset All"] items=["No Action", "Reset Time", "Reset All", "Lock Angle", "Drive", "Zero Drive Encoders", "Zero YAW"] ("Actions")
              }
            }
          }
          frame "Cross Line" {
            n303 = case shown="\"Rotate To Angle\"" w1179 {
              tunnel: w1178 -> [w1185 w1188 w1216 w1245 w1260 w1264 w1268]
              tunnel: [w1185 w1187 w1215 w1244 w1260 w1264 w1268] -> w1182
              tunnel: [ENUM_Auto_State."Idle" ("State") w1198 w1225 w1254 ENUM_Auto_State."Shutdown" ("State") ENUM_Auto_State."Shutdown" ("State") ENUM_Auto_State."Shutdown" ("State")] -> w1181
              tunnel: [w1184 w1191 w1219 w1248 w1258 w1262 w1266] -> w1177
              tunnel: w1180 -> [_ _ _ _ _ _ _]
              tunnel: [_ _ _ _ TRUE TRUE TRUE] -> w1176
              frame "Startup" {
                w1184 = T11[] [enum."Reset All", enum."Reset Time"] items=["No Action", "Reset Time", "Reset All", "Lock Angle", "Drive", "Zero Drive Encoders", "Zero YAW"] ("Actions")
              }
              frame "Idle" {
                n304 = Unbundle By Name(w1188) -> ("Test"=w1190:dbl)
                n305 = Less?(x=w1190, y=2.0) -> (x < y?=w1193:bool)
                n306 = Select(t=ENUM_Auto_State."Cross Line" ("State"), s=w1193, f=ENUM_Auto_State."Shutdown" ("State")) -> (s? t:f=w1198:T10)
                n307 = Select(t=ENUM_Auto_Action."Reset All" ("Action"), s=w1193, f=ENUM_Auto_Action."No Action" ("Action")) -> (s? t:f=w1192:T11)
                n308 = Build Array(w1192) -> (w1191:T11[])
                n309 = Bundle By Name(cluster=w1188, "Encoder Target Position(in)"=120.0) -> (w1187:T12)
              }
              frame "Cross Line" {
                w1201 = 120.0 ("Encoder Target Position(in)")
                n310 = Unbundle By Name(w1216) -> ("Zero YAW"=w1207:bool, "Left Encoder"=w1205:i32, "Right Encoder"=w1204:i32, "Test"=w1218:dbl)
                n311 = Greater?(x=w1218, y=0.5) -> (0:w1221:bool)
                n312 = call "EncoderPositionCalc.vi"("PositionTarget(in)"=4092.0, "Wheel Size(in)"=6.0, "EncoderCount/Revolution"=w1201) -> ("PostionTarget(Counts)"=w1202:i32)  [unwired: 8 in]
                n313 = call "AUTO_Encoder_In_Range_Check.vi"("Right Encoder"=w1204, "Left Encoder"=w1205, "PostionTarget(Counts)"=w1202) -> ("Boolean"=w1203:bool)  [unwired: 8 in]
                n314 = case shown="True" w1203 {
                  tunnel: [ENUM_Auto_State."Cross Line" ("State") ENUM_Auto_State."Shutdown" ("State")] -> w1206
                  frame False {
                  }
                  frame True {
                  }
                }
                n315 = First Call?() -> (First Call?: T/F=w1208:bool)
                n316 = Select(t=w1206, s=w1221, f=ENUM_Auto_State."Idle" ("State")) -> (s? t:f=w1225:T10)
                n317 = Select(t=ENUM_Auto_Action."Drive" ("Action"), s=w1221, f=ENUM_Auto_Action."No Action" ("Action")) -> (s? t:f=w1220:T11)
                n318 = Bundle By Name(cluster=w1216, "Target Angle(Degree)"=0.0, "Steering"=0.0, "Encoder Target Position(in)"=w1201, "Zero Drive Encoders"=w1208, "Zero YAW"=w1207, "CMD_Drive_Data.Drive_Mode"=ENUM_WC_Drive_DriveMode."Motion Profile") -> (w1215:T12)
                n319 = Build Array(w1220, ENUM_Auto_Action."Zero Drive Encoders" ("Action"), ENUM_Auto_Action."Zero YAW" ("Action"), ENUM_Auto_Action."Lock Angle" ("Action")) -> (w1219:T11[])
              }
              frame "Rotate To Angle" {
                w1233 = 3.0 ("y")
                w1229 = 180.0 ("Target Angle(Degree)")
                n320 = Unbundle By Name(w1245) -> ("YAW"=w1228:dbl, "Test"=w1247:dbl)
                n321 = Greater?(x=w1247, y=0.5) -> (0:w1250:bool)
                n322 = Add(x=w1229, y=w1233) -> (x+y=w1235:dbl)
                n323 = Subtract(x=w1229, y=w1233) -> (x-y=w1234:dbl)
                n324 = In Range and Coerce(upper limit=w1235, x=w1228, lower limit=w1234) -> (In Range?=w1230:bool)  [unwired: 1 out]
                n325 = Select(t=w1228, s=w1230, f=w1229) -> (s? t:f=w1231:dbl)
                n326 = case shown="False" w1230 {
                  tunnel: [ENUM_Auto_State."Cross Line" ("State") ENUM_Auto_State."Cross Line" ("State")] -> w1237
                  frame False {
                  }
                  frame True {
                  }
                }
                n327 = First Call?() -> (First Call?: T/F=w1241:bool)
                n328 = Select(t=w1237, s=w1250, f=ENUM_Auto_State."Idle" ("State")) -> (s? t:f=w1254:T10)
                n329 = Select(t=ENUM_Auto_Action."Drive" ("Action"), s=w1250, f=ENUM_Auto_Action."No Action" ("Action")) -> (s? t:f=w1249:T11)
                n330 = Bundle By Name(cluster=w1245, "Target Angle(Degree)"=w1231, "Steering"=0.0, "Encoder Target Position(in)"=0.0, "Zero Drive Encoders"=w1241, "Zero YAW"=w1241, "CMD_Drive_Data.Drive_Mode"=ENUM_WC_Drive_DriveMode."VBus", "Lock Angle"=TRUE) -> (w1244:T12)
                n331 = Build Array(w1249, ENUM_Auto_Action."Zero Drive Encoders" ("Action"), ENUM_Auto_Action."Zero YAW" ("Action"), ENUM_Auto_Action."Lock Angle" ("Action")) -> (w1248:T11[])
              }
              frame "Shutdown" {
                w1258 = T11[] [enum."Reset All"] items=["No Action", "Reset Time", "Reset All", "Lock Angle", "Drive", "Zero Drive Encoders", "Zero YAW"] ("Actions")
              }
              frame "position claw arm lift" {
                w1262 = T11[] [enum."Reset All"] items=["No Action", "Reset Time", "Reset All", "Lock Angle", "Drive", "Zero Drive Encoders", "Zero YAW"] ("Actions")
              }
              frame "Intake" {
                w1266 = T11[] [enum."Reset All"] items=["No Action", "Reset Time", "Reset All", "Lock Angle", "Drive", "Zero Drive Encoders", "Zero YAW"] ("Actions")
              }
            }
          }
          frame "No Movement" {
            n332 = case shown="\"Intake\"" w1272 {
              tunnel: w1271 -> [w1278 w1281 w1294 w1297 w1301 w1305 w1309]
              tunnel: [w1278 w1280 w1294 w1297 w1301 w1305 w1309] -> w1275
              tunnel: [ENUM_Auto_State."Idle" ("State") w1291 ENUM_Auto_State."Idle" ("State") ENUM_Auto_State."Idle" ("State") ENUM_Auto_State."Shutdown" ("State") ENUM_Auto_State."Shutdown" ("State") ENUM_Auto_State."Shutdown" ("State")] -> w1274
              tunnel: [w1277 w1284 w1292 w1295 w1299 w1303 w1307] -> w1270
              tunnel: w1273 -> [_ _ _ _ _ _ _]
              tunnel: [_ _ _ _ TRUE TRUE TRUE] -> w1269
              frame "Startup" {
                w1277 = T11[] [enum."Reset All", enum."Reset Time"] items=["No Action", "Reset Time", "Reset All", "Lock Angle", "Drive", "Zero Drive Encoders", "Zero YAW"] ("Actions")
              }
              frame "Idle" {
                n333 = Unbundle By Name(w1281) -> ("Test"=w1283:dbl)
                n334 = Less?(x=w1283, y=2.0) -> (x < y?=w1286:bool)
                n335 = Select(t=ENUM_Auto_State."Idle" ("State"), s=w1286, f=ENUM_Auto_State."Shutdown" ("State")) -> (s? t:f=w1291:T10)
                n336 = Select(t=ENUM_Auto_Action."Reset All" ("Action"), s=w1286, f=ENUM_Auto_Action."No Action" ("Action")) -> (s? t:f=w1285:T11)
                n337 = Build Array(w1285) -> (w1284:T11[])
                n338 = Bundle By Name(cluster=w1281, "Encoder Target Position(in)"=120.0) -> (w1280:T12)
              }
              frame "Cross Line" {
                w1292 = T11[] [enum."No Action"] items=["No Action", "Reset Time", "Reset All", "Lock Angle", "Drive", "Zero Drive Encoders", "Zero YAW"] ("Actions")
              }
              frame "Rotate To Angle" {
                w1295 = T11[] [enum."No Action"] items=["No Action", "Reset Time", "Reset All", "Lock Angle", "Drive", "Zero Drive Encoders", "Zero YAW"] ("Actions")
              }
              frame "Shutdown" {
                w1299 = T11[] [enum."Reset All"] items=["No Action", "Reset Time", "Reset All", "Lock Angle", "Drive", "Zero Drive Encoders", "Zero YAW"] ("Actions")
              }
              frame "position claw arm lift" {
                w1303 = T11[] [enum."Reset All"] items=["No Action", "Reset Time", "Reset All", "Lock Angle", "Drive", "Zero Drive Encoders", "Zero YAW"] ("Actions")
              }
              frame "Intake" {
                w1307 = T11[] [enum."Reset All"] items=["No Action", "Reset Time", "Reset All", "Lock Angle", "Drive", "Zero Drive Encoders", "Zero YAW"] ("Actions")
              }
            }
          }
        }
        n339 = Bundle By Name(cluster=w691, "Previous State"=w688, "State"=w690) -> (w692:T12)
      }
      frame "RRR" {
        n340 = case shown="\"Cross Line\"" w1310 {
          tunnel: [w1325 w1486 w1647 w1808 w1901] -> w1317
          tunnel: [w1319 w1480 w1641 w1807 w1900] -> w1316
          tunnel: w1315 -> [w1324 w1485 w1646 w1806 w1899]
          tunnel: w1314 -> [w1323 w1484 w1645 w1805 w1898]
          tunnel: w1313 -> [w1322 w1483 w1644 w1804 w1897]
          tunnel: [w1320 w1481 w1642 w1803 w1896] -> w1312
          tunnel: [w1321 w1482 w1643 w1802 w1895] -> w1311
          frame "Switch" {
            n341 = case shown="\"Rotate To Angle\"" w1323 {
              tunnel: w1322 -> [w1328 w1334 w1385 w1400 w1425 w1464 w1479]
              tunnel: [w1328 w1333 w1384 w1400 w1424 w1463 w1479] -> w1325
              tunnel: w1324 -> [_ _ _ _ _ _ _]
              tunnel: [_ _ _ _ _ _ TRUE] -> w1321
              tunnel: [ENUM_Auto_State."Idle" ("State") w1329 w1382 w1398 w1406 w1445 ENUM_Auto_State."Shutdown" ("State")] -> w1319
              tunnel: [w1326 w1330 w1380 w1399 w1405 w1444 w1476] -> w1320
              frame "Startup" {
                w1326 = T11[] [enum."Reset All", enum."Reset Time"] items=["No Action", "Reset Time", "Reset All", "Lock Angle", "Drive", "Zero Drive Encoders", "Zero YAW"] ("Actions")
              }
              frame "Idle" {
                n342 = Unbundle By Name(w1334) -> ("Switch Booleans.First Drive"=w1339:bool, "Switch Booleans.Rotated"=w1338:bool, "Switch Booleans.Second Move"=w1337:bool, "Switch Booleans.Arm In position"=w1336:bool, "Switch Booleans.Cube released"=w1335:bool, "Test"=w1341:dbl)
                n343 = Less?(x=w1341, y=2.0) -> (x < y?=w1343:bool)
                n344 = case shown="True" w1339 {
                  tunnel: [ENUM_Auto_State."Cross Line" ("State") w1356] -> w1347
                  tunnel: w1338 -> [_ w1357]
                  tunnel: w1337 -> [_ w1355]
                  tunnel: w1336 -> [_ w1354]
                  tunnel: w1335 -> [_ w1353]
                  tunnel: [94.0 w1351] -> w1332
                  tunnel: [0.0 w1352] -> w1331
                  frame False {
                  }
                  frame True {
                    n345 = case shown="True" w1357 {
                      tunnel: [ENUM_Auto_State."Rotate To Angle" ("State") w1364] -> w1356
                      tunnel: w1355 -> [_ w1363]
                      tunnel: w1354 -> [_ w1365]
                      tunnel: w1353 -> [_ w1361]
                      tunnel: [90.0 0.0] -> w1352
                      tunnel: [0.0 w1362] -> w1351
                      frame False {
                      }
                      frame True {
                        n346 = case shown="False" w1365 {
                          tunnel: [ENUM_Auto_State."position claw arm lift" ("State") w1371] -> w1364
                          tunnel: w1363 -> [_ w1372]
                          tunnel: [0.0 w1370] -> w1362
                          tunnel: w1361 -> [_ w1369]
                          frame False {
                          }
                          frame True {
                            n347 = case shown="True" w1372 {
                              tunnel: [ENUM_Auto_State."Cross Line" ("State") w1376] -> w1371
                              tunnel: [32.0 0.0] -> w1370
                              tunnel: w1369 -> [_ w1375]
                              frame False {
                              }
                              frame True {
                                n348 = case shown="True" w1375 {
                                tunnel: [ENUM_Auto_State."Intake" ("State") ENUM_Auto_State."Shutdown" ("State")] -> w1376
                                frame False {
                                }
                                frame True {
                                }
                                }
                              }
                            }
                          }
                        }
                      }
                    }
                  }
                }
                n349 = Select(t=w1347, s=w1343, f=ENUM_Auto_State."Shutdown" ("State")) -> (s? t:f=w1329:T10)
                n350 = Select(t=ENUM_Auto_Action."Reset All" ("Action"), s=w1343, f=ENUM_Auto_Action."No Action" ("Action")) -> (s? t:f=w1342:T11)
                n351 = Bundle By Name(cluster=w1334, "Encoder Target Position(in)"=w1332, "Target Angle(Degree)"=w1331) -> (w1333:T12)
                n352 = Build Array(w1342) -> (w1330:T11[])
              }
              frame "position claw arm lift" {
                n353 = Unbundle By Name(w1385) -> ("SM_Rotation_Output"=w1388:T1)
                n354 = Equal?(x=w1388, y=ENUM_Rotation_Positon."Switch" ("CMD_SM_Rotation.Rotation Positon")) -> (x = y?=w1386:bool)
                n355 = case shown="True" w1386 {
                  tunnel: [ENUM_Rotation_Positon."Switch" ("CMD_SM_Rotation.Rotation Positon") ENUM_Rotation_Positon."Switch" ("CMD_SM_Rotation.Rotation Positon")] -> w1383
                  tunnel: [ENUM_Auto_State."position claw arm lift" ("State") ENUM_Auto_State."Idle" ("State")] -> w1382
                  tunnel: [FALSE ("Switch Booleans.Arm In position") TRUE ("Switch Booleans.Arm In position")] -> w1381
                  tunnel: [w1389 w1393] -> w1380
                  frame False {
                    w1389 = T11[] [enum."Drive"] items=["No Action", "Reset Time", "Reset All", "Lock Angle", "Drive", "Zero Drive Encoders", "Zero YAW"] ("Actions")
                  }
                  frame True {
                    w1393 = T11[] [enum."No Action"] items=["No Action", "Reset Time", "Reset All", "Lock Angle", "Drive", "Zero Drive Encoders", "Zero YAW"] ("Actions")
                  }
                }
                n356 = Bundle By Name(cluster=w1385, "CMD_SM_Rotation.Rotation Positon"=w1383, "Switch Booleans.Arm In position"=w1381) -> (w1384:T12)
              }
              frame "Intake" {
                n357 = case shown="False" TRUE {
                  tunnel: [ENUM_Auto_State."Intake" ("State") ENUM_Auto_State."Idle" ("State")] -> w1398
                  tunnel: [w1401 w1403] -> w1399
                  frame False {
                    w1401 = T11[] [enum."Drive"] items=["No Action", "Reset Time", "Reset All", "Lock Angle", "Drive", "Zero Drive Encoders", "Zero YAW"] ("Actions")
                  }
                  frame True {
                    w1403 = T11[] [enum."No Action"] items=["No Action", "Reset Time", "Reset All", "Lock Angle", "Drive", "Zero Drive Encoders", "Zero YAW"] ("Actions")
                  }
                }
              }
              frame "Cross Line" {
                n358 = Unbundle By Name(w1425) -> ("Encoder Target Position(in)"=w1407:dbl, "Left Encoder"=w1416:i32, "Right Encoder"=w1415:i32, "Test"=w1427:dbl, "Switch Booleans.First Drive"=w1412:bool)
                n359 = call "EncoderPositionCalc.vi"("PositionTarget(in)"=w1407, "Wheel Size(in)"=6.0, "EncoderCount/Revolution"=4096.0) -> ("PostionTarget(Counts)"=w1414:i32)  [unwired: 8 in]
                n360 = call "AUTO_Encoder_In_Range_Check.vi"("Right Encoder"=w1415, "Left Encoder"=w1416, "PostionTarget(Counts)"=w1414) -> ("Boolean"=w1417:bool)  [unwired: 8 in]
                n361 = Greater?(x=w1427, y=0.5) -> (0:w1429:bool)
                n362 = case shown="False" w1417 {
                  tunnel: [ENUM_Auto_State."Cross Line" ("State") w1438] -> w1418
                  tunnel: w1412 -> [_ w1437]
                  tunnel: [w1433 w1436] -> w1411
                  tunnel: [w1433 w1435] -> w1410
                  frame False {
                    w1433 = FALSE
                  }
                  frame True {
                    n363 = case shown="False" w1437 {
                      tunnel: [ENUM_Auto_State."Idle" ("State") ENUM_Auto_State."Idle" ("State")] -> w1438
                      tunnel: [FALSE w1442] -> w1436
                      tunnel: [TRUE w1442] -> w1435
                      frame False {
                      }
                      frame True {
                        w1442 = TRUE
                      }
                    }
                  }
                }
                n364 = First Call?() -> (First Call?: T/F=w1420:bool)
                n365 = Select(t=w1418, s=w1429, f=ENUM_Auto_State."Idle" ("State")) -> (s? t:f=w1406:T10)
                n366 = Select(t=ENUM_Auto_Action."Drive" ("Action"), s=w1429, f=ENUM_Auto_Action."No Action" ("Action")) -> (s? t:f=w1428:T11)
                n367 = Bundle By Name(cluster=w1425, "Target Angle(Degree)"=0.0, "Steering"=0.0, "Encoder Target Position(in)"=w1407, "Zero Drive Encoders"=w1420, "Zero YAW"=w1420, "CMD_Drive_Data.Drive_Mode"=ENUM_WC_Drive_DriveMode."Motion Profile", "Switch Booleans.First Drive"=w1410, "Switch Booleans.Second Move"=w1411) -> (w1424:T12)
                n368 = Build Array(w1428, ENUM_Auto_Action."Zero Drive Encoders" ("Action"), ENUM_Auto_Action."Lock Angle" ("Action")) -> (w1405:T11[])
              }
              frame "Rotate To Angle" {
                w1455 = 3.0 ("y")
                w1451 = -90.0 ("Target Angle(Degree)")
                n369 = Unbundle By Name(w1464) -> ("YAW"=w1450:dbl, "Test"=w1466:dbl)
                n370 = Greater?(x=w1466, y=0.5) -> (0:w1468:bool)
                n371 = Add(x=w1451, y=w1455) -> (x+y=w1447:dbl)
                n372 = Subtract(x=w1451, y=w1455) -> (x-y=w1446:dbl)
                n373 = In Range and Coerce(upper limit=w1447, x=w1450, lower limit=w1446) -> (In Range?=w1452:bool)  [unwired: 1 out]
                n374 = Select(t=w1450, s=w1452, f=w1451) -> (s? t:f=w1453:dbl)
                n375 = case shown="True" w1452 {
                  tunnel: [ENUM_Auto_State."Rotate To Angle" ("State") ENUM_Auto_State."Idle" ("State")] -> w1457
                  tunnel: [FALSE ("Lock Angle") TRUE ("Lock Angle")] -> w1448
                  frame False {
                  }
                  frame True {
                  }
                }
                n376 = First Call?() -> (First Call?: T/F=w1461:bool)
                n377 = Select(t=w1457, s=w1468, f=ENUM_Auto_State."Idle" ("State")) -> (s? t:f=w1445:T10)
                n378 = Select(t=ENUM_Auto_Action."Drive" ("Action"), s=w1468, f=ENUM_Auto_Action."No Action" ("Action")) -> (s? t:f=w1467:T11)
                n379 = Bundle By Name(cluster=w1464, "Target Angle(Degree)"=w1453, "Steering"=0.0, "Encoder Target Position(in)"=0.0, "Zero Drive Encoders"=w1461, "Zero YAW"=w1461, "CMD_Drive_Data.Drive_Mode"=ENUM_WC_Drive_DriveMode."VBus", "Lock Angle"=TRUE, "Switch Booleans.Rotated"=w1448) -> (w1463:T12)
                n380 = Build Array(w1467, ENUM_Auto_Action."Zero Drive Encoders" ("Action"), ENUM_Auto_Action."Zero YAW" ("Action"), ENUM_Auto_Action."Lock Angle" ("Action")) -> (w1444:T11[])
              }
              frame "Shutdown" {
                w1476 = T11[] [enum."Reset All"] items=["No Action", "Reset Time", "Reset All", "Lock Angle", "Drive", "Zero Drive Encoders", "Zero YAW"] ("Actions")
              }
            }
          }
          frame "Scale" {
            n381 = case shown="\"Rotate To Angle\"" w1484 {
              tunnel: w1483 -> [w1489 w1495 w1546 w1561 w1586 w1625 w1640]
              tunnel: [w1489 w1494 w1545 w1561 w1585 w1624 w1640] -> w1486
              tunnel: w1485 -> [_ _ _ _ _ _ _]
              tunnel: [_ _ _ _ _ _ TRUE] -> w1482
              tunnel: [ENUM_Auto_State."Idle" ("State") w1490 w1543 w1559 w1567 w1606 ENUM_Auto_State."Shutdown" ("State")] -> w1480
              tunnel: [w1487 w1491 w1541 w1560 w1566 w1605 w1637] -> w1481
              frame "Startup" {
                w1487 = T11[] [enum."Reset All", enum."Reset Time"] items=["No Action", "Reset Time", "Reset All", "Lock Angle", "Drive", "Zero Drive Encoders", "Zero YAW"] ("Actions")
              }
              frame "Idle" {
                n382 = Unbundle By Name(w1495) -> ("Switch Booleans.First Drive"=w1500:bool, "Switch Booleans.Rotated"=w1499:bool, "Switch Booleans.Second Move"=w1498:bool, "Switch Booleans.Arm In position"=w1497:bool, "Switch Booleans.Cube released"=w1496:bool, "Test"=w1502:dbl)
                n383 = Less?(x=w1502, y=2.0) -> (x < y?=w1504:bool)
                n384 = case shown="True" w1500 {
                  tunnel: [ENUM_Auto_State."Cross Line" ("State") w1517] -> w1508
                  tunnel: w1499 -> [_ w1518]
                  tunnel: w1498 -> [_ w1516]
                  tunnel: w1497 -> [_ w1515]
                  tunnel: w1496 -> [_ w1514]
                  tunnel: [94.0 w1512] -> w1493
                  tunnel: [0.0 w1513] -> w1492
                  frame False {
                  }
                  frame True {
                    n385 = case shown="True" w1518 {
                      tunnel: [ENUM_Auto_State."Rotate To Angle" ("State") w1525] -> w1517
                      tunnel: w1516 -> [_ w1524]
                      tunnel: w1515 -> [_ w1526]
                      tunnel: w1514 -> [_ w1522]
                      tunnel: [90.0 0.0] -> w1513
                      tunnel: [0.0 w1523] -> w1512
                      frame False {
                      }
                      frame True {
                        n386 = case shown="False" w1526 {
                          tunnel: [ENUM_Auto_State."position claw arm lift" ("State") w1532] -> w1525
                          tunnel: w1524 -> [_ w1533]
                          tunnel: [0.0 w1531] -> w1523
                          tunnel: w1522 -> [_ w1530]
                          frame False {
                          }
                          frame True {
                            n387 = case shown="True" w1533 {
                              tunnel: [ENUM_Auto_State."Cross Line" ("State") w1537] -> w1532
                              tunnel: [32.0 0.0] -> w1531
                              tunnel: w1530 -> [_ w1536]
                              frame False {
                              }
                              frame True {
                                n388 = case shown="True" w1536 {
                                tunnel: [ENUM_Auto_State."Intake" ("State") ENUM_Auto_State."Shutdown" ("State")] -> w1537
                                frame False {
                                }
                                frame True {
                                }
                                }
                              }
                            }
                          }
                        }
                      }
                    }
                  }
                }
                n389 = Select(t=w1508, s=w1504, f=ENUM_Auto_State."Shutdown" ("State")) -> (s? t:f=w1490:T10)
                n390 = Select(t=ENUM_Auto_Action."Reset All" ("Action"), s=w1504, f=ENUM_Auto_Action."No Action" ("Action")) -> (s? t:f=w1503:T11)
                n391 = Bundle By Name(cluster=w1495, "Encoder Target Position(in)"=w1493, "Target Angle(Degree)"=w1492) -> (w1494:T12)
                n392 = Build Array(w1503) -> (w1491:T11[])
              }
              frame "position claw arm lift" {
                n393 = Unbundle By Name(w1546) -> ("SM_Rotation_Output"=w1549:T1)
                n394 = Equal?(x=w1549, y=ENUM_Rotation_Positon."Switch" ("CMD_SM_Rotation.Rotation Positon")) -> (x = y?=w1547:bool)
                n395 = case shown="True" w1547 {
                  tunnel: [ENUM_Rotation_Positon."Switch" ("CMD_SM_Rotation.Rotation Positon") ENUM_Rotation_Positon."Switch" ("CMD_SM_Rotation.Rotation Positon")] -> w1544
                  tunnel: [ENUM_Auto_State."position claw arm lift" ("State") ENUM_Auto_State."Idle" ("State")] -> w1543
                  tunnel: [FALSE ("Switch Booleans.Arm In position") TRUE ("Switch Booleans.Arm In position")] -> w1542
                  tunnel: [w1550 w1554] -> w1541
                  frame False {
                    w1550 = T11[] [enum."Drive"] items=["No Action", "Reset Time", "Reset All", "Lock Angle", "Drive", "Zero Drive Encoders", "Zero YAW"] ("Actions")
                  }
                  frame True {
                    w1554 = T11[] [enum."No Action"] items=["No Action", "Reset Time", "Reset All", "Lock Angle", "Drive", "Zero Drive Encoders", "Zero YAW"] ("Actions")
                  }
                }
                n396 = Bundle By Name(cluster=w1546, "CMD_SM_Rotation.Rotation Positon"=w1544, "Switch Booleans.Arm In position"=w1542) -> (w1545:T12)
              }
              frame "Intake" {
                n397 = case shown="False" TRUE {
                  tunnel: [ENUM_Auto_State."Intake" ("State") ENUM_Auto_State."Idle" ("State")] -> w1559
                  tunnel: [w1562 w1564] -> w1560
                  frame False {
                    w1562 = T11[] [enum."Drive"] items=["No Action", "Reset Time", "Reset All", "Lock Angle", "Drive", "Zero Drive Encoders", "Zero YAW"] ("Actions")
                  }
                  frame True {
                    w1564 = T11[] [enum."No Action"] items=["No Action", "Reset Time", "Reset All", "Lock Angle", "Drive", "Zero Drive Encoders", "Zero YAW"] ("Actions")
                  }
                }
              }
              frame "Cross Line" {
                n398 = Unbundle By Name(w1586) -> ("Encoder Target Position(in)"=w1568:dbl, "Left Encoder"=w1577:i32, "Right Encoder"=w1576:i32, "Test"=w1588:dbl, "Switch Booleans.First Drive"=w1573:bool)
                n399 = call "EncoderPositionCalc.vi"("PositionTarget(in)"=w1568, "Wheel Size(in)"=6.0, "EncoderCount/Revolution"=4096.0) -> ("PostionTarget(Counts)"=w1575:i32)  [unwired: 8 in]
                n400 = call "AUTO_Encoder_In_Range_Check.vi"("Right Encoder"=w1576, "Left Encoder"=w1577, "PostionTarget(Counts)"=w1575) -> ("Boolean"=w1578:bool)  [unwired: 8 in]
                n401 = Greater?(x=w1588, y=0.5) -> (0:w1590:bool)
                n402 = case shown="False" w1578 {
                  tunnel: [ENUM_Auto_State."Cross Line" ("State") w1599] -> w1579
                  tunnel: w1573 -> [_ w1598]
                  tunnel: [w1594 w1597] -> w1572
                  tunnel: [w1594 w1596] -> w1571
                  frame False {
                    w1594 = FALSE
                  }
                  frame True {
                    n403 = case shown="False" w1598 {
                      tunnel: [ENUM_Auto_State."Idle" ("State") ENUM_Auto_State."Idle" ("State")] -> w1599
                      tunnel: [FALSE w1603] -> w1597
                      tunnel: [TRUE w1603] -> w1596
                      frame False {
                      }
                      frame True {
                        w1603 = TRUE
                      }
                    }
                  }
                }
                n404 = First Call?() -> (First Call?: T/F=w1581:bool)
                n405 = Select(t=w1579, s=w1590, f=ENUM_Auto_State."Idle" ("State")) -> (s? t:f=w1567:T10)
                n406 = Select(t=ENUM_Auto_Action."Drive" ("Action"), s=w1590, f=ENUM_Auto_Action."No Action" ("Action")) -> (s? t:f=w1589:T11)
                n407 = Bundle By Name(cluster=w1586, "Target Angle(Degree)"=0.0, "Steering"=0.0, "Encoder Target Position(in)"=w1568, "Zero Drive Encoders"=w1581, "Zero YAW"=w1581, "CMD_Drive_Data.Drive_Mode"=ENUM_WC_Drive_DriveMode."Motion Profile", "Switch Booleans.First Drive"=w1571, "Switch Booleans.Second Move"=w1572) -> (w1585:T12)
                n408 = Build Array(w1589, ENUM_Auto_Action."Zero Drive Encoders" ("Action"), ENUM_Auto_Action."Lock Angle" ("Action")) -> (w1566:T11[])
              }
              frame "Rotate To Angle" {
                w1616 = 3.0 ("y")
                w1612 = -90.0 ("Target Angle(Degree)")
                n409 = Unbundle By Name(w1625) -> ("YAW"=w1611:dbl, "Test"=w1627:dbl)
                n410 = Greater?(x=w1627, y=0.5) -> (0:w1629:bool)
                n411 = Add(x=w1612, y=w1616) -> (x+y=w1608:dbl)
                n412 = Subtract(x=w1612, y=w1616) -> (x-y=w1607:dbl)
                n413 = In Range and Coerce(upper limit=w1608, x=w1611, lower limit=w1607) -> (In Range?=w1613:bool)  [unwired: 1 out]
                n414 = Select(t=w1611, s=w1613, f=w1612) -> (s? t:f=w1614:dbl)
                n415 = case shown="True" w1613 {
                  tunnel: [ENUM_Auto_State."Rotate To Angle" ("State") ENUM_Auto_State."Idle" ("State")] -> w1618
                  tunnel: [FALSE ("Lock Angle") TRUE ("Lock Angle")] -> w1609
                  frame False {
                  }
                  frame True {
                  }
                }
                n416 = First Call?() -> (First Call?: T/F=w1622:bool)
                n417 = Select(t=w1618, s=w1629, f=ENUM_Auto_State."Idle" ("State")) -> (s? t:f=w1606:T10)
                n418 = Select(t=ENUM_Auto_Action."Drive" ("Action"), s=w1629, f=ENUM_Auto_Action."No Action" ("Action")) -> (s? t:f=w1628:T11)
                n419 = Bundle By Name(cluster=w1625, "Target Angle(Degree)"=w1614, "Steering"=0.0, "Encoder Target Position(in)"=0.0, "Zero Drive Encoders"=w1622, "Zero YAW"=w1622, "CMD_Drive_Data.Drive_Mode"=ENUM_WC_Drive_DriveMode."VBus", "Lock Angle"=TRUE, "Switch Booleans.Rotated"=w1609) -> (w1624:T12)
                n420 = Build Array(w1628, ENUM_Auto_Action."Zero Drive Encoders" ("Action"), ENUM_Auto_Action."Zero YAW" ("Action"), ENUM_Auto_Action."Lock Angle" ("Action")) -> (w1605:T11[])
              }
              frame "Shutdown" {
                w1637 = T11[] [enum."Reset All"] items=["No Action", "Reset Time", "Reset All", "Lock Angle", "Drive", "Zero Drive Encoders", "Zero YAW"] ("Actions")
              }
            }
          }
          frame "Scale And Switch" {
            n421 = case shown="\"Rotate To Angle\"" w1645 {
              tunnel: w1644 -> [w1650 w1656 w1707 w1722 w1747 w1786 w1801]
              tunnel: [w1650 w1655 w1706 w1722 w1746 w1785 w1801] -> w1647
              tunnel: w1646 -> [_ _ _ _ _ _ _]
              tunnel: [_ _ _ _ _ _ TRUE] -> w1643
              tunnel: [ENUM_Auto_State."Idle" ("State") w1651 w1704 w1720 w1728 w1767 ENUM_Auto_State."Shutdown" ("State")] -> w1641
              tunnel: [w1648 w1652 w1702 w1721 w1727 w1766 w1798] -> w1642
              frame "Startup" {
                w1648 = T11[] [enum."Reset All", enum."Reset Time"] items=["No Action", "Reset Time", "Reset All", "Lock Angle", "Drive", "Zero Drive Encoders", "Zero YAW"] ("Actions")
              }
              frame "Idle" {
                n422 = Unbundle By Name(w1656) -> ("Switch Booleans.First Drive"=w1661:bool, "Switch Booleans.Rotated"=w1660:bool, "Switch Booleans.Second Move"=w1659:bool, "Switch Booleans.Arm In position"=w1658:bool, "Switch Booleans.Cube released"=w1657:bool, "Test"=w1663:dbl)
                n423 = Less?(x=w1663, y=2.0) -> (x < y?=w1665:bool)
                n424 = case shown="True" w1661 {
                  tunnel: [ENUM_Auto_State."Cross Line" ("State") w1678] -> w1669
                  tunnel: w1660 -> [_ w1679]
                  tunnel: w1659 -> [_ w1677]
                  tunnel: w1658 -> [_ w1676]
                  tunnel: w1657 -> [_ w1675]
                  tunnel: [94.0 w1673] -> w1654
                  tunnel: [0.0 w1674] -> w1653
                  frame False {
                  }
                  frame True {
                    n425 = case shown="True" w1679 {
                      tunnel: [ENUM_Auto_State."Rotate To Angle" ("State") w1686] -> w1678
                      tunnel: w1677 -> [_ w1685]
                      tunnel: w1676 -> [_ w1687]
                      tunnel: w1675 -> [_ w1683]
                      tunnel: [90.0 0.0] -> w1674
                      tunnel: [0.0 w1684] -> w1673
                      frame False {
                      }
                      frame True {
                        n426 = case shown="False" w1687 {
                          tunnel: [ENUM_Auto_State."position claw arm lift" ("State") w1693] -> w1686
                          tunnel: w1685 -> [_ w1694]
                          tunnel: [0.0 w1692] -> w1684
                          tunnel: w1683 -> [_ w1691]
                          frame False {
                          }
                          frame True {
                            n427 = case shown="True" w1694 {
                              tunnel: [ENUM_Auto_State."Cross Line" ("State") w1698] -> w1693
                              tunnel: [32.0 0.0] -> w1692
                              tunnel: w1691 -> [_ w1697]
                              frame False {
                              }
                              frame True {
                                n428 = case shown="True" w1697 {
                                tunnel: [ENUM_Auto_State."Intake" ("State") ENUM_Auto_State."Shutdown" ("State")] -> w1698
                                frame False {
                                }
                                frame True {
                                }
                                }
                              }
                            }
                          }
                        }
                      }
                    }
                  }
                }
                n429 = Select(t=w1669, s=w1665, f=ENUM_Auto_State."Shutdown" ("State")) -> (s? t:f=w1651:T10)
                n430 = Select(t=ENUM_Auto_Action."Reset All" ("Action"), s=w1665, f=ENUM_Auto_Action."No Action" ("Action")) -> (s? t:f=w1664:T11)
                n431 = Bundle By Name(cluster=w1656, "Encoder Target Position(in)"=w1654, "Target Angle(Degree)"=w1653) -> (w1655:T12)
                n432 = Build Array(w1664) -> (w1652:T11[])
              }
              frame "position claw arm lift" {
                n433 = Unbundle By Name(w1707) -> ("SM_Rotation_Output"=w1710:T1)
                n434 = Equal?(x=w1710, y=ENUM_Rotation_Positon."Switch" ("CMD_SM_Rotation.Rotation Positon")) -> (x = y?=w1708:bool)
                n435 = case shown="True" w1708 {
                  tunnel: [ENUM_Rotation_Positon."Switch" ("CMD_SM_Rotation.Rotation Positon") ENUM_Rotation_Positon."Switch" ("CMD_SM_Rotation.Rotation Positon")] -> w1705
                  tunnel: [ENUM_Auto_State."position claw arm lift" ("State") ENUM_Auto_State."Idle" ("State")] -> w1704
                  tunnel: [FALSE ("Switch Booleans.Arm In position") TRUE ("Switch Booleans.Arm In position")] -> w1703
                  tunnel: [w1711 w1715] -> w1702
                  frame False {
                    w1711 = T11[] [enum."Drive"] items=["No Action", "Reset Time", "Reset All", "Lock Angle", "Drive", "Zero Drive Encoders", "Zero YAW"] ("Actions")
                  }
                  frame True {
                    w1715 = T11[] [enum."No Action"] items=["No Action", "Reset Time", "Reset All", "Lock Angle", "Drive", "Zero Drive Encoders", "Zero YAW"] ("Actions")
                  }
                }
                n436 = Bundle By Name(cluster=w1707, "CMD_SM_Rotation.Rotation Positon"=w1705, "Switch Booleans.Arm In position"=w1703) -> (w1706:T12)
              }
              frame "Intake" {
                n437 = case shown="False" TRUE {
                  tunnel: [ENUM_Auto_State."Intake" ("State") ENUM_Auto_State."Idle" ("State")] -> w1720
                  tunnel: [w1723 w1725] -> w1721
                  frame False {
                    w1723 = T11[] [enum."Drive"] items=["No Action", "Reset Time", "Reset All", "Lock Angle", "Drive", "Zero Drive Encoders", "Zero YAW"] ("Actions")
                  }
                  frame True {
                    w1725 = T11[] [enum."No Action"] items=["No Action", "Reset Time", "Reset All", "Lock Angle", "Drive", "Zero Drive Encoders", "Zero YAW"] ("Actions")
                  }
                }
              }
              frame "Cross Line" {
                n438 = Unbundle By Name(w1747) -> ("Encoder Target Position(in)"=w1729:dbl, "Left Encoder"=w1738:i32, "Right Encoder"=w1737:i32, "Test"=w1749:dbl, "Switch Booleans.First Drive"=w1734:bool)
                n439 = call "EncoderPositionCalc.vi"("PositionTarget(in)"=w1729, "Wheel Size(in)"=6.0, "EncoderCount/Revolution"=4096.0) -> ("PostionTarget(Counts)"=w1736:i32)  [unwired: 8 in]
                n440 = call "AUTO_Encoder_In_Range_Check.vi"("Right Encoder"=w1737, "Left Encoder"=w1738, "PostionTarget(Counts)"=w1736) -> ("Boolean"=w1739:bool)  [unwired: 8 in]
                n441 = Greater?(x=w1749, y=0.5) -> (0:w1751:bool)
                n442 = case shown="False" w1739 {
                  tunnel: [ENUM_Auto_State."Cross Line" ("State") w1760] -> w1740
                  tunnel: w1734 -> [_ w1759]
                  tunnel: [w1755 w1758] -> w1733
                  tunnel: [w1755 w1757] -> w1732
                  frame False {
                    w1755 = FALSE
                  }
                  frame True {
                    n443 = case shown="False" w1759 {
                      tunnel: [ENUM_Auto_State."Idle" ("State") ENUM_Auto_State."Idle" ("State")] -> w1760
                      tunnel: [FALSE w1764] -> w1758
                      tunnel: [TRUE w1764] -> w1757
                      frame False {
                      }
                      frame True {
                        w1764 = TRUE
                      }
                    }
                  }
                }
                n444 = First Call?() -> (First Call?: T/F=w1742:bool)
                n445 = Select(t=w1740, s=w1751, f=ENUM_Auto_State."Idle" ("State")) -> (s? t:f=w1728:T10)
                n446 = Select(t=ENUM_Auto_Action."Drive" ("Action"), s=w1751, f=ENUM_Auto_Action."No Action" ("Action")) -> (s? t:f=w1750:T11)
                n447 = Bundle By Name(cluster=w1747, "Target Angle(Degree)"=0.0, "Steering"=0.0, "Encoder Target Position(in)"=w1729, "Zero Drive Encoders"=w1742, "Zero YAW"=w1742, "CMD_Drive_Data.Drive_Mode"=ENUM_WC_Drive_DriveMode."Motion Profile", "Switch Booleans.First Drive"=w1732, "Switch Booleans.Second Move"=w1733) -> (w1746:T12)
                n448 = Build Array(w1750, ENUM_Auto_Action."Zero Drive Encoders" ("Action"), ENUM_Auto_Action."Lock Angle" ("Action")) -> (w1727:T11[])
              }
              frame "Rotate To Angle" {
                w1777 = 3.0 ("y")
                w1773 = -90.0 ("Target Angle(Degree)")
                n449 = Unbundle By Name(w1786) -> ("YAW"=w1772:dbl, "Test"=w1788:dbl)
                n450 = Greater?(x=w1788, y=0.5) -> (0:w1790:bool)
                n451 = Add(x=w1773, y=w1777) -> (x+y=w1769:dbl)
                n452 = Subtract(x=w1773, y=w1777) -> (x-y=w1768:dbl)
                n453 = In Range and Coerce(upper limit=w1769, x=w1772, lower limit=w1768) -> (In Range?=w1774:bool)  [unwired: 1 out]
                n454 = Select(t=w1772, s=w1774, f=w1773) -> (s? t:f=w1775:dbl)
                n455 = case shown="True" w1774 {
                  tunnel: [ENUM_Auto_State."Rotate To Angle" ("State") ENUM_Auto_State."Idle" ("State")] -> w1779
                  tunnel: [FALSE ("Lock Angle") TRUE ("Lock Angle")] -> w1770
                  frame False {
                  }
                  frame True {
                  }
                }
                n456 = First Call?() -> (First Call?: T/F=w1783:bool)
                n457 = Select(t=w1779, s=w1790, f=ENUM_Auto_State."Idle" ("State")) -> (s? t:f=w1767:T10)
                n458 = Select(t=ENUM_Auto_Action."Drive" ("Action"), s=w1790, f=ENUM_Auto_Action."No Action" ("Action")) -> (s? t:f=w1789:T11)
                n459 = Bundle By Name(cluster=w1786, "Target Angle(Degree)"=w1775, "Steering"=0.0, "Encoder Target Position(in)"=0.0, "Zero Drive Encoders"=w1783, "Zero YAW"=w1783, "CMD_Drive_Data.Drive_Mode"=ENUM_WC_Drive_DriveMode."VBus", "Lock Angle"=TRUE, "Switch Booleans.Rotated"=w1770) -> (w1785:T12)
                n460 = Build Array(w1789, ENUM_Auto_Action."Zero Drive Encoders" ("Action"), ENUM_Auto_Action."Zero YAW" ("Action"), ENUM_Auto_Action."Lock Angle" ("Action")) -> (w1766:T11[])
              }
              frame "Shutdown" {
                w1798 = T11[] [enum."Reset All"] items=["No Action", "Reset Time", "Reset All", "Lock Angle", "Drive", "Zero Drive Encoders", "Zero YAW"] ("Actions")
              }
            }
          }
          frame "Cross Line" {
            n461 = case shown="\"Rotate To Angle\"" w1805 {
              tunnel: w1804 -> [w1811 w1814 w1842 w1871 w1886 w1890 w1894]
              tunnel: [w1811 w1813 w1841 w1870 w1886 w1890 w1894] -> w1808
              tunnel: [ENUM_Auto_State."Idle" ("State") w1824 w1851 w1880 ENUM_Auto_State."Shutdown" ("State") ENUM_Auto_State."Shutdown" ("State") ENUM_Auto_State."Shutdown" ("State")] -> w1807
              tunnel: [w1810 w1817 w1845 w1874 w1884 w1888 w1892] -> w1803
              tunnel: w1806 -> [_ _ _ _ _ _ _]
              tunnel: [_ _ _ _ TRUE TRUE TRUE] -> w1802
              frame "Startup" {
                w1810 = T11[] [enum."Reset All", enum."Reset Time"] items=["No Action", "Reset Time", "Reset All", "Lock Angle", "Drive", "Zero Drive Encoders", "Zero YAW"] ("Actions")
              }
              frame "Idle" {
                n462 = Unbundle By Name(w1814) -> ("Test"=w1816:dbl)
                n463 = Less?(x=w1816, y=2.0) -> (x < y?=w1819:bool)
                n464 = Select(t=ENUM_Auto_State."Cross Line" ("State"), s=w1819, f=ENUM_Auto_State."Shutdown" ("State")) -> (s? t:f=w1824:T10)
                n465 = Select(t=ENUM_Auto_Action."Reset All" ("Action"), s=w1819, f=ENUM_Auto_Action."No Action" ("Action")) -> (s? t:f=w1818:T11)
                n466 = Build Array(w1818) -> (w1817:T11[])
                n467 = Bundle By Name(cluster=w1814, "Encoder Target Position(in)"=120.0) -> (w1813:T12)
              }
              frame "Cross Line" {
                w1827 = 120.0 ("Encoder Target Position(in)")
                n468 = Unbundle By Name(w1842) -> ("Zero YAW"=w1833:bool, "Left Encoder"=w1831:i32, "Right Encoder"=w1830:i32, "Test"=w1844:dbl)
                n469 = Greater?(x=w1844, y=0.5) -> (0:w1847:bool)
                n470 = call "EncoderPositionCalc.vi"("PositionTarget(in)"=4092.0, "Wheel Size(in)"=6.0, "EncoderCount/Revolution"=w1827) -> ("PostionTarget(Counts)"=w1828:i32)  [unwired: 8 in]
                n471 = call "AUTO_Encoder_In_Range_Check.vi"("Right Encoder"=w1830, "Left Encoder"=w1831, "PostionTarget(Counts)"=w1828) -> ("Boolean"=w1829:bool)  [unwired: 8 in]
                n472 = case shown="True" w1829 {
                  tunnel: [ENUM_Auto_State."Cross Line" ("State") ENUM_Auto_State."Shutdown" ("State")] -> w1832
                  frame False {
                  }
                  frame True {
                  }
                }
                n473 = First Call?() -> (First Call?: T/F=w1834:bool)
                n474 = Select(t=w1832, s=w1847, f=ENUM_Auto_State."Idle" ("State")) -> (s? t:f=w1851:T10)
                n475 = Select(t=ENUM_Auto_Action."Drive" ("Action"), s=w1847, f=ENUM_Auto_Action."No Action" ("Action")) -> (s? t:f=w1846:T11)
                n476 = Bundle By Name(cluster=w1842, "Target Angle(Degree)"=0.0, "Steering"=0.0, "Encoder Target Position(in)"=w1827, "Zero Drive Encoders"=w1834, "Zero YAW"=w1833, "CMD_Drive_Data.Drive_Mode"=ENUM_WC_Drive_DriveMode."Motion Profile") -> (w1841:T12)
                n477 = Build Array(w1846, ENUM_Auto_Action."Zero Drive Encoders" ("Action"), ENUM_Auto_Action."Zero YAW" ("Action"), ENUM_Auto_Action."Lock Angle" ("Action")) -> (w1845:T11[])
              }
              frame "Rotate To Angle" {
                w1859 = 3.0 ("y")
                w1855 = 180.0 ("Target Angle(Degree)")
                n478 = Unbundle By Name(w1871) -> ("YAW"=w1854:dbl, "Test"=w1873:dbl)
                n479 = Greater?(x=w1873, y=0.5) -> (0:w1876:bool)
                n480 = Add(x=w1855, y=w1859) -> (x+y=w1861:dbl)
                n481 = Subtract(x=w1855, y=w1859) -> (x-y=w1860:dbl)
                n482 = In Range and Coerce(upper limit=w1861, x=w1854, lower limit=w1860) -> (In Range?=w1856:bool)  [unwired: 1 out]
                n483 = Select(t=w1854, s=w1856, f=w1855) -> (s? t:f=w1857:dbl)
                n484 = case shown="False" w1856 {
                  tunnel: [ENUM_Auto_State."Cross Line" ("State") ENUM_Auto_State."Cross Line" ("State")] -> w1863
                  frame False {
                  }
                  frame True {
                  }
                }
                n485 = First Call?() -> (First Call?: T/F=w1867:bool)
                n486 = Select(t=w1863, s=w1876, f=ENUM_Auto_State."Idle" ("State")) -> (s? t:f=w1880:T10)
                n487 = Select(t=ENUM_Auto_Action."Drive" ("Action"), s=w1876, f=ENUM_Auto_Action."No Action" ("Action")) -> (s? t:f=w1875:T11)
                n488 = Bundle By Name(cluster=w1871, "Target Angle(Degree)"=w1857, "Steering"=0.0, "Encoder Target Position(in)"=0.0, "Zero Drive Encoders"=w1867, "Zero YAW"=w1867, "CMD_Drive_Data.Drive_Mode"=ENUM_WC_Drive_DriveMode."VBus", "Lock Angle"=TRUE) -> (w1870:T12)
                n489 = Build Array(w1875, ENUM_Auto_Action."Zero Drive Encoders" ("Action"), ENUM_Auto_Action."Zero YAW" ("Action"), ENUM_Auto_Action."Lock Angle" ("Action")) -> (w1874:T11[])
              }
              frame "Shutdown" {
                w1884 = T11[] [enum."Reset All"] items=["No Action", "Reset Time", "Reset All", "Lock Angle", "Drive", "Zero Drive Encoders", "Zero YAW"] ("Actions")
              }
              frame "position claw arm lift" {
                w1888 = T11[] [enum."Reset All"] items=["No Action", "Reset Time", "Reset All", "Lock Angle", "Drive", "Zero Drive Encoders", "Zero YAW"] ("Actions")
              }
              frame "Intake" {
                w1892 = T11[] [enum."Reset All"] items=["No Action", "Reset Time", "Reset All", "Lock Angle", "Drive", "Zero Drive Encoders", "Zero YAW"] ("Actions")
              }
            }
          }
          frame "No Movement" {
            n490 = case shown="\"Intake\"" w1898 {
              tunnel: w1897 -> [w1904 w1907 w1920 w1923 w1926 w1929 w1933]
              tunnel: [w1904 w1906 w1920 w1923 w1926 w1929 w1933] -> w1901
              tunnel: [ENUM_Auto_State."Idle" ("State") w1917 ENUM_Auto_State."Shutdown" ("State") ENUM_Auto_State."Idle" ("State") ENUM_Auto_State."Idle" ("State") ENUM_Auto_State."Idle" ("State") ENUM_Auto_State."Shutdown" ("State")] -> w1900
              tunnel: [w1903 w1910 w1919 w1921 w1924 w1927 w1931] -> w1896
              tunnel: w1899 -> [_ _ _ _ _ _ _]
              tunnel: [_ _ _ _ _ _ TRUE] -> w1895
              frame "Startup" {
                w1903 = T11[] [enum."Reset All", enum."Reset Time"] items=["No Action", "Reset Time", "Reset All", "Lock Angle", "Drive", "Zero Drive Encoders", "Zero YAW"] ("Actions")
              }
              frame "Idle" {
                n491 = Unbundle By Name(w1907) -> ("Test"=w1909:dbl)
                n492 = Less?(x=w1909, y=2.0) -> (x < y?=w1912:bool)
                n493 = Select(t=ENUM_Auto_State."Idle" ("State"), s=w1912, f=ENUM_Auto_State."Shutdown" ("State")) -> (s? t:f=w1917:T10)
                n494 = Select(t=ENUM_Auto_Action."Reset All" ("Action"), s=w1912, f=ENUM_Auto_Action."No Action" ("Action")) -> (s? t:f=w1911:T11)
                n495 = Build Array(w1911) -> (w1910:T11[])
                n496 = Bundle By Name(cluster=w1907, "Encoder Target Position(in)"=120.0) -> (w1906:T12)
              }
              frame "Cross Line" {
                w1919 = T11[] [enum."No Action"] items=["No Action", "Reset Time", "Reset All", "Lock Angle", "Drive", "Zero Drive Encoders", "Zero YAW"] ("Actions")
              }
              frame "Rotate To Angle" {
                w1921 = T11[] [enum."No Action"] items=["No Action", "Reset Time", "Reset All", "Lock Angle", "Drive", "Zero Drive Encoders", "Zero YAW"] ("Actions")
              }
              frame "Intake" {
                w1924 = T11[] [enum."No Action"] items=["No Action", "Reset Time", "Reset All", "Lock Angle", "Drive", "Zero Drive Encoders", "Zero YAW"] ("Actions")
              }
              frame "position claw arm lift" {
                w1927 = T11[] [enum."No Action"] items=["No Action", "Reset Time", "Reset All", "Lock Angle", "Drive", "Zero Drive Encoders", "Zero YAW"] ("Actions")
              }
              frame "Shutdown" {
                w1931 = T11[] [enum."Reset All"] items=["No Action", "Reset Time", "Reset All", "Lock Angle", "Drive", "Zero Drive Encoders", "Zero YAW"] ("Actions")
              }
            }
          }
        }
        n497 = Bundle By Name(cluster=w1317, "Previous State"=w1314, "State"=w1316) -> (w1318:T12)
      }
      frame "LLL" {
        n498 = case shown="\"Cross Line\"" w1934 {
          tunnel: [w1949 w2110 w2271 w2432 w2523] -> w1941
          tunnel: [w1943 w2104 w2265 w2431 w2522] -> w1940
          tunnel: w1939 -> [w1948 w2109 w2270 w2430 w2521]
          tunnel: w1938 -> [w1947 w2108 w2269 w2429 w2520]
          tunnel: w1937 -> [w1946 w2107 w2268 w2428 w2519]
          tunnel: [w1944 w2105 w2266 w2427 w2518] -> w1936
          tunnel: [w1945 w2106 w2267 w2426 w2517] -> w1935
          frame "Switch" {
            n499 = case shown="\"Rotate To Angle\"" w1947 {
              tunnel: w1946 -> [w1952 w1958 w2009 w2024 w2049 w2088 w2103]
              tunnel: [w1952 w1957 w2008 w2024 w2048 w2087 w2103] -> w1949
              tunnel: w1948 -> [_ _ _ _ _ _ _]
              tunnel: [_ _ _ _ _ _ TRUE] -> w1945
              tunnel: [ENUM_Auto_State."Idle" ("State") w1953 w2006 w2022 w2030 w2069 ENUM_Auto_State."Shutdown" ("State")] -> w1943
              tunnel: [w1950 w1954 w2004 w2023 w2029 w2068 w2100] -> w1944
              frame "Startup" {
                w1950 = T11[] [enum."Reset All", enum."Reset Time"] items=["No Action", "Reset Time", "Reset All", "Lock Angle", "Drive", "Zero Drive Encoders", "Zero YAW"] ("Actions")
              }
              frame "Idle" {
                n500 = Unbundle By Name(w1958) -> ("Switch Booleans.First Drive"=w1963:bool, "Switch Booleans.Rotated"=w1962:bool, "Switch Booleans.Second Move"=w1961:bool, "Switch Booleans.Arm In position"=w1960:bool, "Switch Booleans.Cube released"=w1959:bool, "Test"=w1965:dbl)
                n501 = Less?(x=w1965, y=2.0) -> (x < y?=w1967:bool)
                n502 = case shown="True" w1963 {
                  tunnel: [ENUM_Auto_State."Cross Line" ("State") w1980] -> w1971
                  tunnel: w1962 -> [_ w1981]
                  tunnel: w1961 -> [_ w1979]
                  tunnel: w1960 -> [_ w1978]
                  tunnel: w1959 -> [_ w1977]
                  tunnel: [94.0 w1975] -> w1956
                  tunnel: [0.0 w1976] -> w1955
                  frame False {
                  }
                  frame True {
                    n503 = case shown="True" w1981 {
                      tunnel: [ENUM_Auto_State."Rotate To Angle" ("State") w1988] -> w1980
                      tunnel: w1979 -> [_ w1987]
                      tunnel: w1978 -> [_ w1989]
                      tunnel: w1977 -> [_ w1985]
                      tunnel: [90.0 0.0] -> w1976
                      tunnel: [0.0 w1986] -> w1975
                      frame False {
                      }
                      frame True {
                        n504 = case shown="False" w1989 {
                          tunnel: [ENUM_Auto_State."position claw arm lift" ("State") w1995] -> w1988
                          tunnel: w1987 -> [_ w1996]
                          tunnel: [0.0 w1994] -> w1986
                          tunnel: w1985 -> [_ w1993]
                          frame False {
                          }
                          frame True {
                            n505 = case shown="True" w1996 {
                              tunnel: [ENUM_Auto_State."Cross Line" ("State") w2000] -> w1995
                              tunnel: [32.0 0.0] -> w1994
                              tunnel: w1993 -> [_ w1999]
                              frame False {
                              }
                              frame True {
                                n506 = case shown="True" w1999 {
                                tunnel: [ENUM_Auto_State."Intake" ("State") ENUM_Auto_State."Shutdown" ("State")] -> w2000
                                frame False {
                                }
                                frame True {
                                }
                                }
                              }
                            }
                          }
                        }
                      }
                    }
                  }
                }
                n507 = Select(t=w1971, s=w1967, f=ENUM_Auto_State."Shutdown" ("State")) -> (s? t:f=w1953:T10)
                n508 = Select(t=ENUM_Auto_Action."Reset All" ("Action"), s=w1967, f=ENUM_Auto_Action."No Action" ("Action")) -> (s? t:f=w1966:T11)
                n509 = Bundle By Name(cluster=w1958, "Encoder Target Position(in)"=w1956, "Target Angle(Degree)"=w1955) -> (w1957:T12)
                n510 = Build Array(w1966) -> (w1954:T11[])
              }
              frame "position claw arm lift" {
                n511 = Unbundle By Name(w2009) -> ("SM_Rotation_Output"=w2012:T1)
                n512 = Equal?(x=w2012, y=ENUM_Rotation_Positon."Switch" ("CMD_SM_Rotation.Rotation Positon")) -> (x = y?=w2010:bool)
                n513 = case shown="True" w2010 {
                  tunnel: [ENUM_Rotation_Positon."Switch" ("CMD_SM_Rotation.Rotation Positon") ENUM_Rotation_Positon."Switch" ("CMD_SM_Rotation.Rotation Positon")] -> w2007
                  tunnel: [ENUM_Auto_State."position claw arm lift" ("State") ENUM_Auto_State."Idle" ("State")] -> w2006
                  tunnel: [FALSE ("Switch Booleans.Arm In position") TRUE ("Switch Booleans.Arm In position")] -> w2005
                  tunnel: [w2013 w2017] -> w2004
                  frame False {
                    w2013 = T11[] [enum."Drive"] items=["No Action", "Reset Time", "Reset All", "Lock Angle", "Drive", "Zero Drive Encoders", "Zero YAW"] ("Actions")
                  }
                  frame True {
                    w2017 = T11[] [enum."No Action"] items=["No Action", "Reset Time", "Reset All", "Lock Angle", "Drive", "Zero Drive Encoders", "Zero YAW"] ("Actions")
                  }
                }
                n514 = Bundle By Name(cluster=w2009, "CMD_SM_Rotation.Rotation Positon"=w2007, "Switch Booleans.Arm In position"=w2005) -> (w2008:T12)
              }
              frame "Intake" {
                n515 = case shown="False" TRUE {
                  tunnel: [ENUM_Auto_State."Intake" ("State") ENUM_Auto_State."Idle" ("State")] -> w2022
                  tunnel: [w2025 w2027] -> w2023
                  frame False {
                    w2025 = T11[] [enum."Drive"] items=["No Action", "Reset Time", "Reset All", "Lock Angle", "Drive", "Zero Drive Encoders", "Zero YAW"] ("Actions")
                  }
                  frame True {
                    w2027 = T11[] [enum."No Action"] items=["No Action", "Reset Time", "Reset All", "Lock Angle", "Drive", "Zero Drive Encoders", "Zero YAW"] ("Actions")
                  }
                }
              }
              frame "Cross Line" {
                n516 = Unbundle By Name(w2049) -> ("Encoder Target Position(in)"=w2031:dbl, "Left Encoder"=w2040:i32, "Right Encoder"=w2039:i32, "Test"=w2051:dbl, "Switch Booleans.First Drive"=w2036:bool)
                n517 = call "EncoderPositionCalc.vi"("PositionTarget(in)"=w2031, "Wheel Size(in)"=6.0, "EncoderCount/Revolution"=4096.0) -> ("PostionTarget(Counts)"=w2038:i32)  [unwired: 8 in]
                n518 = call "AUTO_Encoder_In_Range_Check.vi"("Right Encoder"=w2039, "Left Encoder"=w2040, "PostionTarget(Counts)"=w2038) -> ("Boolean"=w2041:bool)  [unwired: 8 in]
                n519 = Greater?(x=w2051, y=0.5) -> (0:w2053:bool)
                n520 = case shown="False" w2041 {
                  tunnel: [ENUM_Auto_State."Cross Line" ("State") w2062] -> w2042
                  tunnel: w2036 -> [_ w2061]
                  tunnel: [w2057 w2060] -> w2035
                  tunnel: [w2057 w2059] -> w2034
                  frame False {
                    w2057 = FALSE
                  }
                  frame True {
                    n521 = case shown="False" w2061 {
                      tunnel: [ENUM_Auto_State."Idle" ("State") ENUM_Auto_State."Idle" ("State")] -> w2062
                      tunnel: [FALSE w2066] -> w2060
                      tunnel: [TRUE w2066] -> w2059
                      frame False {
                      }
                      frame True {
                        w2066 = TRUE
                      }
                    }
                  }
                }
                n522 = First Call?() -> (First Call?: T/F=w2044:bool)
                n523 = Select(t=w2042, s=w2053, f=ENUM_Auto_State."Idle" ("State")) -> (s? t:f=w2030:T10)
                n524 = Select(t=ENUM_Auto_Action."Drive" ("Action"), s=w2053, f=ENUM_Auto_Action."No Action" ("Action")) -> (s? t:f=w2052:T11)
                n525 = Bundle By Name(cluster=w2049, "Target Angle(Degree)"=0.0, "Steering"=0.0, "Encoder Target Position(in)"=w2031, "Zero Drive Encoders"=w2044, "Zero YAW"=w2044, "CMD_Drive_Data.Drive_Mode"=ENUM_WC_Drive_DriveMode."Motion Profile", "Switch Booleans.First Drive"=w2034, "Switch Booleans.Second Move"=w2035) -> (w2048:T12)
                n526 = Build Array(w2052, ENUM_Auto_Action."Zero Drive Encoders" ("Action"), ENUM_Auto_Action."Lock Angle" ("Action")) -> (w2029:T11[])
              }
              frame "Rotate To Angle" {
                w2079 = 3.0 ("y")
                w2075 = -90.0 ("Target Angle(Degree)")
                n527 = Unbundle By Name(w2088) -> ("YAW"=w2074:dbl, "Test"=w2090:dbl)
                n528 = Greater?(x=w2090, y=0.5) -> (0:w2092:bool)
                n529 = Add(x=w2075, y=w2079) -> (x+y=w2071:dbl)
                n530 = Subtract(x=w2075, y=w2079) -> (x-y=w2070:dbl)
                n531 = In Range and Coerce(upper limit=w2071, x=w2074, lower limit=w2070) -> (In Range?=w2076:bool)  [unwired: 1 out]
                n532 = Select(t=w2074, s=w2076, f=w2075) -> (s? t:f=w2077:dbl)
                n533 = case shown="True" w2076 {
                  tunnel: [ENUM_Auto_State."Rotate To Angle" ("State") ENUM_Auto_State."Idle" ("State")] -> w2081
                  tunnel: [FALSE ("Lock Angle") TRUE ("Lock Angle")] -> w2072
                  frame False {
                  }
                  frame True {
                  }
                }
                n534 = First Call?() -> (First Call?: T/F=w2085:bool)
                n535 = Select(t=w2081, s=w2092, f=ENUM_Auto_State."Idle" ("State")) -> (s? t:f=w2069:T10)
                n536 = Select(t=ENUM_Auto_Action."Drive" ("Action"), s=w2092, f=ENUM_Auto_Action."No Action" ("Action")) -> (s? t:f=w2091:T11)
                n537 = Bundle By Name(cluster=w2088, "Target Angle(Degree)"=w2077, "Steering"=0.0, "Encoder Target Position(in)"=0.0, "Zero Drive Encoders"=w2085, "Zero YAW"=w2085, "CMD_Drive_Data.Drive_Mode"=ENUM_WC_Drive_DriveMode."VBus", "Lock Angle"=TRUE, "Switch Booleans.Rotated"=w2072) -> (w2087:T12)
                n538 = Build Array(w2091, ENUM_Auto_Action."Zero Drive Encoders" ("Action"), ENUM_Auto_Action."Zero YAW" ("Action"), ENUM_Auto_Action."Lock Angle" ("Action")) -> (w2068:T11[])
              }
              frame "Shutdown" {
                w2100 = T11[] [enum."Reset All"] items=["No Action", "Reset Time", "Reset All", "Lock Angle", "Drive", "Zero Drive Encoders", "Zero YAW"] ("Actions")
              }
            }
          }
          frame "Scale" {
            n539 = case shown="\"Rotate To Angle\"" w2108 {
              tunnel: w2107 -> [w2113 w2119 w2170 w2185 w2210 w2249 w2264]
              tunnel: [w2113 w2118 w2169 w2185 w2209 w2248 w2264] -> w2110
              tunnel: w2109 -> [_ _ _ _ _ _ _]
              tunnel: [_ _ _ _ _ _ TRUE] -> w2106
              tunnel: [ENUM_Auto_State."Idle" ("State") w2114 w2167 w2183 w2191 w2230 ENUM_Auto_State."Shutdown" ("State")] -> w2104
              tunnel: [w2111 w2115 w2165 w2184 w2190 w2229 w2261] -> w2105
              frame "Startup" {
                w2111 = T11[] [enum."Reset All", enum."Reset Time"] items=["No Action", "Reset Time", "Reset All", "Lock Angle", "Drive", "Zero Drive Encoders", "Zero YAW"] ("Actions")
              }
              frame "Idle" {
                n540 = Unbundle By Name(w2119) -> ("Switch Booleans.First Drive"=w2124:bool, "Switch Booleans.Rotated"=w2123:bool, "Switch Booleans.Second Move"=w2122:bool, "Switch Booleans.Arm In position"=w2121:bool, "Switch Booleans.Cube released"=w2120:bool, "Test"=w2126:dbl)
                n541 = Less?(x=w2126, y=2.0) -> (x < y?=w2128:bool)
                n542 = case shown="True" w2124 {
                  tunnel: [ENUM_Auto_State."Cross Line" ("State") w2141] -> w2132
                  tunnel: w2123 -> [_ w2142]
                  tunnel: w2122 -> [_ w2140]
                  tunnel: w2121 -> [_ w2139]
                  tunnel: w2120 -> [_ w2138]
                  tunnel: [94.0 w2136] -> w2117
                  tunnel: [0.0 w2137] -> w2116
                  frame False {
                  }
                  frame True {
                    n543 = case shown="True" w2142 {
                      tunnel: [ENUM_Auto_State."Rotate To Angle" ("State") w2149] -> w2141
                      tunnel: w2140 -> [_ w2148]
                      tunnel: w2139 -> [_ w2150]
                      tunnel: w2138 -> [_ w2146]
                      tunnel: [90.0 0.0] -> w2137
                      tunnel: [0.0 w2147] -> w2136
                      frame False {
                      }
                      frame True {
                        n544 = case shown="False" w2150 {
                          tunnel: [ENUM_Auto_State."position claw arm lift" ("State") w2156] -> w2149
                          tunnel: w2148 -> [_ w2157]
                          tunnel: [0.0 w2155] -> w2147
                          tunnel: w2146 -> [_ w2154]
                          frame False {
                          }
                          frame True {
                            n545 = case shown="True" w2157 {
                              tunnel: [ENUM_Auto_State."Cross Line" ("State") w2161] -> w2156
                              tunnel: [32.0 0.0] -> w2155
                              tunnel: w2154 -> [_ w2160]
                              frame False {
                              }
                              frame True {
                                n546 = case shown="True" w2160 {
                                tunnel: [ENUM_Auto_State."Intake" ("State") ENUM_Auto_State."Shutdown" ("State")] -> w2161
                                frame False {
                                }
                                frame True {
                                }
                                }
                              }
                            }
                          }
                        }
                      }
                    }
                  }
                }
                n547 = Select(t=w2132, s=w2128, f=ENUM_Auto_State."Shutdown" ("State")) -> (s? t:f=w2114:T10)
                n548 = Select(t=ENUM_Auto_Action."Reset All" ("Action"), s=w2128, f=ENUM_Auto_Action."No Action" ("Action")) -> (s? t:f=w2127:T11)
                n549 = Bundle By Name(cluster=w2119, "Encoder Target Position(in)"=w2117, "Target Angle(Degree)"=w2116) -> (w2118:T12)
                n550 = Build Array(w2127) -> (w2115:T11[])
              }
              frame "position claw arm lift" {
                n551 = Unbundle By Name(w2170) -> ("SM_Rotation_Output"=w2173:T1)
                n552 = Equal?(x=w2173, y=ENUM_Rotation_Positon."Switch" ("CMD_SM_Rotation.Rotation Positon")) -> (x = y?=w2171:bool)
                n553 = case shown="True" w2171 {
                  tunnel: [ENUM_Rotation_Positon."Switch" ("CMD_SM_Rotation.Rotation Positon") ENUM_Rotation_Positon."Switch" ("CMD_SM_Rotation.Rotation Positon")] -> w2168
                  tunnel: [ENUM_Auto_State."position claw arm lift" ("State") ENUM_Auto_State."Idle" ("State")] -> w2167
                  tunnel: [FALSE ("Switch Booleans.Arm In position") TRUE ("Switch Booleans.Arm In position")] -> w2166
                  tunnel: [w2174 w2178] -> w2165
                  frame False {
                    w2174 = T11[] [enum."Drive"] items=["No Action", "Reset Time", "Reset All", "Lock Angle", "Drive", "Zero Drive Encoders", "Zero YAW"] ("Actions")
                  }
                  frame True {
                    w2178 = T11[] [enum."No Action"] items=["No Action", "Reset Time", "Reset All", "Lock Angle", "Drive", "Zero Drive Encoders", "Zero YAW"] ("Actions")
                  }
                }
                n554 = Bundle By Name(cluster=w2170, "CMD_SM_Rotation.Rotation Positon"=w2168, "Switch Booleans.Arm In position"=w2166) -> (w2169:T12)
              }
              frame "Intake" {
                n555 = case shown="False" TRUE {
                  tunnel: [ENUM_Auto_State."Intake" ("State") ENUM_Auto_State."Idle" ("State")] -> w2183
                  tunnel: [w2186 w2188] -> w2184
                  frame False {
                    w2186 = T11[] [enum."Drive"] items=["No Action", "Reset Time", "Reset All", "Lock Angle", "Drive", "Zero Drive Encoders", "Zero YAW"] ("Actions")
                  }
                  frame True {
                    w2188 = T11[] [enum."No Action"] items=["No Action", "Reset Time", "Reset All", "Lock Angle", "Drive", "Zero Drive Encoders", "Zero YAW"] ("Actions")
                  }
                }
              }
              frame "Cross Line" {
                n556 = Unbundle By Name(w2210) -> ("Encoder Target Position(in)"=w2192:dbl, "Left Encoder"=w2201:i32, "Right Encoder"=w2200:i32, "Test"=w2212:dbl, "Switch Booleans.First Drive"=w2197:bool)
                n557 = call "EncoderPositionCalc.vi"("PositionTarget(in)"=w2192, "Wheel Size(in)"=6.0, "EncoderCount/Revolution"=4096.0) -> ("PostionTarget(Counts)"=w2199:i32)  [unwired: 8 in]
                n558 = call "AUTO_Encoder_In_Range_Check.vi"("Right Encoder"=w2200, "Left Encoder"=w2201, "PostionTarget(Counts)"=w2199) -> ("Boolean"=w2202:bool)  [unwired: 8 in]
                n559 = Greater?(x=w2212, y=0.5) -> (0:w2214:bool)
                n560 = case shown="False" w2202 {
                  tunnel: [ENUM_Auto_State."Cross Line" ("State") w2223] -> w2203
                  tunnel: w2197 -> [_ w2222]
                  tunnel: [w2218 w2221] -> w2196
                  tunnel: [w2218 w2220] -> w2195
                  frame False {
                    w2218 = FALSE
                  }
                  frame True {
                    n561 = case shown="False" w2222 {
                      tunnel: [ENUM_Auto_State."Idle" ("State") ENUM_Auto_State."Idle" ("State")] -> w2223
                      tunnel: [FALSE w2227] -> w2221
                      tunnel: [TRUE w2227] -> w2220
                      frame False {
                      }
                      frame True {
                        w2227 = TRUE
                      }
                    }
                  }
                }
                n562 = First Call?() -> (First Call?: T/F=w2205:bool)
                n563 = Select(t=w2203, s=w2214, f=ENUM_Auto_State."Idle" ("State")) -> (s? t:f=w2191:T10)
                n564 = Select(t=ENUM_Auto_Action."Drive" ("Action"), s=w2214, f=ENUM_Auto_Action."No Action" ("Action")) -> (s? t:f=w2213:T11)
                n565 = Bundle By Name(cluster=w2210, "Target Angle(Degree)"=0.0, "Steering"=0.0, "Encoder Target Position(in)"=w2192, "Zero Drive Encoders"=w2205, "Zero YAW"=w2205, "CMD_Drive_Data.Drive_Mode"=ENUM_WC_Drive_DriveMode."Motion Profile", "Switch Booleans.First Drive"=w2195, "Switch Booleans.Second Move"=w2196) -> (w2209:T12)
                n566 = Build Array(w2213, ENUM_Auto_Action."Zero Drive Encoders" ("Action"), ENUM_Auto_Action."Lock Angle" ("Action")) -> (w2190:T11[])
              }
              frame "Rotate To Angle" {
                w2240 = 3.0 ("y")
                w2236 = -90.0 ("Target Angle(Degree)")
                n567 = Unbundle By Name(w2249) -> ("YAW"=w2235:dbl, "Test"=w2251:dbl)
                n568 = Greater?(x=w2251, y=0.5) -> (0:w2253:bool)
                n569 = Add(x=w2236, y=w2240) -> (x+y=w2232:dbl)
                n570 = Subtract(x=w2236, y=w2240) -> (x-y=w2231:dbl)
                n571 = In Range and Coerce(upper limit=w2232, x=w2235, lower limit=w2231) -> (In Range?=w2237:bool)  [unwired: 1 out]
                n572 = Select(t=w2235, s=w2237, f=w2236) -> (s? t:f=w2238:dbl)
                n573 = case shown="True" w2237 {
                  tunnel: [ENUM_Auto_State."Rotate To Angle" ("State") ENUM_Auto_State."Idle" ("State")] -> w2242
                  tunnel: [FALSE ("Lock Angle") TRUE ("Lock Angle")] -> w2233
                  frame False {
                  }
                  frame True {
                  }
                }
                n574 = First Call?() -> (First Call?: T/F=w2246:bool)
                n575 = Select(t=w2242, s=w2253, f=ENUM_Auto_State."Idle" ("State")) -> (s? t:f=w2230:T10)
                n576 = Select(t=ENUM_Auto_Action."Drive" ("Action"), s=w2253, f=ENUM_Auto_Action."No Action" ("Action")) -> (s? t:f=w2252:T11)
                n577 = Bundle By Name(cluster=w2249, "Target Angle(Degree)"=w2238, "Steering"=0.0, "Encoder Target Position(in)"=0.0, "Zero Drive Encoders"=w2246, "Zero YAW"=w2246, "CMD_Drive_Data.Drive_Mode"=ENUM_WC_Drive_DriveMode."VBus", "Lock Angle"=TRUE, "Switch Booleans.Rotated"=w2233) -> (w2248:T12)
                n578 = Build Array(w2252, ENUM_Auto_Action."Zero Drive Encoders" ("Action"), ENUM_Auto_Action."Zero YAW" ("Action"), ENUM_Auto_Action."Lock Angle" ("Action")) -> (w2229:T11[])
              }
              frame "Shutdown" {
                w2261 = T11[] [enum."Reset All"] items=["No Action", "Reset Time", "Reset All", "Lock Angle", "Drive", "Zero Drive Encoders", "Zero YAW"] ("Actions")
              }
            }
          }
          frame "Scale And Switch" {
            n579 = case shown="\"Rotate To Angle\"" w2269 {
              tunnel: w2268 -> [w2274 w2280 w2331 w2346 w2371 w2410 w2425]
              tunnel: [w2274 w2279 w2330 w2346 w2370 w2409 w2425] -> w2271
              tunnel: w2270 -> [_ _ _ _ _ _ _]
              tunnel: [_ _ _ _ _ _ TRUE] -> w2267
              tunnel: [ENUM_Auto_State."Idle" ("State") w2275 w2328 w2344 w2352 w2391 ENUM_Auto_State."Shutdown" ("State")] -> w2265
              tunnel: [w2272 w2276 w2326 w2345 w2351 w2390 w2422] -> w2266
              frame "Startup" {
                w2272 = T11[] [enum."Reset All", enum."Reset Time"] items=["No Action", "Reset Time", "Reset All", "Lock Angle", "Drive", "Zero Drive Encoders", "Zero YAW"] ("Actions")
              }
              frame "Idle" {
                n580 = Unbundle By Name(w2280) -> ("Switch Booleans.First Drive"=w2285:bool, "Switch Booleans.Rotated"=w2284:bool, "Switch Booleans.Second Move"=w2283:bool, "Switch Booleans.Arm In position"=w2282:bool, "Switch Booleans.Cube released"=w2281:bool, "Test"=w2287:dbl)
                n581 = Less?(x=w2287, y=2.0) -> (x < y?=w2289:bool)
                n582 = case shown="True" w2285 {
                  tunnel: [ENUM_Auto_State."Cross Line" ("State") w2302] -> w2293
                  tunnel: w2284 -> [_ w2303]
                  tunnel: w2283 -> [_ w2301]
                  tunnel: w2282 -> [_ w2300]
                  tunnel: w2281 -> [_ w2299]
                  tunnel: [94.0 w2297] -> w2278
                  tunnel: [0.0 w2298] -> w2277
                  frame False {
                  }
                  frame True {
                    n583 = case shown="True" w2303 {
                      tunnel: [ENUM_Auto_State."Rotate To Angle" ("State") w2310] -> w2302
                      tunnel: w2301 -> [_ w2309]
                      tunnel: w2300 -> [_ w2311]
                      tunnel: w2299 -> [_ w2307]
                      tunnel: [90.0 0.0] -> w2298
                      tunnel: [0.0 w2308] -> w2297
                      frame False {
                      }
                      frame True {
                        n584 = case shown="False" w2311 {
                          tunnel: [ENUM_Auto_State."position claw arm lift" ("State") w2317] -> w2310
                          tunnel: w2309 -> [_ w2318]
                          tunnel: [0.0 w2316] -> w2308
                          tunnel: w2307 -> [_ w2315]
                          frame False {
                          }
                          frame True {
                            n585 = case shown="True" w2318 {
                              tunnel: [ENUM_Auto_State."Cross Line" ("State") w2322] -> w2317
                              tunnel: [32.0 0.0] -> w2316
                              tunnel: w2315 -> [_ w2321]
                              frame False {
                              }
                              frame True {
                                n586 = case shown="True" w2321 {
                                tunnel: [ENUM_Auto_State."Intake" ("State") ENUM_Auto_State."Shutdown" ("State")] -> w2322
                                frame False {
                                }
                                frame True {
                                }
                                }
                              }
                            }
                          }
                        }
                      }
                    }
                  }
                }
                n587 = Select(t=w2293, s=w2289, f=ENUM_Auto_State."Shutdown" ("State")) -> (s? t:f=w2275:T10)
                n588 = Select(t=ENUM_Auto_Action."Reset All" ("Action"), s=w2289, f=ENUM_Auto_Action."No Action" ("Action")) -> (s? t:f=w2288:T11)
                n589 = Bundle By Name(cluster=w2280, "Encoder Target Position(in)"=w2278, "Target Angle(Degree)"=w2277) -> (w2279:T12)
                n590 = Build Array(w2288) -> (w2276:T11[])
              }
              frame "position claw arm lift" {
                n591 = Unbundle By Name(w2331) -> ("SM_Rotation_Output"=w2334:T1)
                n592 = Equal?(x=w2334, y=ENUM_Rotation_Positon."Switch" ("CMD_SM_Rotation.Rotation Positon")) -> (x = y?=w2332:bool)
                n593 = case shown="True" w2332 {
                  tunnel: [ENUM_Rotation_Positon."Switch" ("CMD_SM_Rotation.Rotation Positon") ENUM_Rotation_Positon."Switch" ("CMD_SM_Rotation.Rotation Positon")] -> w2329
                  tunnel: [ENUM_Auto_State."position claw arm lift" ("State") ENUM_Auto_State."Idle" ("State")] -> w2328
                  tunnel: [FALSE ("Switch Booleans.Arm In position") TRUE ("Switch Booleans.Arm In position")] -> w2327
                  tunnel: [w2335 w2339] -> w2326
                  frame False {
                    w2335 = T11[] [enum."Drive"] items=["No Action", "Reset Time", "Reset All", "Lock Angle", "Drive", "Zero Drive Encoders", "Zero YAW"] ("Actions")
                  }
                  frame True {
                    w2339 = T11[] [enum."No Action"] items=["No Action", "Reset Time", "Reset All", "Lock Angle", "Drive", "Zero Drive Encoders", "Zero YAW"] ("Actions")
                  }
                }
                n594 = Bundle By Name(cluster=w2331, "CMD_SM_Rotation.Rotation Positon"=w2329, "Switch Booleans.Arm In position"=w2327) -> (w2330:T12)
              }
              frame "Intake" {
                n595 = case shown="False" TRUE {
                  tunnel: [ENUM_Auto_State."Intake" ("State") ENUM_Auto_State."Idle" ("State")] -> w2344
                  tunnel: [w2347 w2349] -> w2345
                  frame False {
                    w2347 = T11[] [enum."Drive"] items=["No Action", "Reset Time", "Reset All", "Lock Angle", "Drive", "Zero Drive Encoders", "Zero YAW"] ("Actions")
                  }
                  frame True {
                    w2349 = T11[] [enum."No Action"] items=["No Action", "Reset Time", "Reset All", "Lock Angle", "Drive", "Zero Drive Encoders", "Zero YAW"] ("Actions")
                  }
                }
              }
              frame "Cross Line" {
                n596 = Unbundle By Name(w2371) -> ("Encoder Target Position(in)"=w2353:dbl, "Left Encoder"=w2362:i32, "Right Encoder"=w2361:i32, "Test"=w2373:dbl, "Switch Booleans.First Drive"=w2358:bool)
                n597 = call "EncoderPositionCalc.vi"("PositionTarget(in)"=w2353, "Wheel Size(in)"=6.0, "EncoderCount/Revolution"=4096.0) -> ("PostionTarget(Counts)"=w2360:i32)  [unwired: 8 in]
                n598 = call "AUTO_Encoder_In_Range_Check.vi"("Right Encoder"=w2361, "Left Encoder"=w2362, "PostionTarget(Counts)"=w2360) -> ("Boolean"=w2363:bool)  [unwired: 8 in]
                n599 = Greater?(x=w2373, y=0.5) -> (0:w2375:bool)
                n600 = case shown="False" w2363 {
                  tunnel: [ENUM_Auto_State."Cross Line" ("State") w2384] -> w2364
                  tunnel: w2358 -> [_ w2383]
                  tunnel: [w2379 w2382] -> w2357
                  tunnel: [w2379 w2381] -> w2356
                  frame False {
                    w2379 = FALSE
                  }
                  frame True {
                    n601 = case shown="False" w2383 {
                      tunnel: [ENUM_Auto_State."Idle" ("State") ENUM_Auto_State."Idle" ("State")] -> w2384
                      tunnel: [FALSE w2388] -> w2382
                      tunnel: [TRUE w2388] -> w2381
                      frame False {
                      }
                      frame True {
                        w2388 = TRUE
                      }
                    }
                  }
                }
                n602 = First Call?() -> (First Call?: T/F=w2366:bool)
                n603 = Select(t=w2364, s=w2375, f=ENUM_Auto_State."Idle" ("State")) -> (s? t:f=w2352:T10)
                n604 = Select(t=ENUM_Auto_Action."Drive" ("Action"), s=w2375, f=ENUM_Auto_Action."No Action" ("Action")) -> (s? t:f=w2374:T11)
                n605 = Bundle By Name(cluster=w2371, "Target Angle(Degree)"=0.0, "Steering"=0.0, "Encoder Target Position(in)"=w2353, "Zero Drive Encoders"=w2366, "Zero YAW"=w2366, "CMD_Drive_Data.Drive_Mode"=ENUM_WC_Drive_DriveMode."Motion Profile", "Switch Booleans.First Drive"=w2356, "Switch Booleans.Second Move"=w2357) -> (w2370:T12)
                n606 = Build Array(w2374, ENUM_Auto_Action."Zero Drive Encoders" ("Action"), ENUM_Auto_Action."Lock Angle" ("Action")) -> (w2351:T11[])
              }
              frame "Rotate To Angle" {
                w2401 = 3.0 ("y")
                w2397 = -90.0 ("Target Angle(Degree)")
                n607 = Unbundle By Name(w2410) -> ("YAW"=w2396:dbl, "Test"=w2412:dbl)
                n608 = Greater?(x=w2412, y=0.5) -> (0:w2414:bool)
                n609 = Add(x=w2397, y=w2401) -> (x+y=w2393:dbl)
                n610 = Subtract(x=w2397, y=w2401) -> (x-y=w2392:dbl)
                n611 = In Range and Coerce(upper limit=w2393, x=w2396, lower limit=w2392) -> (In Range?=w2398:bool)  [unwired: 1 out]
                n612 = Select(t=w2396, s=w2398, f=w2397) -> (s? t:f=w2399:dbl)
                n613 = case shown="True" w2398 {
                  tunnel: [ENUM_Auto_State."Rotate To Angle" ("State") ENUM_Auto_State."Idle" ("State")] -> w2403
                  tunnel: [FALSE ("Lock Angle") TRUE ("Lock Angle")] -> w2394
                  frame False {
                  }
                  frame True {
                  }
                }
                n614 = First Call?() -> (First Call?: T/F=w2407:bool)
                n615 = Select(t=w2403, s=w2414, f=ENUM_Auto_State."Idle" ("State")) -> (s? t:f=w2391:T10)
                n616 = Select(t=ENUM_Auto_Action."Drive" ("Action"), s=w2414, f=ENUM_Auto_Action."No Action" ("Action")) -> (s? t:f=w2413:T11)
                n617 = Bundle By Name(cluster=w2410, "Target Angle(Degree)"=w2399, "Steering"=0.0, "Encoder Target Position(in)"=0.0, "Zero Drive Encoders"=w2407, "Zero YAW"=w2407, "CMD_Drive_Data.Drive_Mode"=ENUM_WC_Drive_DriveMode."VBus", "Lock Angle"=TRUE, "Switch Booleans.Rotated"=w2394) -> (w2409:T12)
                n618 = Build Array(w2413, ENUM_Auto_Action."Zero Drive Encoders" ("Action"), ENUM_Auto_Action."Zero YAW" ("Action"), ENUM_Auto_Action."Lock Angle" ("Action")) -> (w2390:T11[])
              }
              frame "Shutdown" {
                w2422 = T11[] [enum."Reset All"] items=["No Action", "Reset Time", "Reset All", "Lock Angle", "Drive", "Zero Drive Encoders", "Zero YAW"] ("Actions")
              }
            }
          }
          frame "Cross Line" {
            n619 = case shown="\"Rotate To Angle\"" w2429 {
              tunnel: w2428 -> [w2435 w2438 w2466 w2480 w2483 w2501 w2516]
              tunnel: [w2435 w2437 w2465 w2480 w2483 w2500 w2516] -> w2432
              tunnel: [ENUM_Auto_State."Idle" ("State") w2448 w2475 ENUM_Auto_State."Shutdown" ("State") ENUM_Auto_State."Shutdown" ("State") w2510 ENUM_Auto_State."Shutdown" ("State")] -> w2431
              tunnel: [w2434 w2441 w2469 w2479 w2482 w2504 w2514] -> w2427
              tunnel: w2430 -> [_ _ _ _ _ _ _]
              tunnel: [_ _ _ _ _ _ TRUE] -> w2426
              frame "Startup" {
                w2434 = T11[] [enum."Reset All", enum."Reset Time"] items=["No Action", "Reset Time", "Reset All", "Lock Angle", "Drive", "Zero Drive Encoders", "Zero YAW"] ("Actions")
              }
              frame "Idle" {
                n620 = Unbundle By Name(w2438) -> ("Test"=w2440:dbl)
                n621 = Less?(x=w2440, y=2.0) -> (x < y?=w2443:bool)
                n622 = Select(t=ENUM_Auto_State."Cross Line" ("State"), s=w2443, f=ENUM_Auto_State."Shutdown" ("State")) -> (s? t:f=w2448:T10)
                n623 = Select(t=ENUM_Auto_Action."Reset All" ("Action"), s=w2443, f=ENUM_Auto_Action."No Action" ("Action")) -> (s? t:f=w2442:T11)
                n624 = Build Array(w2442) -> (w2441:T11[])
                n625 = Bundle By Name(cluster=w2438, "Encoder Target Position(in)"=120.0) -> (w2437:T12)
              }
              frame "Cross Line" {
                w2451 = 120.0 ("Encoder Target Position(in)")
                n626 = Unbundle By Name(w2466) -> ("Zero YAW"=w2457:bool, "Left Encoder"=w2455:i32, "Right Encoder"=w2454:i32, "Test"=w2468:dbl)
                n627 = Greater?(x=w2468, y=0.5) -> (0:w2471:bool)
                n628 = call "EncoderPositionCalc.vi"("PositionTarget(in)"=4092.0, "Wheel Size(in)"=6.0, "EncoderCount/Revolution"=w2451) -> ("PostionTarget(Counts)"=w2452:i32)  [unwired: 8 in]
                n629 = call "AUTO_Encoder_In_Range_Check.vi"("Right Encoder"=w2454, "Left Encoder"=w2455, "PostionTarget(Counts)"=w2452) -> ("Boolean"=w2453:bool)  [unwired: 8 in]
                n630 = case shown="True" w2453 {
                  tunnel: [ENUM_Auto_State."Cross Line" ("State") ENUM_Auto_State."Shutdown" ("State")] -> w2456
                  frame False {
                  }
                  frame True {
                  }
                }
                n631 = First Call?() -> (First Call?: T/F=w2458:bool)
                n632 = Select(t=w2456, s=w2471, f=ENUM_Auto_State."Idle" ("State")) -> (s? t:f=w2475:T10)
                n633 = Select(t=ENUM_Auto_Action."Drive" ("Action"), s=w2471, f=ENUM_Auto_Action."No Action" ("Action")) -> (s? t:f=w2470:T11)
                n634 = Bundle By Name(cluster=w2466, "Target Angle(Degree)"=0.0, "Steering"=0.0, "Encoder Target Position(in)"=w2451, "Zero Drive Encoders"=w2458, "Zero YAW"=w2457, "CMD_Drive_Data.Drive_Mode"=ENUM_WC_Drive_DriveMode."Motion Profile") -> (w2465:T12)
                n635 = Build Array(w2470, ENUM_Auto_Action."Zero Drive Encoders" ("Action"), ENUM_Auto_Action."Zero YAW" ("Action"), ENUM_Auto_Action."Lock Angle" ("Action")) -> (w2469:T11[])
              }
              frame "position claw arm lift" {
                w2479 = T11[] [enum."No Action"] items=["No Action", "Reset Time", "Reset All", "Lock Angle", "Drive", "Zero Drive Encoders", "Zero YAW"] ("Actions")
              }
              frame "Intake" {
                w2482 = T11[] [enum."No Action"] items=["No Action", "Reset Time", "Reset All", "Lock Angle", "Drive", "Zero Drive Encoders", "Zero YAW"] ("Actions")
              }
              frame "Rotate To Angle" {
                w2489 = 3.0 ("y")
                w2485 = 180.0 ("Target Angle(Degree)")
                n636 = Unbundle By Name(w2501) -> ("YAW"=w2484:dbl, "Test"=w2503:dbl)
                n637 = Greater?(x=w2503, y=0.5) -> (0:w2506:bool)
                n638 = Add(x=w2485, y=w2489) -> (x+y=w2491:dbl)
                n639 = Subtract(x=w2485, y=w2489) -> (x-y=w2490:dbl)
                n640 = In Range and Coerce(upper limit=w2491, x=w2484, lower limit=w2490) -> (In Range?=w2486:bool)  [unwired: 1 out]
                n641 = Select(t=w2484, s=w2486, f=w2485) -> (s? t:f=w2487:dbl)
                n642 = case shown="False" w2486 {
                  tunnel: [ENUM_Auto_State."Cross Line" ("State") ENUM_Auto_State."Cross Line" ("State")] -> w2493
                  frame False {
                  }
                  frame True {
                  }
                }
                n643 = First Call?() -> (First Call?: T/F=w2497:bool)
                n644 = Select(t=w2493, s=w2506, f=ENUM_Auto_State."Idle" ("State")) -> (s? t:f=w2510:T10)
                n645 = Select(t=ENUM_Auto_Action."Drive" ("Action"), s=w2506, f=ENUM_Auto_Action."No Action" ("Action")) -> (s? t:f=w2505:T11)
                n646 = Bundle By Name(cluster=w2501, "Target Angle(Degree)"=w2487, "Steering"=0.0, "Encoder Target Position(in)"=0.0, "Zero Drive Encoders"=w2497, "Zero YAW"=w2497, "CMD_Drive_Data.Drive_Mode"=ENUM_WC_Drive_DriveMode."VBus", "Lock Angle"=TRUE) -> (w2500:T12)
                n647 = Build Array(w2505, ENUM_Auto_Action."Zero Drive Encoders" ("Action"), ENUM_Auto_Action."Zero YAW" ("Action"), ENUM_Auto_Action."Lock Angle" ("Action")) -> (w2504:T11[])
              }
              frame "Shutdown" {
                w2514 = T11[] [enum."Reset All"] items=["No Action", "Reset Time", "Reset All", "Lock Angle", "Drive", "Zero Drive Encoders", "Zero YAW"] ("Actions")
              }
            }
          }
          frame "No Movement" {
            n648 = case shown="\"Rotate To Angle\"" w2520 {
              tunnel: w2519 -> [w2526 w2529 w2542 w2545 w2548 w2551 w2555]
              tunnel: [w2526 w2528 w2542 w2545 w2548 w2551 w2555] -> w2523
              tunnel: [ENUM_Auto_State."Idle" ("State") w2539 ENUM_Auto_State."Shutdown" ("State") ENUM_Auto_State."Idle" ("State") ENUM_Auto_State."Idle" ("State") ENUM_Auto_State."Idle" ("State") ENUM_Auto_State."Shutdown" ("State")] -> w2522
              tunnel: [w2525 w2532 w2541 w2543 w2546 w2549 w2553] -> w2518
              tunnel: w2521 -> [_ _ _ _ _ _ _]
              tunnel: [_ _ _ _ _ _ TRUE] -> w2517
              frame "Startup" {
                w2525 = T11[] [enum."Reset All", enum."Reset Time"] items=["No Action", "Reset Time", "Reset All", "Lock Angle", "Drive", "Zero Drive Encoders", "Zero YAW"] ("Actions")
              }
              frame "Idle" {
                n649 = Unbundle By Name(w2529) -> ("Test"=w2531:dbl)
                n650 = Less?(x=w2531, y=2.0) -> (x < y?=w2534:bool)
                n651 = Select(t=ENUM_Auto_State."Idle" ("State"), s=w2534, f=ENUM_Auto_State."Shutdown" ("State")) -> (s? t:f=w2539:T10)
                n652 = Select(t=ENUM_Auto_Action."Reset All" ("Action"), s=w2534, f=ENUM_Auto_Action."No Action" ("Action")) -> (s? t:f=w2533:T11)
                n653 = Build Array(w2533) -> (w2532:T11[])
                n654 = Bundle By Name(cluster=w2529, "Encoder Target Position(in)"=120.0) -> (w2528:T12)
              }
              frame "position claw arm lift" {
                w2541 = T11[] [enum."No Action"] items=["No Action", "Reset Time", "Reset All", "Lock Angle", "Drive", "Zero Drive Encoders", "Zero YAW"] ("Actions")
              }
              frame "Cross Line" {
                w2543 = T11[] [enum."No Action"] items=["No Action", "Reset Time", "Reset All", "Lock Angle", "Drive", "Zero Drive Encoders", "Zero YAW"] ("Actions")
              }
              frame "Intake" {
                w2546 = T11[] [enum."No Action"] items=["No Action", "Reset Time", "Reset All", "Lock Angle", "Drive", "Zero Drive Encoders", "Zero YAW"] ("Actions")
              }
              frame "Rotate To Angle" {
                w2549 = T11[] [enum."No Action"] items=["No Action", "Reset Time", "Reset All", "Lock Angle", "Drive", "Zero Drive Encoders", "Zero YAW"] ("Actions")
              }
              frame "Shutdown" {
                w2553 = T11[] [enum."Reset All"] items=["No Action", "Reset Time", "Reset All", "Lock Angle", "Drive", "Zero Drive Encoders", "Zero YAW"] ("Actions")
              }
            }
          }
        }
        n655 = Bundle By Name(cluster=w1941, "Previous State"=w1938, "State"=w1940) -> (w1942:T12)
      }
    }
    n656 = for {
      tunnel: w39 -> [w2558] mode=indexing
      shift-right: [w2557] -> w46
      shift-left: w55 -> [w2556]
      n657 = case shown="\"Drive\"" w2558 {
        tunnel: w2556 -> [w2559 w2562 w2566 w2572 w2575 w2578 w2581]
        tunnel: [w2559 w2561 w2565 w2571 w2574 w2577 w2580] -> w2557
        frame "No Action" {
        }
        frame "Reset Time" {
          # "Reset timer by taking the current time\nand making it the start time\n\nLater when the current time is \nsubtracted from the start time\nyou will get the elapsed time in \nseconds"
          n658 = Unbundle By Name(w2562) -> ("Current Time"=w2560:timestamp)
          n659 = Bundle By Name(cluster=w2562, "Start Time"=w2560) -> (w2561:T12)
        }
        frame "Reset All" {
          w2564 = 0.0 ("FG Write Value")
          n660 = Bundle By Name(cluster=w2566, "CMD_Drive_Data.VBus.Drive.Steer"=w2564, "CMD_Drive_Data.VBus.Drive.Throtle"=w2564, "CMD_Drive_Data.Set Target Position(IN)"=w2564, "CMD_Drive_Data.Zero Drive Encoders"=TRUE ("Output Bool")) -> (w2565:T12)
        }
        frame "Drive" {
          n661 = Unbundle By Name(w2572) -> ("Throtal"=w2568:dbl, "Steering"=w2567:dbl, "Encoder Target Position(in)"=w2570:dbl, "Target Angle(Degree)"=w2569:dbl)
          n662 = Bundle By Name(cluster=w2572, "CMD_Drive_Data.VBus.Drive.Throtle"=w2568, "CMD_Drive_Data.VBus.Drive.Steer"=w2567, "CMD_Drive_Data.Set Target Position(IN)"=w2570, "CMD_Drive_Data.Target Angle(Degree)"=w2569) -> (w2571:T12)
        }
        frame "Zero Drive Encoders" {
          n663 = Unbundle By Name(w2575) -> ("Zero Drive Encoders"=w2573:bool)
          n664 = Bundle By Name(cluster=w2575, "CMD_Drive_Data.Zero Drive Encoders"=w2573) -> (w2574:T12)
        }
        frame "Zero YAW" {
          n665 = Unbundle By Name(w2578) -> ("Zero YAW"=w2576:bool)
          n666 = Bundle By Name(cluster=w2578, "CMD_Drive_Data.Zero YAW"=w2576) -> (w2577:T12)
        }
        frame "Lock Angle" {
          n667 = Unbundle By Name(w2581) -> ("Lock Angle"=w2579:bool)
          n668 = Bundle By Name(cluster=w2581, "CMD_Drive_Data.Lock Angle"=w2579) -> (w2580:T12)
        }
      }
    }
    n669 = Unbundle By Name(w46) -> ("CMD_Drive_Data"=w37:T5, "CMD_SM_Rotation"=w26:T2)
    n670 = Unbundle By Name(w46) -> ("Cycle Time(S)"=→"Cycle Time (S)":dbl)
    n671 = global write "Global_CMD.vi" "CMD_SM_Rotation"(w26) -> ()
    n672 = global write "Global_CMD_Drive.vi" "CMD_Drive_Data"(w37) -> ()
  }
